vi "EC_Applied_XYZ_MM_BR_RES_2_NC_GR_pxi_Acc3_preset_LIM2.vi"() -> ()   [LabVIEW 2009]
uses:
  <vilib>/Utility/file.llb/Read From Spreadsheet File (I64).vi
  <vilib>/Utility/file.llb/Read From Spreadsheet File (string).vi
  <vilib>/Instr/_visa.llb/VISA Configure Serial Port (Instr).vi
  <vilib>/Utility/file.llb/Write To Spreadsheet File (I64).vi
  <vilib>/Utility/file.llb/Write To Spreadsheet File (string).vi
panel:
  out "R Velocity MVdeg/sec":dbl format="%.3f"
  out "R Position MV deg":dbl
  out "Z Velocity MV mm/sec":dbl format="%.3f"
  out "Z Position MV mm":dbl
  out "Y Velocity MV mm/sec":dbl format="%.3f"
  out "Y Position MV mm":dbl
  out "X Velocity MV mm/sec":dbl format="%.3f"
  out "X Position MV mm":dbl
  out "Presets":i32[][](array[numeric])
  in  "stop":bool
  in  "Tab Control 3":enum32{"Status", "Reset"}(tab)
  out "Y in Range":bool
  out "Y Scan":bool
  out "Y in Motion":bool
  out "Y Backlash corr":bool
  out "X  in Range":bool
  out "X Scan":bool
  out "X  in Motion":bool
  out "X Backlash corr":bool
  out "Z in Range":bool
  out "Z Scan":bool
  out "Z in Motion":bool
  out "Z Backlash corr":bool
  out "R in Range":bool
  out "R Scan":bool
  out "R in Motion":bool
  out "R Backlash corr":bool
  out "X Ready":bool
  out "Y Ready":bool
  out "Z Ready":bool
  out "R Ready":bool
  in  "Reset Y Position mm":dbl
  out "Reset Y Motor Steps":i32
  in  "Reset X Position mm":dbl
  out "Reset X Motor Steps":i32
  in  "Reset Z Position mm":dbl
  out "Reset Z Motor Steps":i32
  in  "Reset R Position deg":dbl
  out "Reset R Motor Steps":i32
  in  "Reset":bool
  in  "Tab Control 2":enum32{"mm", "step"}(tab)
  in  "X Scan Length SP mm":dbl
  in  "X Scan Velocity SP mm/sec":dbl
  in  "X Scan set":bool
  in  "Y Scan Length SP mm":dbl
  in  "Y Scan Velocity SP mm/sec":dbl
  in  "Y Scan set":bool
  in  "Z Scan Length SP mm":dbl
  in  "Z Scan Velocity SP mm/sec":dbl
  in  "Z Scan set":bool
  in  "R Scan Length SP deg":dbl
  in  "R Scan Velocity SP deg/sec":dbl
  in  "R Scan set":bool
  in  "X Scan Velocity SP steps/sec":i32=1 min=1 max=102400 step=1
  in  "X Scan Length SP steps":i32 min=-500000 max=500000 step=100
  out "X Scan length MV mm":dbl
  out "X Scan velocity MV mm/sec":dbl format="%#_6f"
  in  "Y Scan Velocity SP steps/sec":i32=1 min=1 max=102400 step=1
  in  "Y Scan Length SP steps":i32 min=-1000000 max=0 step=100
  out "Y Scan length MV mm":dbl
  out "Y Scan velocity MV mm/sec":dbl format="%#_6f"
  in  "Z Scan Velocity SP steps/sec":i32=1 min=1 max=102400 step=1
  in  "Z Scan Length SP steps":i32 min=-204724 max=102195276 step=100
  out "Z Scan length MV mm":dbl
  out "Z Scan velocity MV mm/sec":dbl format="%#_6f"
  in  "R Scan Velocity SP steps/sec":i32=1 min=1 max=102400 step=1
  in  "R Scan Length SP steps":i32 min=-6144000 max=0 step=100
  out "R Scan length MV deg":dbl
  out "R Scan velocity MV deg/sec":dbl format="%#_6f"
  out "atan Y/Z":dbl
  in  "Tab Control":enum32{"mm", "preset", "step"}(tab)
  in  "X Position SP mm":dbl
  in  "X Velocity SP mm/sec":dbl
  in  "X Move Set":bool
  in  "Y Move Set":bool
  in  "Y Position SP mm":dbl
  in  "Y Velocity SP mm/sec":dbl
  in  "Z Position SP mm":dbl
  in  "Z Velocity SP mm/sec":dbl
  in  "Z Move Set":bool
  in  "R Position SP deg":dbl
  in  "R Velocity SP deg/sec":dbl
  in  "R Move Set":bool
  in  "Add Button":bool
  in  "String":string
  in  "Delete Button":bool
  in  "Preset positions":i32(ring) items=["ZERO", "Default", "CDOSE", "QMS", "test", "test2", "test3"]
  in  "Set Button":bool
  in  "X Velocity SP step/sec":i32 min=1 max=50000
  in  "Y Velocity SP step/sec":i32 min=1 max=50000
  in  "Z Velocity SP step/sec":i32 min=1 max=5000
  in  "R Velocity SP step/sec":i32 min=1 max=10000
  in  "Y Step SP":i32=-20000 min=-800000 max=800000 step=500
  in  "X Step SP":i32=-20000 min=-800000 max=800000 step=500
  in  "Z Step SP":i32=-20000 min=0 max=102400000 step=500
  in  "R Step SP":i32=-20000 min=-6144000 max=0 step=500
  out "X Step PV":i32 max=2000
  out "Y Step PV":i32 max=2000
  out "Z Step PV":i32 max=2000
  out "R Step PV":i32 max=2000
  in  "Clear ZY":bool
  out "ZY Graph":cluster{"Y":dbl[], "Y":dbl[]}[](graph)
  out "ZR Graph":cluster{"Y":dbl[], "Y":dbl[]}[](graph)
  out "XY Graph":cluster{"Y":dbl[], "Y":dbl[]}[](graph)
  out "X Scan Duration":dbl
  out "Y Scan Duration":dbl
  out "Z Scan Duration":dbl
  out "R Scan Duration":dbl
  out "R Backlash steps/sec":i32
  out "R Backlash":i32
  out "R Holding Current %":i32
  out "R Run Current %":i32
  out "R offset deg":dbl
  out "R deg/rev":dbl
  out "R steps/rev":u32
  out "R velocity PV step/sec":i32
  out "R MINPOS":i32=-94296
  out "R MAXPOS":i32=-34296
  out "R COM PORT":refnum<visa-resource-name>="COM5"
  in  "R Scan OK":bool
  in  "R Go":bool
  out "R Position deg PV":dbl
  out "Z COM PORT":refnum<visa-resource-name>="COM5"
  out "Z Backlash steps/sec":i32
  out "Z Backlash":i32
  out "Z Holding Current %":i32
  out "Z Run Current %":i32
  out "Z offset mm":dbl
  out "Z mm/rev":dbl
  out "Z steps/rev":u32
  out "Z  velocity PV step/sec":i32
  out "Z MINPOS":i32=-94296
  out "Z MAXPOS":i32=-34296
  in  "Z Scan OK":bool
  in  "Z Go":bool
  out "Z Position mm PV":dbl
  out "X Position mm PV":dbl
  out "X velocity PV step/sec":i32
  in  "X Scan OK":bool
  in  "X Go":bool
  out "X Backlash steps/sec":i32
  out "X Backlash":i32
  out "X Holding Current %":i32
  out "X Run Current %":i32
  out "X offset mm":dbl
  out "X mm/rev":dbl
  out "X steps/rev":u32
  out "X MAXPOS":i32=-34296
  out "X MINPOS":i32=-94296
  out "X COM PORT":refnum<visa-resource-name>="COM5"
  out "Y Backlash steps/sec":i32
  out "Y Backlash":i32
  out "Y Holding Current %":i32
  out "Y Run Current %":i32
  in  "Scan Cancel":bool
  out "Y Position mm PV":dbl
  out "Y offset mm":dbl
  out "Y mm/rev":dbl
  out "Y steps/rev":u32
  out "Y velocity PV step/sec":i32
  in  "Y Scan OK":bool
  in  "Scan Go":bool
  in  "Stop":bool
  in  "Y Go":bool
  out "Y MINPOS":i32=-94296
  out "Y MAXPOS":i32=-34296
  out "Y COM PORT":refnum<visa-resource-name>="COM5"
  # "Current position"
  # "Goto position"
  # "RX"
  # "RY"
  # "RZ"
  # "RR"
  # "L"
  # "M"
  # "B"
  # "S"
  # "R"
  # "Preset position"
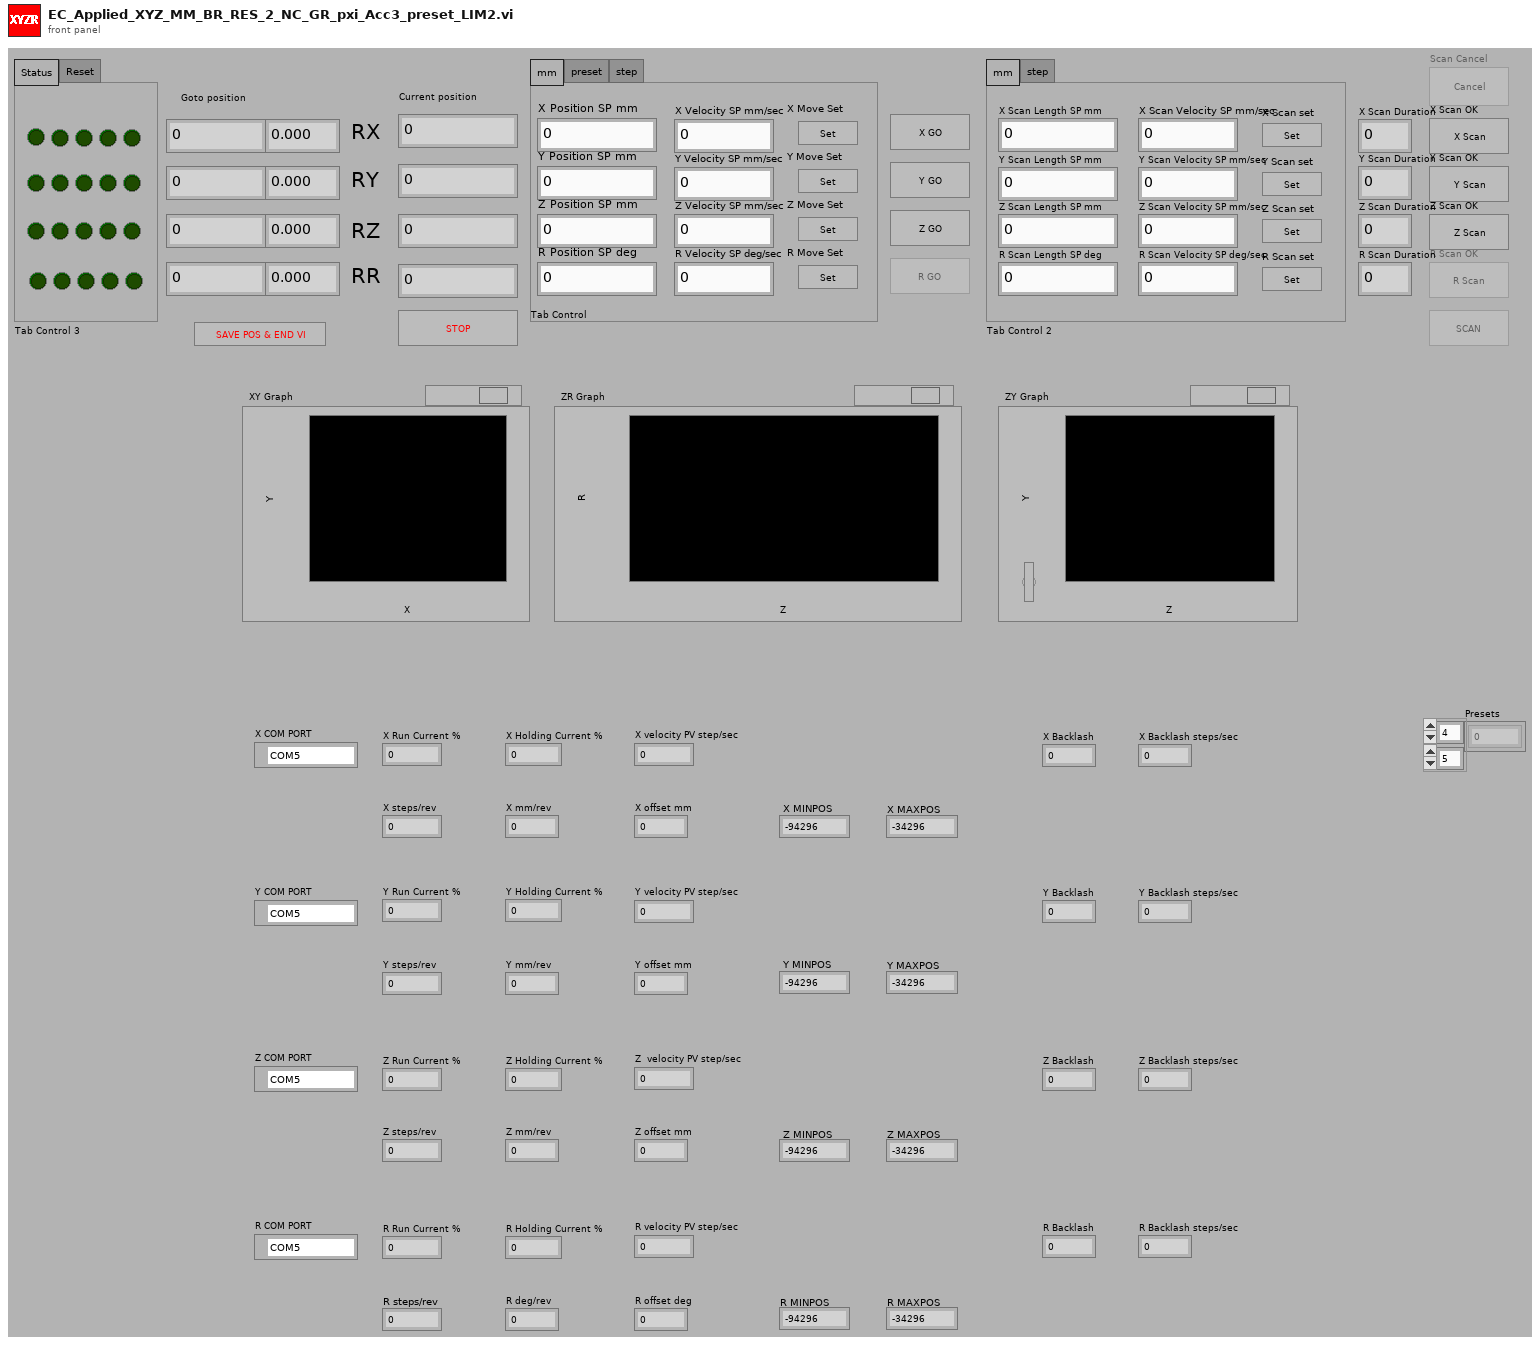
[diagram p1: front panel]
types:
  T1 = enum16{"Power-up Signature", "Accel Rate", "Accel Max", "Bit Rate", "Buffer Status", "Change Current", "Commence Jogging", "Change Jog Speed", "Continue", "Define Address", "Distance for FC,FM,FO,FY", "Decel Rate", "Distance or Position", "Define Limits", "Encoder Deadband", "Encoder Function", "Encoder Position", "Encoder Ratio", "Feed to Length with Speed Change", "Feed to Length", "Feed to Sensor with Mask Dist", "Feed to Length & Set Output", "Feed to Position", "Feed to Sensor", "Feed to Sensor w/safety", "Follow Handwheel", "Immediate Distance?", "Immediate Encoder?", "Immediate Low Output", "Immediate High Output", "Immediate Position?", "Input Status?", "Jog Accel/Decel", "Jog Disable", "Jog Enable", "Jog Speed", "Motor Disable", "Motor Enable", "Microstep Resolution", "Power up Current", "Power up Mode", "Pause", "Request Status", "Revision Level?", "Seek Home", "Stop Jogging", "Stop & Kill Buffer", "Set Output", "Set ABS Position", "Send String", "Stop", "Velocity for Speed Change", "Velocity Setting", "Wait for Input", "Wait Time"}
  T2 = enum8{"Enabled", "Disabled", "Disabled and Grayed Out"}
  T3 = cluster{"first row[0]":i64, "first row[1]":i64, "first row[2]":i64, "first row[3]":i64, "first row[4]":i64, "first row[5]":i64, "first row[6]":i64, "first row[7]":i64, "first row[8]":i64}
  T4 = cluster{"Value[0]":i32, "Value[1]":i32, "Value[2]":i32, "Value[3]":i32, "Value[4]":i32, "Value[5]":i32, "Value[6]":i32, "Value[7]":i32, "Value[8]":i32}
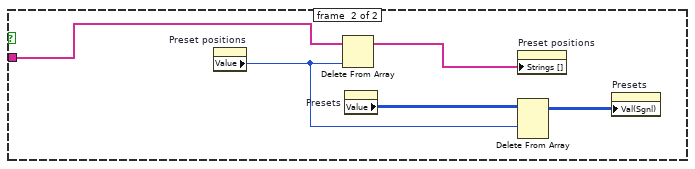
[diagram p2: hidden frame]
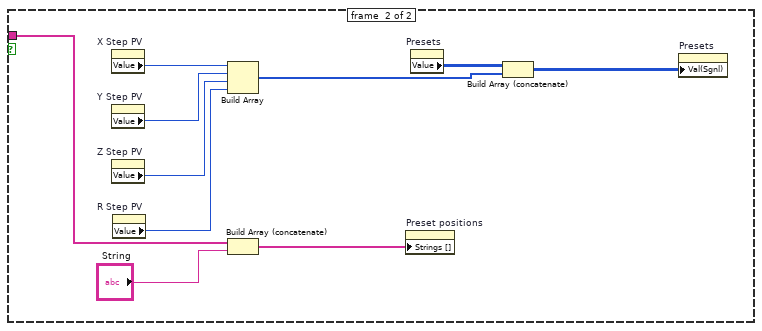
[diagram p3: hidden frame]
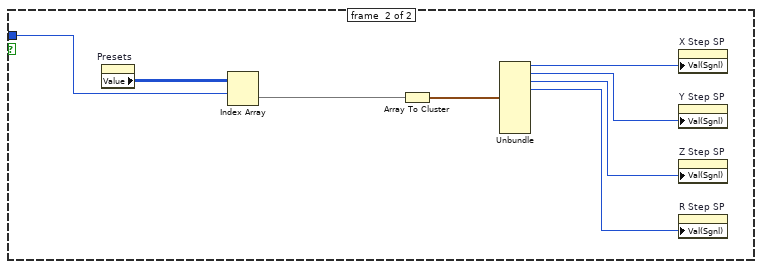
[diagram p4: hidden frame]
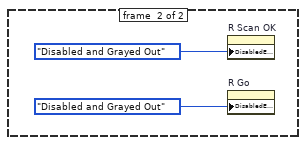
[diagram p5: hidden frame]
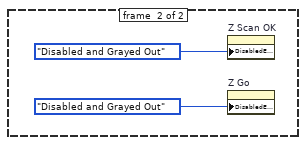
[diagram p8: hidden frame]
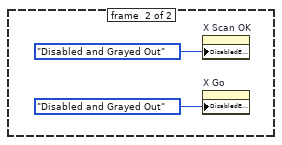
[diagram p11: hidden frame]
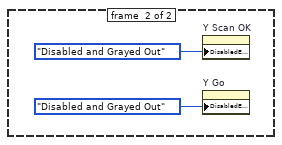
[diagram p14: hidden frame]
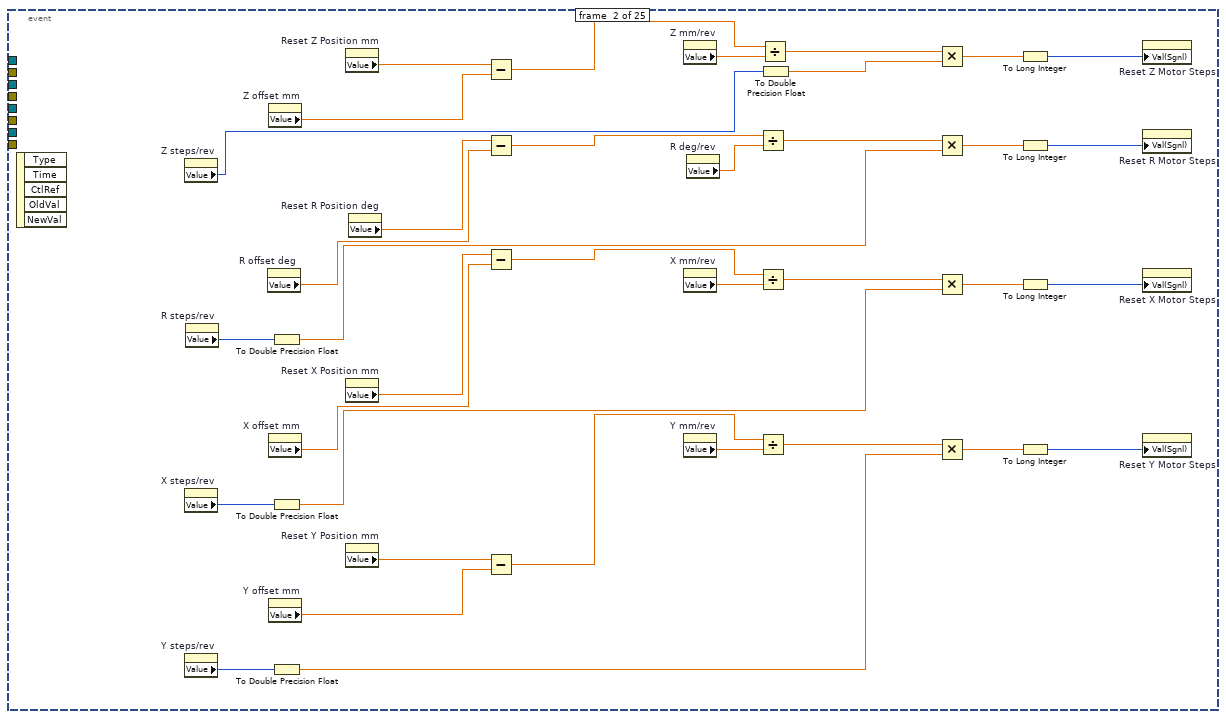
[diagram p17: hidden frame]
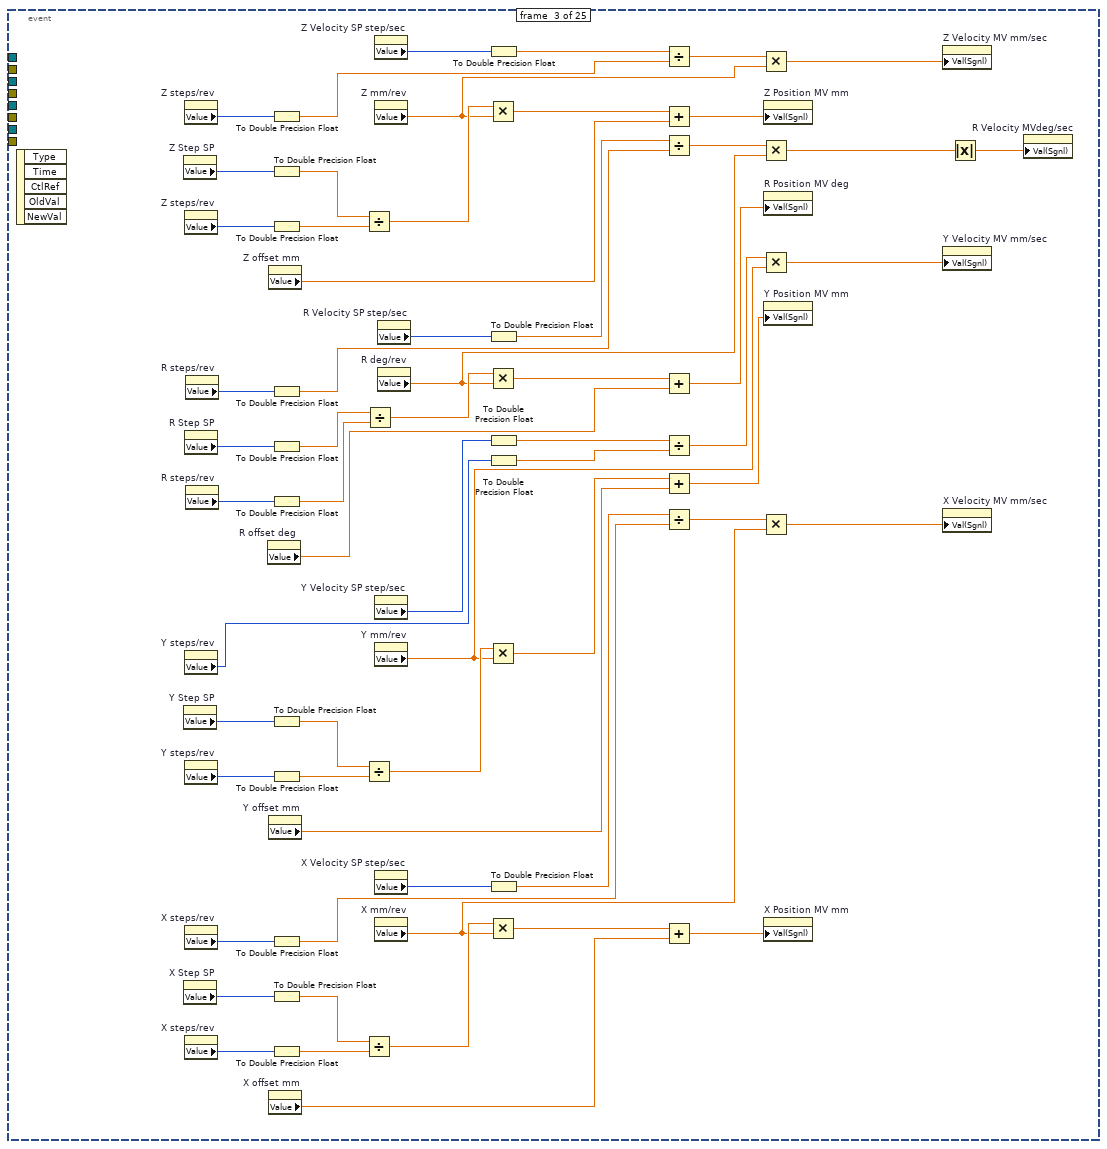
[diagram p18: hidden frame]
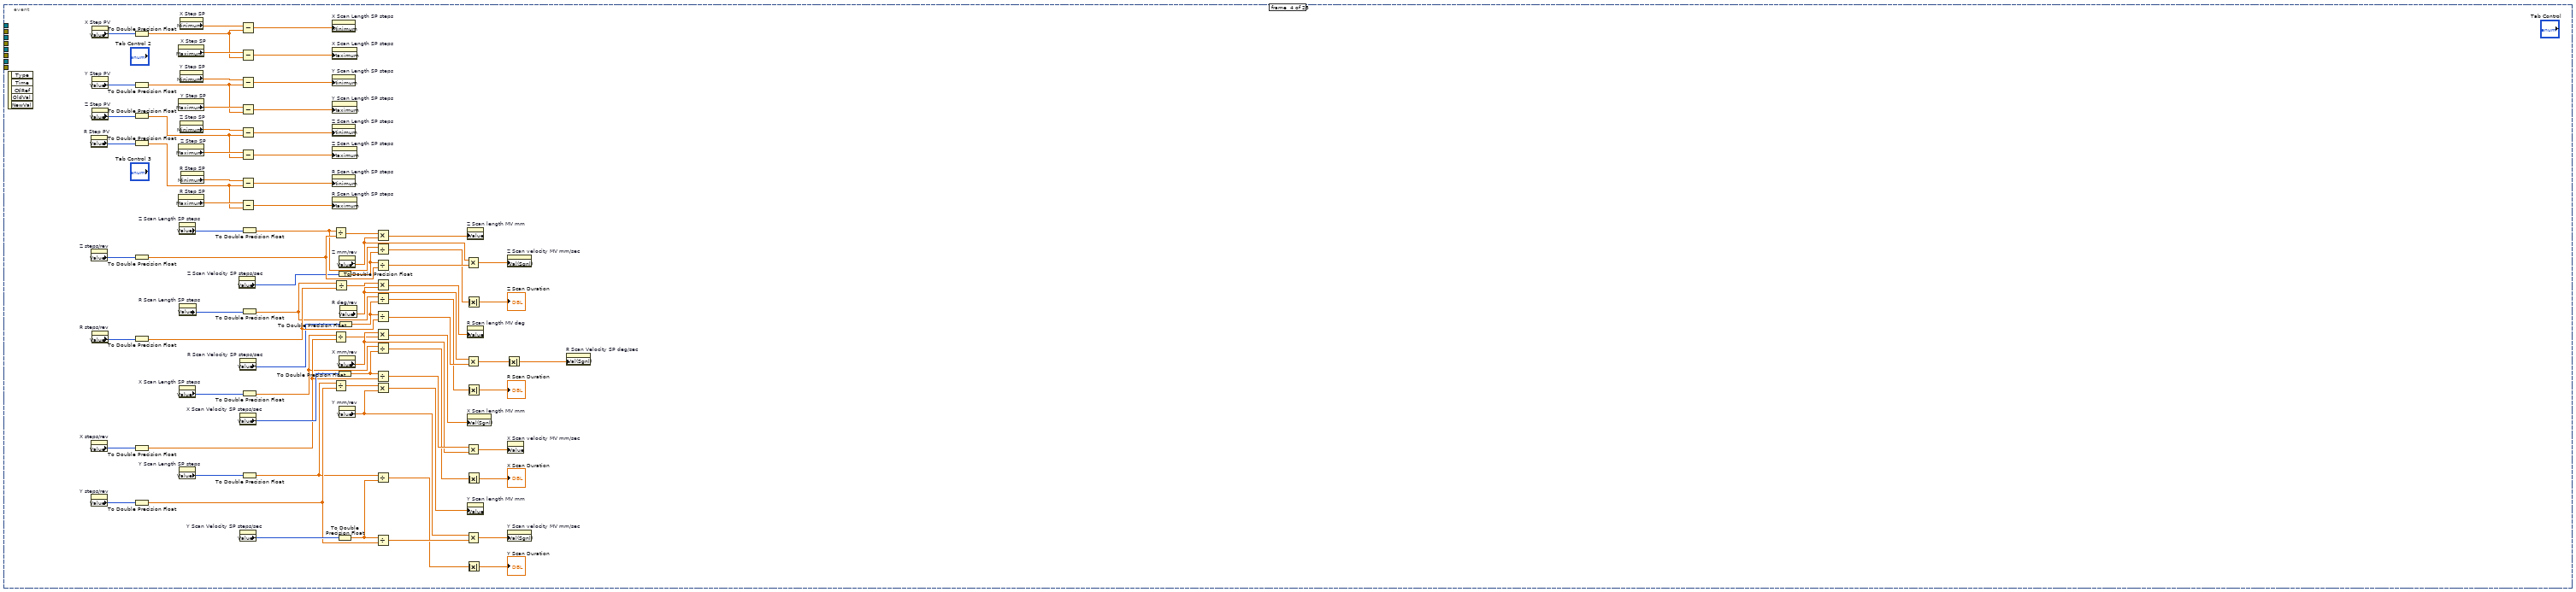
[diagram p19: hidden frame]
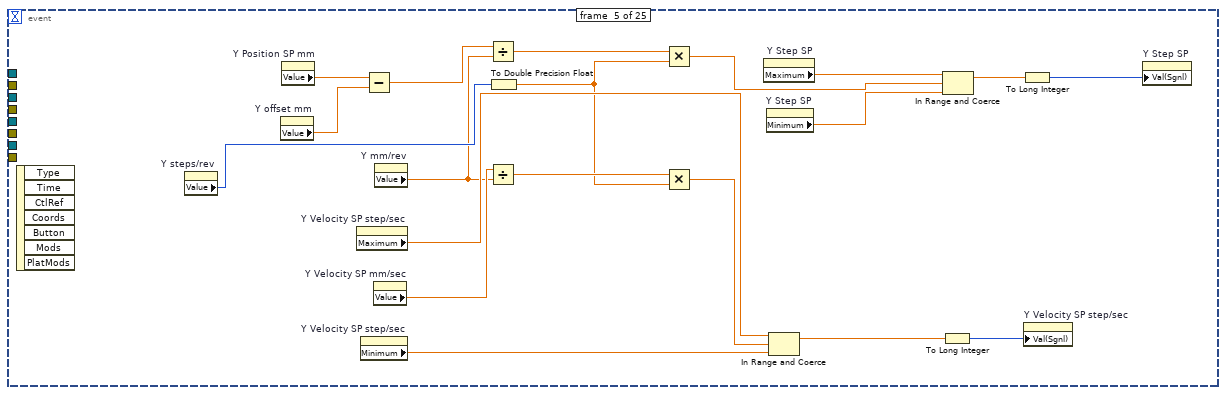
[diagram p20: hidden frame]
diagram:
  w24 = 0 ("dimension size")
  n1 = flat-sequence {
    tunnel: [w93] -> w10
    tunnel: [w92] -> w9
    tunnel: w10 -> [w107]
    tunnel: w9 -> [w106]
    tunnel: [w105] -> w8
    tunnel: [w104] -> w7
    tunnel: [w115] -> w64
    tunnel: [w114] -> w63
    tunnel: w8 -> [w117]
    tunnel: w7 -> [w116]
    tunnel: w64 -> [w132]
    tunnel: w63 -> [w131]
    tunnel: [w133] -> w62
    tunnel: [w134] -> w61
    tunnel: [w135] -> w6
    tunnel: [w146] -> w55
    tunnel: [w147] -> w56
    tunnel: w62 -> [w147]
    tunnel: w61 -> [w146]
    tunnel: w6 -> [w144]
    frame #0 {
      "Z Run Current %" <- 100 ("Z Run Current %")
      "Z Holding Current %" <- 50 ("Z Holding Current %")
    }
    frame #1 {
      "Z Backlash steps/sec" <- 1000 ("Z Backlash steps/sec")
      "Z Backlash" <- -5000 ("Z Backlash")
    }
    frame #2 {
      w83 = 2.54 ("Z mm/rev")
      w82 = u32 20000 ("step/rev")
      w84 = 5000 ("Value (Signaling)")
      n2 = property on="Z Scan Velocity SP mm/sec" class="DigNum (strict)"("Val(Sgnl)"=0.1 ("Value (Signaling)")) -> ()  [unwired: 2 in, 2 out]
      n3 = property on="Z Velocity SP step/sec" class="DigNum (strict)"("Val(Sgnl)"=w84) -> ()  [unwired: 2 in, 2 out]
      n4 = property on="Z Velocity SP step/sec" class="DigNum (strict)"("Minimum"=1.0 ("Data Entry Limits:Minimum")) -> ()  [unwired: 2 in, 2 out]
      n5 = To Double Precision Float(number=w84) -> (double precision float=w88:dbl)
      n6 = To Double Precision Float(number=w82) -> (double precision float=w87:dbl)
      n7 = property on="Z Velocity SP step/sec" class="DigNum (strict)"("Maximum"=w88) -> ()  [unwired: 2 in, 2 out]
      n8 = Divide(x=w88, y=w87) -> (x/y=w85:dbl)
      n9 = Multiply(x=w85, y=w83) -> (x*y=w86:dbl)
      n10 = property on="Z Velocity SP mm/sec" class="DigNum (strict)"("Val(Sgnl)"=w86) -> ()  [unwired: 2 in, 2 out]
      "Z mm/rev" <- w83
      "Z steps/rev" <- w82
    }
    frame #3 {
      w90 = 0 ("lower limit")
      w89 = 102400000 ("upper limit")
      n11 = property on="Z Step SP" class="DigNum (strict)"("Minimum"=w90) -> ()  [unwired: 2 in, 2 out]
      n12 = property on="Z Step SP" class="DigNum (strict)"("Maximum"=w89) -> ()  [unwired: 2 in, 2 out]
      "Z offset mm" <- 0.0 ("Z offset mm")
      "Z MINPOS" <- w90
      "Z MAXPOS" <- w89
    }
    frame #4 {
      w100 = refnum<visa-resource-name> "COM5" ("COM PORT")
      w98 = u16 0 items=["None", "XON/XOFF", "RTS/CTS", "XON/XOFF & RTS/CTS", "DTR/DSR", "XON/XOFF & DTR/DSR"] ("flow control (0:none)")
      w97 = u16 10 items=["1.0"=10, "1.5"=15, "2.0"=20] ("stop bits (10: 1 bit)")
      # "Stop bits"
      n13 = call-poly "VISA Configure Serial Port"("VISA resource name"=w100, "timeout (10sec)"=u32 10000, "baud rate (9600)"=u32 9600, "data bits (8)"=u16 8, "parity (0:none)"=enum16{"None", "Odd", "Even", "Mark", "Space"}."None", "stop bits (10: 1 bit)"=w97, "flow control (0:none)"=w98) -> ("VISA resource name out"=w93:refnum<visa-resource-name>, "error out"=w92:errorcluster)  [unwired: 7 in]
      "Z COM PORT" <- w100
    }
    frame #5 {
      # "Run Current %"
      n14 = property on="Z Run Current %" class="DigNum (strict)"() -> ("Value"=w108:i32)  [unwired: 2 in, 2 out]
      n15 = Divide(x=w108, y=100) -> (x/y=w109:dbl)
      n16 = Multiply(x=w109, y=3.5) -> (x*y=w103:dbl)
      n17 = Number To Fractional String(number=w103) -> (F-format string=w110:string)  [unwired: 3 in]
      n18 = call "Applied Send Command.vi"("error in (no error)"=w106, "Extra"=w110, "Command"=T1."Change Current", "VISA resource name"=w107) -> ("error out"=w104:errorcluster, "VISA resource name out"=w105:refnum<visa-resource-name>)  [unwired: 3 in, 1 out]
    }
    frame #6 {
      # "VELOCITY"
      n19 = property on="Z steps/rev" class="DigNum (strict)"() -> ("Value"=w113:u32)  [unwired: 2 in, 2 out]
      n20 = property on="Z Velocity SP step/sec" class="DigNum (strict)"() -> ("Value"=w112:i32)  [unwired: 2 in, 2 out]
      n21 = Divide(x=w112, y=w113) -> (x/y=w120:dbl)
      n22 = Number To Fractional String(number=w120) -> (F-format string=w122:string)  [unwired: 3 in]
      n23 = call "Applied Send Command.vi"("error in (no error)"=w116, "Extra"=w122, "Command"=T1."Velocity Setting", "VISA resource name"=w117) -> ("error out"=w123:errorcluster, "VISA resource name out"=w130:refnum<visa-resource-name>)  [unwired: 3 in, 1 out]
      n24 = call "Time Delay2"("error in (no error)"=w123, "Delay Time (s)"=0.1) -> ("error out"=w128:errorcluster)  [unwired: 9 in]
      n25 = call "Applied Send Command.vi"("error in (no error)"=w128, "Extra"="", "Command"=T1."Velocity Setting", "VISA resource name"=w130) -> ("error out"=w114:errorcluster, "read buffer"=w126:string, "VISA resource name out"=w115:refnum<visa-resource-name>)  [unwired: 3 in]
      n26 = Fract/Exp String To Number(string=w126, offset=3) -> (number=w121:dbl)  [unwired: 2 in, 1 out]
      n27 = Multiply(x=w121, y=w113) -> (x*y=w118:dbl)
      n28 = property on="Z  velocity PV step/sec" class="DigNum (strict)"("Val(Sgnl)"=w118) -> ()  [unwired: 2 in, 2 out]
    }
    frame #7 {
      # "GET CURRENT POSITION"
      n29 = call "Applied Send Command.vi"("error in (no error)"=w131, "Extra"="", "Command"=T1."Immediate Position?", "VISA resource name"=w132) -> ("error out"=w137:errorcluster, "read buffer"=w139:string, "VISA resource name out"=w133:refnum<visa-resource-name>)  [unwired: 3 in]
      n30 = call "Time Delay8"("error in (no error)"=w137, "Delay Time (s)"=0.1) -> ("error out"=w134:errorcluster)  [unwired: 9 in]
      n31 = Hexadecimal String To Number(string=w139, offset=3) -> (number=w135:u32)  [unwired: 1 in, 1 out]
    }
    frame #8 {
      n32 = property on="Z Step SP" class="DigNum (strict)"() -> ("Maximum"=w143:dbl)  [unwired: 2 in, 2 out]
      n33 = property on="Z Step SP" class="DigNum (strict)"("Val(Sgnl)"=w144) -> ()  [unwired: 2 in, 2 out]
      n34 = property on="Z Step SP" class="DigNum (strict)"() -> ("Minimum"=w142:dbl)  [unwired: 2 in, 2 out]
      n35 = In Range and Coerce(upper limit=w143, x=w144, lower limit=w142) -> (In Range?=w145:bool)  [unwired: 1 out]
      n36 = property on="Z in Range" class="Bool (strict)"("Val(Sgnl)"=w145) -> ()  [unwired: 2 in, 2 out]
    }
  }
  n37 = flat-sequence {
    tunnel: [w166] -> w3
    tunnel: [w165] -> w2
    tunnel: [w180] -> w5
    tunnel: [w179] -> w4
    tunnel: w3 -> [w178]
    tunnel: w2 -> [w177]
    tunnel: [w187] -> w60
    tunnel: [w188] -> w59
    tunnel: w5 -> [w185]
    tunnel: w4 -> [w186]
    tunnel: w60 -> [w205]
    tunnel: w59 -> [w204]
    tunnel: [w206] -> w58
    tunnel: [w208] -> w57
    tunnel: [w207] -> w1
    tunnel: [w219] -> w53
    tunnel: [w220] -> w54
    tunnel: w58 -> [w219]
    tunnel: w57 -> [w217]
    tunnel: w1 -> [w220]
    frame #0 {
      "R Run Current %" <- 100 ("R Run Current %")
      "R Holding Current %" <- 50 ("R Holding Current %")
    }
    frame #1 {
      "R Backlash" <- -12800 ("R Backlash")
      "R Backlash steps/sec" <- 6400 ("R Backlash steps/sec")
    }
    frame #2 {
      w156 = -3.0 ("R deg/rev")
      w158 = u32 20000 ("step/rev")
      w154 = 10000 ("Value (Signaling)")
      n38 = property on="R Velocity SP step/sec" class="DigNum (strict)"("Minimum"=1.0 ("Data Entry Limits:Minimum")) -> ()  [unwired: 2 in, 2 out]
      n39 = property on="R Velocity SP step/sec" class="DigNum (strict)"("Val(Sgnl)"=w154) -> ()  [unwired: 2 in, 2 out]
      n40 = property on="R Velocity SP deg/sec" class="DigNum (strict)"("Val(Sgnl)"=0.1 ("Value (Signaling)")) -> ()  [unwired: 2 in, 2 out]
      n41 = To Double Precision Float(number=w154) -> (double precision float=w152:dbl)
      n42 = To Double Precision Float(number=w158) -> (double precision float=w157:dbl)
      n43 = property on="R Velocity SP step/sec" class="DigNum (strict)"("Maximum"=w152) -> ()  [unwired: 2 in, 2 out]
      n44 = Divide(x=w152, y=w157) -> (x/y=w153:dbl)
      n45 = Multiply(x=w153, y=w156) -> (x*y=w155:dbl)
      n46 = Absolute Value(x=w155) -> (abs(x)=w160:dbl)
      n47 = property on="R Velocity SP deg/sec" class="DigNum (strict)"("Val(Sgnl)"=w160) -> ()  [unwired: 2 in, 2 out]
      "R deg/rev" <- w156
      "R steps/rev" <- w158
    }
    frame #3 {
      w163 = 0 ("upper limit")
      w164 = -6144000 ("lower limit")
      n48 = property on="R Step SP" class="DigNum (strict)"("Minimum"=w164) -> ()  [unwired: 2 in, 2 out]
      n49 = property on="R Step SP" class="DigNum (strict)"("Maximum"=w163) -> ()  [unwired: 2 in, 2 out]
      "R MINPOS" <- w163
      "R MAXPOS" <- w164
      "R offset deg" <- 0.0 ("R offset deg")
    }
    frame #4 {
      w173 = refnum<visa-resource-name> "COM6" ("COM PORT")
      w171 = u16 0 items=["None", "XON/XOFF", "RTS/CTS", "XON/XOFF & RTS/CTS", "DTR/DSR", "XON/XOFF & DTR/DSR"] ("flow control (0:none)")
      w170 = u16 10 items=["1.0"=10, "1.5"=15, "2.0"=20] ("stop bits (10: 1 bit)")
      # "Stop bits"
      n50 = call-poly "VISA Configure Serial Port"("VISA resource name"=w173, "timeout (10sec)"=u32 10000, "baud rate (9600)"=u32 9600, "data bits (8)"=u16 8, "parity (0:none)"=enum16{"None", "Odd", "Even", "Mark", "Space"}."None", "stop bits (10: 1 bit)"=w170, "flow control (0:none)"=w171) -> ("VISA resource name out"=w166:refnum<visa-resource-name>, "error out"=w165:errorcluster)  [unwired: 7 in]
      "R COM PORT" <- w173
    }
    frame #5 {
      # "Run Current %"
      n51 = property on="R Run Current %" class="DigNum (strict)"() -> ("Value"=w181:i32)  [unwired: 2 in, 2 out]
      n52 = Divide(x=w181, y=100) -> (x/y=w182:dbl)
      n53 = Multiply(x=w182, y=3.5) -> (x*y=w176:dbl)
      n54 = Number To Fractional String(number=w176) -> (F-format string=w183:string)  [unwired: 3 in]
      n55 = call "Applied Send Command.vi"("error in (no error)"=w177, "Extra"=w183, "Command"=T1."Change Current", "VISA resource name"=w178) -> ("error out"=w179:errorcluster, "VISA resource name out"=w180:refnum<visa-resource-name>)  [unwired: 3 in, 1 out]
    }
    frame #6 {
      # "VELOCITY"
      n56 = property on="R steps/rev" class="DigNum (strict)"() -> ("Value"=w191:u32)  [unwired: 2 in, 2 out]
      n57 = property on="R Velocity SP step/sec" class="DigNum (strict)"() -> ("Value"=w189:i32)  [unwired: 2 in, 2 out]
      n58 = Divide(x=w189, y=w191) -> (x/y=w193:dbl)
      n59 = Number To Fractional String(number=w193) -> (F-format string=w195:string)  [unwired: 3 in]
      n60 = call "Applied Send Command.vi"("error in (no error)"=w186, "Extra"=w195, "Command"=T1."Velocity Setting", "VISA resource name"=w185) -> ("error out"=w196:errorcluster, "VISA resource name out"=w203:refnum<visa-resource-name>)  [unwired: 3 in, 1 out]
      n61 = call "Time Delay43"("error in (no error)"=w196, "Delay Time (s)"=0.1) -> ("error out"=w201:errorcluster)  [unwired: 9 in]
      n62 = call "Applied Send Command.vi"("error in (no error)"=w201, "Extra"="", "Command"=T1."Velocity Setting", "VISA resource name"=w203) -> ("error out"=w188:errorcluster, "read buffer"=w199:string, "VISA resource name out"=w187:refnum<visa-resource-name>)  [unwired: 3 in]
      n63 = Fract/Exp String To Number(string=w199, offset=3) -> (number=w194:dbl)  [unwired: 2 in, 1 out]
      n64 = Multiply(x=w194, y=w191) -> (x*y=w190:dbl)
      n65 = property on="R velocity PV step/sec" class="DigNum (strict)"("Val(Sgnl)"=w190) -> ()  [unwired: 2 in, 2 out]
    }
    frame #7 {
      # "GET CURRENT POSITION"
      n66 = call "Applied Send Command.vi"("error in (no error)"=w204, "Extra"="", "Command"=T1."Immediate Position?", "VISA resource name"=w205) -> ("error out"=w210:errorcluster, "read buffer"=w212:string, "VISA resource name out"=w207:refnum<visa-resource-name>)  [unwired: 3 in]
      n67 = call "Time Delay42"("error in (no error)"=w210, "Delay Time (s)"=0.1) -> ("error out"=w206:errorcluster)  [unwired: 9 in]
      n68 = Hexadecimal String To Number(string=w212, offset=3) -> (number=w208:u32)  [unwired: 1 in, 1 out]
    }
    frame #8 {
      n69 = property on="R Step SP" class="DigNum (strict)"() -> ("Maximum"=w215:dbl)  [unwired: 2 in, 2 out]
      n70 = property on="R Step SP" class="DigNum (strict)"("Val(Sgnl)"=w217) -> ()  [unwired: 2 in, 2 out]
      n71 = property on="R Step SP" class="DigNum (strict)"() -> ("Minimum"=w216:dbl)  [unwired: 2 in, 2 out]
      n72 = In Range and Coerce(upper limit=w215, x=w217, lower limit=w216) -> (In Range?=w218:bool)  [unwired: 1 out]
      n73 = property on="R in Range" class="Bool (strict)"("Val(Sgnl)"=w218) -> ()  [unwired: 2 in, 2 out]
    }
  }
  n74 = flat-sequence {
    frame #0 {
      n75 = property on="X Scan" class="Bool (strict)"("Val(Sgnl)"=FALSE ("Value (Signaling)")) -> ()  [unwired: 2 in, 2 out]
      n76 = property on="Y Scan" class="Bool (strict)"("Val(Sgnl)"=FALSE ("Value (Signaling)")) -> ()  [unwired: 2 in, 2 out]
      n77 = property on="Z Scan" class="Bool (strict)"("Val(Sgnl)"=FALSE ("Value (Signaling)")) -> ()  [unwired: 2 in, 2 out]
      n78 = property on="R Scan" class="Bool (strict)"("Val(Sgnl)"=FALSE ("Value (Signaling)")) -> ()  [unwired: 2 in, 2 out]
      n79 = property on="Scan Go" class="Bool"("DisabledEnum"=T2."Disabled and Grayed Out" ("Disabled")) -> ()  [unwired: 2 in, 2 out]
      n80 = property on="Scan Cancel" class="Bool"("DisabledEnum"=T2."Disabled and Grayed Out" ("Disabled")) -> ()  [unwired: 2 in, 2 out]
    }
    frame #1 {
      n81 = property on="Y Backlash corr" class="Bool (strict)"("Val(Sgnl)"=FALSE ("Value (Signaling)")) -> ()  [unwired: 2 in, 2 out]
      n82 = property on="R Backlash corr" class="Bool (strict)"("Val(Sgnl)"=FALSE ("Value (Signaling)")) -> ()  [unwired: 2 in, 2 out]
      n83 = property on="X Backlash corr" class="Bool (strict)"("Val(Sgnl)"=FALSE ("Value (Signaling)")) -> ()  [unwired: 2 in, 2 out]
      n84 = property on="Z Backlash corr" class="Bool (strict)"("Val(Sgnl)"=FALSE ("Value (Signaling)")) -> ()  [unwired: 2 in, 2 out]
    }
  }
  n85 = flat-sequence {
    tunnel: [w248] -> w18
    tunnel: [w247] -> w17
    tunnel: w18 -> [w262]
    tunnel: w17 -> [w261]
    tunnel: [w260] -> w16
    tunnel: [w259] -> w15
    tunnel: w16 -> [w270]
    tunnel: w15 -> [w269]
    tunnel: [w268] -> w14
    tunnel: [w267] -> w13
    tunnel: [w287] -> w68
    tunnel: w14 -> [w290]
    tunnel: w13 -> [w289]
    tunnel: [w288] -> w12
    tunnel: [w286] -> w11
    tunnel: [w299] -> w74
    tunnel: [w302] -> w75
    tunnel: w68 -> [w299]
    tunnel: w12 -> [w302]
    tunnel: w11 -> [w300]
    frame #0 {
      "Y Run Current %" <- 100 ("Run Current %")
      "Y Holding Current %" <- 50 ("Holding Current %")
    }
    frame #1 {
      "Y Backlash" <- 5000 ("Backlash2")
      "Y Backlash steps/sec" <- 10000 ("Value (Signaling)")
    }
    frame #2 {
      w238 = 0.21167 ("MM/rev")
      w241 = u32 20000 ("step/rev")
      w236 = 50000 ("Value (Signaling)")
      n86 = property on="Y Velocity SP step/sec" class="DigNum (strict)"("Minimum"=1.0 ("Data Entry Limits:Minimum")) -> ()  [unwired: 2 in, 2 out]
      n87 = property on="Y Scan Velocity SP mm/sec" class="DigNum (strict)"("Val(Sgnl)"=0.1 ("Value (Signaling)")) -> ()  [unwired: 2 in, 2 out]
      n88 = property on="Y Velocity SP step/sec" class="DigNum (strict)"("Val(Sgnl)"=w236) -> ()  [unwired: 2 in, 2 out]
      n89 = To Double Precision Float(number=w236) -> (double precision float=w242:dbl)
      n90 = To Double Precision Float(number=w241) -> (double precision float=w240:dbl)
      n91 = property on="Y Velocity SP step/sec" class="DigNum (strict)"("Maximum"=w242) -> ()  [unwired: 2 in, 2 out]
      n92 = Divide(x=w242, y=w240) -> (x/y=w237:dbl)
      n93 = Multiply(x=w237, y=w238) -> (x*y=w239:dbl)
      n94 = property on="Y Velocity SP mm/sec" class="DigNum (strict)"("Val(Sgnl)"=w239) -> ()  [unwired: 2 in, 2 out]
      "Y steps/rev" <- w241
      "Y mm/rev" <- w238
    }
    frame #3 {
      w245 = -750000 ("lower limit")
      w246 = 750000 ("upper limit")
      n95 = property on="Y Step SP" class="DigNum (strict)"("Minimum"=w245) -> ()  [unwired: 2 in, 2 out]
      n96 = property on="Y Step SP" class="DigNum (strict)"("Maximum"=w246) -> ()  [unwired: 2 in, 2 out]
      "Y MAXPOS" <- w246
      "Y MINPOS" <- w245
      "Y offset mm" <- 0.0 ("offset")
    }
    frame #4 {
      w255 = refnum<visa-resource-name> "COM4" ("COM PORT")
      w253 = u16 0 items=["None", "XON/XOFF", "RTS/CTS", "XON/XOFF & RTS/CTS", "DTR/DSR", "XON/XOFF & DTR/DSR"] ("flow control (0:none)")
      w252 = u16 10 items=["1.0"=10, "1.5"=15, "2.0"=20] ("stop bits (10: 1 bit)")
      # "Stop bits"
      n97 = call-poly "VISA Configure Serial Port"("VISA resource name"=w255, "timeout (10sec)"=u32 10000, "baud rate (9600)"=u32 9600, "data bits (8)"=u16 8, "parity (0:none)"=enum16{"None", "Odd", "Even", "Mark", "Space"}."None", "stop bits (10: 1 bit)"=w252, "flow control (0:none)"=w253) -> ("VISA resource name out"=w248:refnum<visa-resource-name>, "error out"=w247:errorcluster)  [unwired: 7 in]
      "Y COM PORT" <- w255
    }
    frame #5 {
      n98 = property on="Y Run Current %" class="DigNum (strict)"() -> ("Value"=w263:i32)  [unwired: 2 in, 2 out]
      n99 = Divide(x=w263, y=100) -> (x/y=w264:dbl)
      n100 = Multiply(x=w264, y=3.5) -> (x*y=w258:dbl)
      n101 = Number To Fractional String(number=w258) -> (F-format string=w265:string)  [unwired: 3 in]
      n102 = call "Applied Send Command.vi"("error in (no error)"=w261, "Extra"=w265, "Command"=T1."Change Current", "VISA resource name"=w262) -> ("error out"=w259:errorcluster, "VISA resource name out"=w260:refnum<visa-resource-name>)  [unwired: 3 in, 1 out]
    }
    frame #6 {
      # "VELOCITY"
      n103 = property on="Y steps/rev" class="DigNum (strict)"() -> ("Value"=w274:u32)  [unwired: 2 in, 2 out]
      n104 = property on="Y Velocity SP step/sec" class="DigNum (strict)"() -> ("Value"=w271:i32)  [unwired: 2 in, 2 out]
      n105 = Divide(x=w271, y=w274) -> (x/y=w273:dbl)
      n106 = Number To Fractional String(number=w273) -> (F-format string=w277:string)  [unwired: 3 in]
      n107 = call "Applied Send Command.vi"("error in (no error)"=w269, "Extra"=w277, "Command"=T1."Velocity Setting", "VISA resource name"=w270) -> ("error out"=w278:errorcluster, "VISA resource name out"=w285:refnum<visa-resource-name>)  [unwired: 3 in, 1 out]
      n108 = call "Time Delay36"("error in (no error)"=w278, "Delay Time (s)"=0.1) -> ("error out"=w283:errorcluster)  [unwired: 9 in]
      n109 = call "Applied Send Command.vi"("error in (no error)"=w283, "Extra"="", "Command"=T1."Velocity Setting", "VISA resource name"=w285) -> ("error out"=w267:errorcluster, "read buffer"=w281:string, "VISA resource name out"=w268:refnum<visa-resource-name>)  [unwired: 3 in]
      n110 = Fract/Exp String To Number(string=w281, offset=3) -> (number=w276:dbl)  [unwired: 2 in, 1 out]
      n111 = Multiply(x=w276, y=w274) -> (x*y=w275:dbl)
      n112 = property on="Y velocity PV step/sec" class="DigNum (strict)"("Val(Sgnl)"=w275) -> ()  [unwired: 2 in, 2 out]
    }
    frame #7 {
      # "GET CURRENT POSITION"
      n113 = call "Applied Send Command.vi"("error in (no error)"=w289, "Extra"="", "Command"=T1."Immediate Position?", "VISA resource name"=w290) -> ("error out"=w292:errorcluster, "read buffer"=w294:string, "VISA resource name out"=w288:refnum<visa-resource-name>)  [unwired: 3 in]
      n114 = call "Time Delay37"("error in (no error)"=w292, "Delay Time (s)"=0.1) -> ("error out"=w287:errorcluster)  [unwired: 9 in]
      n115 = Hexadecimal String To Number(string=w294, offset=3) -> (number=w286:u32)  [unwired: 1 in, 1 out]
    }
    frame #8 {
      n116 = property on="Y Step SP" class="DigNum (strict)"() -> ("Maximum"=w298:dbl)  [unwired: 2 in, 2 out]
      n117 = property on="Y Step SP" class="DigNum (strict)"("Val(Sgnl)"=w300) -> ()  [unwired: 2 in, 2 out]
      n118 = property on="Y Step SP" class="DigNum (strict)"() -> ("Minimum"=w297:dbl)  [unwired: 2 in, 2 out]
      n119 = In Range and Coerce(upper limit=w298, x=w300, lower limit=w297) -> (In Range?=w301:bool)  [unwired: 1 out]
      n120 = property on="Y in Range" class="Bool (strict)"("Val(Sgnl)"=w301) -> ()  [unwired: 2 in, 2 out]
    }
  }
  n121 = flat-sequence {
    tunnel: [w320] -> w23
    tunnel: [w319] -> w22
    tunnel: w23 -> [w337]
    tunnel: w22 -> [w336]
    tunnel: [w335] -> w21
    tunnel: [w334] -> w20
    tunnel: [w340] -> w73
    tunnel: w21 -> [w348]
    tunnel: w20 -> [w347]
    tunnel: [w341] -> w19
    tunnel: w73 -> [w362]
    tunnel: [w361] -> w67
    tunnel: [w359] -> w66
    tunnel: [w364] -> w65
    tunnel: w19 -> [w363]
    tunnel: [w373] -> w71
    tunnel: [w374] -> w72
    tunnel: w67 -> [w374]
    tunnel: w66 -> [w373]
    tunnel: w65 -> [w369]
    frame #0 {
      "X Run Current %" <- 100 ("Run Current %")
      "X Holding Current %" <- 50 ("Holding Current %")
    }
    frame #1 {
      "X Backlash steps/sec" <- 10000 ("Value (Signaling)")
      "X Backlash" <- 5000 ("Backlash2")
    }
    frame #2 {
      w309 = 0.21167 ("MM/rev")
      w312 = u32 20000 ("step/rev")
      w307 = 50000 ("Value (Signaling)")
      n122 = property on="X Velocity SP step/sec" class="DigNum (strict)"("Minimum"=1.0 ("Data Entry Limits:Minimum")) -> ()  [unwired: 2 in, 2 out]
      n123 = property on="X Velocity SP step/sec" class="DigNum (strict)"("Val(Sgnl)"=w307) -> ()  [unwired: 2 in, 2 out]
      n124 = property on="X Scan Velocity SP mm/sec" class="DigNum (strict)"("Val(Sgnl)"=0.1 ("Value (Signaling)")) -> ()  [unwired: 2 in, 2 out]
      n125 = To Double Precision Float(number=w307) -> (double precision float=w313:dbl)
      n126 = To Double Precision Float(number=w312) -> (double precision float=w311:dbl)
      n127 = property on="X Velocity SP step/sec" class="DigNum (strict)"("Maximum"=w313) -> ()  [unwired: 2 in, 2 out]
      n128 = Divide(x=w313, y=w311) -> (x/y=w308:dbl)
      n129 = Multiply(x=w308, y=w309) -> (x*y=w310:dbl)
      n130 = property on="X Velocity SP mm/sec" class="DigNum (strict)"("Val(Sgnl)"=w310) -> ()  [unwired: 2 in, 2 out]
      "X steps/rev" <- w312
      "X mm/rev" <- w309
    }
    frame #3 {
      w318 = -750000 ("lower limit")
      w317 = 750000 ("upper limit")
      n131 = property on="X Step SP" class="DigNum (strict)"("Minimum"=w318) -> ()  [unwired: 2 in, 2 out]
      n132 = property on="X Step SP" class="DigNum (strict)"("Maximum"=w317) -> ()  [unwired: 2 in, 2 out]
      "X offset mm" <- 0.0 ("offset")
      "X MAXPOS" <- w317
      "X MINPOS" <- w318
    }
    frame #4 {
      w327 = refnum<visa-resource-name> "COM3" ("COM PORT")
      w325 = u16 0 items=["None", "XON/XOFF", "RTS/CTS", "XON/XOFF & RTS/CTS", "DTR/DSR", "XON/XOFF & DTR/DSR"] ("flow control (0:none)")
      w324 = u16 10 items=["1.0"=10, "1.5"=15, "2.0"=20] ("stop bits (10: 1 bit)")
      # "Stop bits"
      n133 = call-poly "VISA Configure Serial Port"("VISA resource name"=w327, "timeout (10sec)"=u32 10000, "baud rate (9600)"=u32 9600, "data bits (8)"=u16 8, "parity (0:none)"=enum16{"None", "Odd", "Even", "Mark", "Space"}."None", "stop bits (10: 1 bit)"=w324, "flow control (0:none)"=w325) -> ("VISA resource name out"=w320:refnum<visa-resource-name>, "error out"=w319:errorcluster)  [unwired: 7 in]
      "X COM PORT" <- w327
    }
    frame #5 {
      n134 = property on="X Run Current" class="DigNum (strict)"() -> ("Value"=w332:i32)  [unwired: 2 in, 2 out]
      n135 = Divide(x=w332, y=100) -> (x/y=w329:dbl)
      n136 = Multiply(x=3.5 ("y"), y=w329) -> (x*y=w331:dbl)
      n137 = Number To Fractional String(number=w331) -> (F-format string=w333:string)  [unwired: 3 in]
      n138 = call "Applied Send Command.vi"("error in (no error)"=w336, "Extra"=w333, "Command"=T1."Change Current", "VISA resource name"=w337) -> ("error out"=w335:errorcluster, "VISA resource name out"=w334:refnum<visa-resource-name>)  [unwired: 3 in, 1 out]
    }
    frame #6 {
      # "VELOCITY"
      n139 = property on="X steps/rev" class="DigNum (strict)"() -> ("Value"=w343:u32)  [unwired: 2 in, 2 out]
      n140 = property on="X Velocity SP step/sec" class="DigNum (strict)"() -> ("Value"=w344:i32)  [unwired: 2 in, 2 out]
      n141 = Divide(x=w344, y=w343) -> (x/y=w342:dbl)
      n142 = Number To Fractional String(number=w342) -> (F-format string=w349:string)  [unwired: 3 in]
      n143 = call "Applied Send Command.vi"("error in (no error)"=w348, "Extra"=w349, "Command"=T1."Velocity Setting", "VISA resource name"=w347) -> ("error out"=w350:errorcluster, "VISA resource name out"=w357:refnum<visa-resource-name>)  [unwired: 3 in, 1 out]
      n144 = call "Time Delay30"("error in (no error)"=w350, "Delay Time (s)"=0.1) -> ("error out"=w355:errorcluster)  [unwired: 9 in]
      n145 = call "Applied Send Command.vi"("error in (no error)"=w355, "Extra"="", "Command"=T1."Velocity Setting", "VISA resource name"=w357) -> ("error out"=w340:errorcluster, "read buffer"=w353:string, "VISA resource name out"=w341:refnum<visa-resource-name>)  [unwired: 3 in]
      n146 = Fract/Exp String To Number(string=w353, offset=3) -> (number=w346:dbl)  [unwired: 2 in, 1 out]
      n147 = Multiply(x=w346, y=w343) -> (x*y=w345:dbl)
      n148 = property on="X velocity PV step/sec" class="DigNum (strict)"("Val(Sgnl)"=w345) -> ()  [unwired: 2 in, 2 out]
    }
    frame #7 {
      # "GET CURRENT POSITION"
      n149 = call "Applied Send Command.vi"("error in (no error)"=w362, "Extra"="", "Command"=T1."Immediate Position?", "VISA resource name"=w363) -> ("error out"=w360:errorcluster, "read buffer"=w366:string, "VISA resource name out"=w361:refnum<visa-resource-name>)  [unwired: 3 in]
      n150 = call "Time Delay13"("error in (no error)"=w360, "Delay Time (s)"=0.1) -> ("error out"=w359:errorcluster)  [unwired: 9 in]
      n151 = Hexadecimal String To Number(string=w366, offset=3) -> (number=w364:u32)  [unwired: 1 in, 1 out]
    }
    frame #8 {
      n152 = property on="X Step SP" class="DigNum (strict)"() -> ("Maximum"=w372:dbl)  [unwired: 2 in, 2 out]
      n153 = property on="X Step SP" class="DigNum (strict)"("Val(Sgnl)"=w369) -> ()  [unwired: 2 in, 2 out]
      n154 = property on="X Step SP" class="DigNum (strict)"() -> ("Minimum"=w371:dbl)  [unwired: 2 in, 2 out]
      n155 = In Range and Coerce(upper limit=w372, x=w369, lower limit=w371) -> (In Range?=w370:bool)  [unwired: 1 out]
      n156 = property on="X  in Range" class="Bool (strict)"("Val(Sgnl)"=w370) -> ()  [unwired: 2 in, 2 out]
    }
  }
  n157 = call-poly <vilib>:"Read From Spreadsheet File.vi"("file path (dialog if empty)"=path "S:/LV codes/SCL2/POS.TXT") -> ("first row"=w42:i64[])  [unwired: 6 in, 4 out]
  n158 = call-poly <vilib>:"Read From Spreadsheet File.vi"("file path (dialog if empty)"=path "S:/LV codes/SCL2/PRESET.TXT") -> ("all rows"=w30:string[][])  [unwired: 6 in, 4 out]
  n159 = Array To Cluster(array=w42) -> (cluster=w41:T3)
  n160 = Transpose 2D Array(2D array=w30) -> (transposed array=w31:string[][])
  n161 = Unbundle(w41) -> ("first row[0]"=w39:i64, "first row[1]"=w38:i64, "first row[2]"=w37:i64, "first row[3]"=w36:i64)  [unwired: 5 out]
  n162 = Delete From Array(array=w31, index (row)=0) -> (deleted portion=w32:string[], array with subset deleted=w34:string[][])  [unwired: 2 in]
  n163 = property on="Reset X Motor Steps" class="DigNum (strict)"("Val(Sgnl)"=w39) -> ()  [unwired: 2 in, 2 out]
  n164 = property on="Reset Y Motor Steps" class="DigNum (strict)"("Val(Sgnl)"=w38) -> ()  [unwired: 2 in, 2 out]
  n165 = property on="Reset Z Motor Steps" class="DigNum (strict)"("Val(Sgnl)"=w37) -> ()  [unwired: 2 in, 2 out]
  n166 = property on="Reset R Motor Steps" class="DigNum (strict)"("Val(Sgnl)"=w36) -> ()  [unwired: 2 in, 2 out]
  n167 = Transpose 2D Array(2D array=w34) -> (transposed array=w35:string[][])
  n168 = property on="Preset positions" class="Ring (strict)"("Strings []"=w32) -> ()  [unwired: 2 in, 2 out]
  n169 = Decimal String To Number(string=w35) -> (number=w33:i32[][])  [unwired: 2 in, 1 out]
  n170 = Initialize Array(w24, w24, 4 ("dimension size")) -> (w27:i32[][])
  n171 = Build Array (concatenate)(w27, w33) -> (→"Presets":i32[][])
  n172 = while {
    tunnel: w75 -> [w393]
    tunnel: w74 -> [w396]
    tunnel: [w397] -> w49
    tunnel: [w395] -> w50
    tunnel: w72 -> [w392]
    tunnel: w71 -> [w391]
    tunnel: [w390] -> w70
    tunnel: [w389] -> w69
    tunnel: w56 -> [w388]
    tunnel: w55 -> [w387]
    tunnel: [w386] -> w52
    tunnel: [w385] -> w51
    tunnel: w54 -> [w384]
    tunnel: w53 -> [w383]
    tunnel: [w382] -> w48
    tunnel: [w381] -> w47
    stop <- "stop" stop-if-true
    n173 = flat-sequence {
      frame #0 {
      }
      frame #1 {
      }
    }
    n174 = flat-sequence {
      frame #0 {
      }
      frame #1 {
      }
    }
    n175 = property on="Preset positions" class="Ring (strict)"() -> ("Strings []"=w377:string[])  [unwired: 2 in, 2 out]
    n176 = event shown="[0] Timeout" {
      selector: _ -> [_ _ _ _ _ _ _ _ _ _ _ _ _ _ _ _ _ _ _ _ _ _ _ _ _]
      dyn-events: _ -> [_ _ _ _ _ _ _ _ _ _ _ _ _ _ _ _ _ _ _ _ _ _ _ _ _]
      timeout: 200 -> [_ _ _ _ _ _ _ _ _ _ _ _ _ _ _ _ _ _ _ _ _ _ _ _ _]
      tunnel: w396 -> [w517 _ _ _ _ _ _ _ _ _ _ _ w1247 _ _ _ _ w1540 _ _ w1644 w1660 w1704 w1792 w1937]
      tunnel: [w516 _ _ _ _ _ _ _ _ _ _ _ w1253 _ _ _ _ w1538 _ _ w1644 w1658 w1706 w1786 w1935] -> w397
      tunnel: w393 -> [w455 _ _ _ _ _ _ _ _ _ _ _ w1248 _ _ _ _ w1539 _ _ w1645 w1661 w1705 w1793 w1938]
      tunnel: [w515 _ _ _ _ _ _ _ _ _ _ _ w1254 _ _ _ _ w1535 _ _ w1645 w1659 w1707 w1787 w1936] -> w395
      tunnel: w392 -> [w454 _ _ _ _ _ _ _ _ _ _ _ _ _ _ w1441 w1501 _ _ _ _ w1655 w1697 w1795 w1934]
      tunnel: w391 -> [w492 _ _ _ _ _ _ _ _ _ _ _ _ _ _ w1440 w1500 _ _ _ _ w1654 w1696 w1794 w1933]
      tunnel: [w491 _ _ _ _ _ _ _ _ _ _ _ _ _ _ w1439 w1499 _ _ _ _ w1657 w1695 w1781 w1932] -> w390
      tunnel: [w490 _ _ _ _ _ _ _ _ _ _ _ _ _ _ w1438 w1498 _ _ _ _ w1656 w1694 w1780 w1931] -> w389
      tunnel: w388 -> [w464 _ _ _ _ _ _ _ _ _ _ _ _ w1310 _ _ _ _ w1573 _ _ w1653 w1691 w1791 w1930]
      tunnel: w387 -> [w467 _ _ _ _ _ _ _ _ _ _ _ _ w1309 _ _ _ _ w1572 _ _ w1652 w1690 w1790 w1929]
      tunnel: [w466 _ _ _ _ _ _ _ _ _ _ _ _ w1307 _ _ _ _ w1570 _ _ w1651 w1689 w1785 w1926] -> w386
      tunnel: [w465 _ _ _ _ _ _ _ _ _ _ _ _ w1308 _ _ _ _ w1571 _ _ w1650 w1688 w1784 w1925] -> w385
      tunnel: w384 -> [w463 _ _ _ _ _ _ _ _ _ _ _ _ _ w1374 _ _ _ _ w1610 _ w1649 w1685 w1789 w1928]
      tunnel: w383 -> [w462 _ _ _ _ _ _ _ _ _ _ _ _ _ w1373 _ _ _ _ w1609 _ w1648 w1684 w1788 w1927]
      tunnel: [w461 _ _ _ _ _ _ _ _ _ _ _ _ _ w1371 _ _ _ _ w1608 _ w1647 w1683 w1783 w1924] -> w382
      tunnel: [w460 _ _ _ _ _ _ _ _ _ _ _ _ _ w1372 _ _ _ _ w1607 _ w1646 w1682 w1782 w1923] -> w381
      event #0 {
        n177 = event-data() -> ()  [unwired: 1 in, 2 out]
        n178 = property on="X Step SP" class="DigNum (strict)"() -> ("Maximum"=w432:dbl)  [unwired: 2 in, 2 out]
        n179 = property on="Y Step SP" class="DigNum (strict)"() -> ("Maximum"=w437:dbl)  [unwired: 2 in, 2 out]
        n180 = flat-sequence {
          tunnel: [w626] -> w489
          tunnel: [w639] -> w488
          tunnel: [w649] -> w487
          tunnel: [w619] -> w486
          tunnel: w464 -> [w634]
          tunnel: w467 -> [w635]
          tunnel: w489 -> [w659]
          tunnel: [w659] -> w485
          tunnel: w488 -> [w658]
          tunnel: [w658] -> w484
          tunnel: w487 -> [w657]
          tunnel: [w657] -> w483
          tunnel: w486 -> [w654]
          tunnel: [w654] -> w482
          tunnel: w485 -> [w666]
          tunnel: [w667] -> w481
          tunnel: w484 -> [w669]
          tunnel: [w668] -> w480
          tunnel: w483 -> [w665]
          tunnel: [w664] -> w479
          tunnel: w482 -> [w664]
          tunnel: w481 -> [w679]
          tunnel: w480 -> [w680]
          tunnel: w479 -> [w682]
          tunnel: [w678] -> w465
          tunnel: [w677] -> w466
          frame #0 {
            w638 = 0.2 ("Delay Time (s)")
            n181 = property on="Z Step SP" class="DigNum (strict)"() -> ("Maximum"=w651:dbl)  [unwired: 2 in, 2 out]
            n182 = property on="Z Step SP" class="DigNum (strict)"() -> ("Minimum"=w653:dbl)  [unwired: 2 in, 2 out]
            n183 = property on="Z steps/rev" class="DigNum (strict)"() -> ("Value"=w647:u32)  [unwired: 2 in, 2 out]
            n184 = property on="Z offset mm" class="DigNum (strict)"() -> ("Value"=w643:dbl)  [unwired: 2 in, 2 out]
            n185 = To Long Integer(number=w651) -> (32bit integer=w650:i32)
            n186 = To Long Integer(number=w653) -> (32bit integer=w652:i32)
            n187 = To Double Precision Float(number=w647) -> (double precision float=w648:dbl)
            n188 = call "Applied Send Command.vi"("error in (no error)"=w635, "Command"=T1."Immediate Position?", "VISA resource name"=w634) -> ("error out"=w633:errorcluster, "read buffer"=w630:string, "VISA resource name out"=w628:refnum<visa-resource-name>)  [unwired: 4 in]
            n189 = call "Time Delay17"("error in (no error)"=w633, "Delay Time (s)"=w638) -> ("error out"=w618:errorcluster)  [unwired: 9 in]
            n190 = Hexadecimal String To Number(string=w630, offset=3) -> (number=w631:u32)  [unwired: 1 in, 1 out]
            n191 = To Long Integer(number=w631) -> (32bit integer=w641:i32)
            n192 = call "Applied Send Command.vi"("error in (no error)"=w618, "Command"=T1."Request Status", "VISA resource name"=w628) -> ("error out"=w627:errorcluster, "read buffer"=w623:string, "VISA resource name out"=w626:refnum<visa-resource-name>)  [unwired: 4 in]
            n193 = property on="Z Step PV" class="DigNum (strict)"("Val(Sgnl)"=w641) -> ()  [unwired: 2 in, 2 out]
            n194 = call "Time Delay16"("error in (no error)"=w627, "Delay Time (s)"=w638) -> ("error out"=w639:errorcluster)  [unwired: 9 in]
            n195 = String Subset(string=w623, offset (0)=0, length (rest)=1 ("length (rest)")) -> (substring=w620:string)
            n196 = In Range and Coerce(upper limit=w650, x=w641, lower limit=w652) -> (In Range?=w649:bool)  [unwired: 1 out]
            n197 = To Double Precision Float(number=w641) -> (double precision float=w642:dbl)
            n198 = Not Equal?(x=w620, y="R") -> (x != y?=w619:bool)
            n199 = Equal?(x=w620, y="R") -> (x = y?=w637:bool)
            n200 = property on="Z in Motion" class="Bool (strict)"("Val(Sgnl)"=w619) -> ()  [unwired: 2 in, 2 out]
            n201 = property on="Z in Range" class="Bool (strict)"("Val(Sgnl)"=w649) -> ()  [unwired: 2 in, 2 out]
            n202 = property on="Z Ready" class="Bool (strict)"("Val(Sgnl)"=w637) -> ()  [unwired: 2 in, 2 out]
            n203 = Divide(x=w642, y=w648) -> (x/y=w646:dbl)
            n204 = property on="Z mm/rev" class="DigNum (strict)"() -> ("Value"=w645:dbl)  [unwired: 2 in, 2 out]
            n205 = Multiply(x=w646, y=w645) -> (x*y=w644:dbl)
            n206 = Add(x=w644, y=w643) -> (x+y=w640:dbl)
            n207 = property on="Z Position mm PV" class="DigNum (strict)"("Val(Sgnl)"=w640) -> ()  [unwired: 2 in, 2 out]
          }
          frame #1 {
            n208 = property on="Z Scan" class="Bool (strict)"() -> ("Value"=w655:bool)  [unwired: 2 in, 2 out]
            n209 = Or(x=w654, y=w655) -> (x .or. y?=w656:bool)
            n210 = case shown="True" w656 {
              frame #0 {
                n211 = property on="Z Scan OK" class="Bool"("DisabledEnum"=T2."Enabled" ("Disabled")) -> ()  [unwired: 2 in, 2 out]
                n212 = property on="Z Go" class="Bool"("DisabledEnum"=T2."Enabled" ("Disabled")) -> ()  [unwired: 2 in, 2 out]
              }
              frame #1 {
                n213 = property on="Z Scan OK" class="Bool"("DisabledEnum"=T2."Disabled and Grayed Out" ("Disabled")) -> ()  [unwired: 2 in, 2 out]
                n214 = property on="Z Go" class="Bool"("DisabledEnum"=T2."Disabled and Grayed Out" ("Disabled")) -> ()  [unwired: 2 in, 2 out]
              }
            }
          }
          frame #2 {
            n215 = case shown="False" w665 {
              tunnel: w666 -> [w673 w676]
              tunnel: [w671 w676] -> w667
              tunnel: [w670 w675] -> w668
              tunnel: w669 -> [w672 w675]
              frame #0 {
                n216 = call "Applied Send Command.vi"("error in (no error)"=w672, "Command"=T1."Stop & Kill Buffer", "VISA resource name"=w673) -> ("error out"=w670:errorcluster, "VISA resource name out"=w671:refnum<visa-resource-name>)  [unwired: 4 in, 1 out]
              }
              frame #1 {
              }
            }
          }
          frame #3 {
            n217 = property on="Z Backlash corr" class="Bool (strict)"() -> ("Value"=w683:bool)  [unwired: 2 in, 2 out]
            n218 = Implies(1:w682, 2:w683) -> (0:w681:bool)
            n219 = case shown="False" w681 {
              tunnel: w680 -> [w684 w716]
              tunnel: w679 -> [w685 w717]
              tunnel: [w686 w716] -> w678
              tunnel: [w687 w717] -> w677
              frame #0 {
                w713 = 0.1 ("Delay Time (s)")
                # "Backlash"
                # "Backlash"
                n220 = property on="Z Backlash" class="DigNum (strict)"() -> ("Value"=w691:i32)  [unwired: 2 in, 2 out]
                n221 = To Long Integer(number=w691) -> (32bit integer=w694:i32)
                n222 = property on="Z Backlash corr" class="Bool (strict)"("Val(Sgnl)"=FALSE ("Value (Signaling)")) -> ()  [unwired: 2 in, 2 out]
                n223 = Number To Decimal String(number=w691) -> (decimal integer string=w699:string)  [unwired: 1 in]
                n224 = Negate(x=w694) -> (-x=w693:i32)
                n225 = property on="Z Backlash steps/sec" class="DigNum (strict)"() -> ("Value"=w690:i32)  [unwired: 2 in, 2 out]
                n226 = Number To Decimal String(number=w693) -> (decimal integer string=w700:string)  [unwired: 1 in]
                n227 = property on="Z steps/rev" class="DigNum (strict)"() -> ("Value"=w689:u32)  [unwired: 2 in, 2 out]
                n228 = Divide(x=w690, y=w689) -> (x/y=w714:dbl)
                n229 = Number To Fractional String(number=w714) -> (F-format string=w715:string)  [unwired: 3 in]
                n230 = call "Applied Send Command.vi"("error in (no error)"=w684, "Extra"=w715, "Command"=T1."Velocity Setting", "VISA resource name"=w685) -> ("error out"=w711:errorcluster, "VISA resource name out"=w704:refnum<visa-resource-name>)  [unwired: 3 in, 1 out]
                n231 = call "Time Delay47"("error in (no error)"=w711, "Delay Time (s)"=w713) -> ("error out"=w712:errorcluster)  [unwired: 9 in]
                n232 = call "Applied Send Command.vi"("error in (no error)"=w712, "Extra"=w699, "Command"=T1."Distance or Position", "VISA resource name"=w704) -> ("error out"=w705:errorcluster, "VISA resource name out"=w698:refnum<visa-resource-name>)  [unwired: 3 in, 1 out]
                n233 = call "Time Delay44"("error in (no error)"=w705, "Delay Time (s)"=w713) -> ("error out"=w706:errorcluster)  [unwired: 9 in]
                n234 = call "Applied Send Command.vi"("error in (no error)"=w706, "Command"=T1."Feed to Length", "VISA resource name"=w698) -> ("error out"=w707:errorcluster, "VISA resource name out"=w701:refnum<visa-resource-name>)  [unwired: 4 in, 1 out]
                n235 = call "Time Delay45"("error in (no error)"=w707, "Delay Time (s)"=w713) -> ("error out"=w708:errorcluster)  [unwired: 9 in]
                n236 = call "Applied Send Command.vi"("error in (no error)"=w708, "Extra"=w700, "Command"=T1."Distance or Position", "VISA resource name"=w701) -> ("error out"=w709:errorcluster, "VISA resource name out"=w702:refnum<visa-resource-name>)  [unwired: 3 in, 1 out]
                n237 = call "Time Delay46"("error in (no error)"=w709, "Delay Time (s)"=w713) -> ("error out"=w710:errorcluster)  [unwired: 9 in]
                n238 = call "Applied Send Command.vi"("error in (no error)"=w710, "Command"=T1."Feed to Length", "VISA resource name"=w702) -> ("error out"=w686:errorcluster, "VISA resource name out"=w687:refnum<visa-resource-name>)  [unwired: 4 in, 1 out]
              }
              frame #1 {
              }
            }
          }
        }
        n239 = flat-sequence {
          tunnel: [w527] -> w478
          tunnel: [w539] -> w477
          tunnel: [w549] -> w476
          tunnel: [w518] -> w475
          tunnel: w463 -> [w536]
          tunnel: w462 -> [w535]
          tunnel: w478 -> [w559]
          tunnel: [w559] -> w474
          tunnel: w477 -> [w558]
          tunnel: [w558] -> w473
          tunnel: w476 -> [w557]
          tunnel: [w557] -> w472
          tunnel: w475 -> [w554]
          tunnel: [w554] -> w471
          tunnel: w474 -> [w566]
          tunnel: [w567] -> w470
          tunnel: w473 -> [w569]
          tunnel: [w568] -> w469
          tunnel: w472 -> [w565]
          tunnel: [w564] -> w468
          tunnel: w471 -> [w564]
          tunnel: w470 -> [w579]
          tunnel: w469 -> [w580]
          tunnel: w468 -> [w582]
          tunnel: [w578] -> w460
          tunnel: [w577] -> w461
          frame #0 {
            w538 = 0.2 ("Delay Time (s)")
            n240 = property on="R Step SP" class="DigNum (strict)"() -> ("Maximum"=w551:dbl)  [unwired: 2 in, 2 out]
            n241 = property on="R Step SP" class="DigNum (strict)"() -> ("Minimum"=w553:dbl)  [unwired: 2 in, 2 out]
            n242 = property on="R steps/rev" class="DigNum (strict)"() -> ("Value"=w547:u32)  [unwired: 2 in, 2 out]
            n243 = property on="R offset deg" class="DigNum (strict)"() -> ("Value"=w543:dbl)  [unwired: 2 in, 2 out]
            n244 = To Long Integer(number=w551) -> (32bit integer=w550:i32)
            n245 = To Long Integer(number=w553) -> (32bit integer=w552:i32)
            n246 = To Double Precision Float(number=w547) -> (double precision float=w548:dbl)
            n247 = call "Applied Send Command.vi"("error in (no error)"=w535, "Command"=T1."Immediate Position?", "VISA resource name"=w536) -> ("error out"=w531:errorcluster, "read buffer"=w532:string, "VISA resource name out"=w529:refnum<visa-resource-name>)  [unwired: 4 in]
            n248 = call "Time Delay21"("error in (no error)"=w531, "Delay Time (s)"=w538) -> ("error out"=w528:errorcluster)  [unwired: 9 in]
            n249 = Hexadecimal String To Number(string=w532, offset=3) -> (number=w533:u32)  [unwired: 1 in, 1 out]
            n250 = To Long Integer(number=w533) -> (32bit integer=w541:i32)
            n251 = call "Applied Send Command.vi"("error in (no error)"=w528, "Command"=T1."Request Status", "VISA resource name"=w529) -> ("error out"=w526:errorcluster, "read buffer"=w523:string, "VISA resource name out"=w527:refnum<visa-resource-name>)  [unwired: 4 in]
            n252 = property on="R Step PV" class="DigNum (strict)"("Val(Sgnl)"=w541) -> ()  [unwired: 2 in, 2 out]
            n253 = call "Time Delay20"("error in (no error)"=w526, "Delay Time (s)"=w538) -> ("error out"=w539:errorcluster)  [unwired: 9 in]
            n254 = String Subset(string=w523, offset (0)=0, length (rest)=1 ("length (rest)")) -> (substring=w519:string)
            n255 = In Range and Coerce(upper limit=w550, x=w541, lower limit=w552) -> (In Range?=w549:bool)  [unwired: 1 out]
            n256 = To Double Precision Float(number=w541) -> (double precision float=w542:dbl)
            n257 = Not Equal?(x=w519, y="R") -> (x != y?=w518:bool)
            n258 = Equal?(x=w519, y="R") -> (x = y?=w520:bool)
            n259 = property on="R in Motion" class="Bool (strict)"("Val(Sgnl)"=w518) -> ()  [unwired: 2 in, 2 out]
            n260 = property on="R in Range" class="Bool (strict)"("Val(Sgnl)"=w549) -> ()  [unwired: 2 in, 2 out]
            n261 = property on="R Ready" class="Bool (strict)"("Val(Sgnl)"=w520) -> ()  [unwired: 2 in, 2 out]
            n262 = Divide(x=w542, y=w548) -> (x/y=w546:dbl)
            n263 = property on="R deg/rev" class="DigNum (strict)"() -> ("Value"=w545:dbl)  [unwired: 2 in, 2 out]
            n264 = Multiply(x=w546, y=w545) -> (x*y=w544:dbl)
            n265 = Add(x=w544, y=w543) -> (x+y=w540:dbl)
            n266 = property on="R Position deg PV" class="DigNum (strict)"("Val(Sgnl)"=w540) -> ()  [unwired: 2 in, 2 out]
          }
          frame #1 {
            n267 = property on="R Scan" class="Bool (strict)"() -> ("Value"=w555:bool)  [unwired: 2 in, 2 out]
            n268 = Or(x=w554, y=w555) -> (x .or. y?=w556:bool)
            n269 = case shown="True" w556 {
              frame #0 {
                n270 = property on="R Scan OK" class="Bool"("DisabledEnum"=T2."Enabled" ("Disabled")) -> ()  [unwired: 2 in, 2 out]
                n271 = property on="R Go" class="Bool"("DisabledEnum"=T2."Enabled" ("Disabled")) -> ()  [unwired: 2 in, 2 out]
              }
              frame #1 {
                n272 = property on="R Scan OK" class="Bool"("DisabledEnum"=T2."Disabled and Grayed Out" ("Disabled")) -> ()  [unwired: 2 in, 2 out]
                n273 = property on="R Go" class="Bool"("DisabledEnum"=T2."Disabled and Grayed Out" ("Disabled")) -> ()  [unwired: 2 in, 2 out]
              }
            }
          }
          frame #2 {
            n274 = case shown="False" w565 {
              tunnel: w566 -> [w573 w576]
              tunnel: [w571 w576] -> w567
              tunnel: [w570 w575] -> w568
              tunnel: w569 -> [w572 w575]
              frame #0 {
                n275 = call "Applied Send Command.vi"("error in (no error)"=w572, "Command"=T1."Stop & Kill Buffer", "VISA resource name"=w573) -> ("error out"=w570:errorcluster, "VISA resource name out"=w571:refnum<visa-resource-name>)  [unwired: 4 in, 1 out]
              }
              frame #1 {
              }
            }
          }
          frame #3 {
            n276 = property on="R Backlash corr" class="Bool (strict)"() -> ("Value"=w583:bool)  [unwired: 2 in, 2 out]
            n277 = Implies(1:w582, 2:w583) -> (0:w581:bool)
            n278 = case shown="False" w581 {
              tunnel: w580 -> [w587 w616]
              tunnel: w579 -> [w586 w617]
              tunnel: [w584 w616] -> w578
              tunnel: [w585 w617] -> w577
              frame #0 {
                w594 = 0.1 ("Delay Time (s)")
                # "Backlash"
                # "Backlash"
                n279 = property on="R Backlash" class="DigNum (strict)"() -> ("Value"=w588:i32)  [unwired: 2 in, 2 out]
                n280 = To Long Integer(number=w588) -> (32bit integer=w613:i32)
                n281 = property on="R Backlash corr" class="Bool (strict)"("Val(Sgnl)"=FALSE ("Value (Signaling)")) -> ()  [unwired: 2 in, 2 out]
                n282 = Number To Decimal String(number=w588) -> (decimal integer string=w608:string)  [unwired: 1 in]
                n283 = Negate(x=w613) -> (-x=w614:i32)
                n284 = property on="R Backlash steps/sec" class="DigNum (strict)"() -> ("Value"=w591:i32)  [unwired: 2 in, 2 out]
                n285 = Number To Decimal String(number=w614) -> (decimal integer string=w607:string)  [unwired: 1 in]
                n286 = property on="R steps/rev" class="DigNum (strict)"() -> ("Value"=w589:u32)  [unwired: 2 in, 2 out]
                n287 = Divide(x=w591, y=w589) -> (x/y=w590:dbl)
                n288 = Number To Fractional String(number=w590) -> (F-format string=w593:string)  [unwired: 3 in]
                n289 = call "Applied Send Command.vi"("error in (no error)"=w587, "Extra"=w593, "Command"=T1."Velocity Setting", "VISA resource name"=w586) -> ("error out"=w596:errorcluster, "VISA resource name out"=w603:refnum<visa-resource-name>)  [unwired: 3 in, 1 out]
                n290 = call "Time Delay49"("error in (no error)"=w596, "Delay Time (s)"=w594) -> ("error out"=w595:errorcluster)  [unwired: 9 in]
                n291 = call "Applied Send Command.vi"("error in (no error)"=w595, "Extra"=w608, "Command"=T1."Distance or Position", "VISA resource name"=w603) -> ("error out"=w602:errorcluster, "VISA resource name out"=w609:refnum<visa-resource-name>)  [unwired: 3 in, 1 out]
                n292 = call "Time Delay18"("error in (no error)"=w602, "Delay Time (s)"=w594) -> ("error out"=w601:errorcluster)  [unwired: 9 in]
                n293 = call "Applied Send Command.vi"("error in (no error)"=w601, "Command"=T1."Feed to Length", "VISA resource name"=w609) -> ("error out"=w600:errorcluster, "VISA resource name out"=w606:refnum<visa-resource-name>)  [unwired: 4 in, 1 out]
                n294 = call "Time Delay19"("error in (no error)"=w600, "Delay Time (s)"=w594) -> ("error out"=w599:errorcluster)  [unwired: 9 in]
                n295 = call "Applied Send Command.vi"("error in (no error)"=w599, "Extra"=w607, "Command"=T1."Distance or Position", "VISA resource name"=w606) -> ("error out"=w598:errorcluster, "VISA resource name out"=w605:refnum<visa-resource-name>)  [unwired: 3 in, 1 out]
                n296 = call "Time Delay48"("error in (no error)"=w598, "Delay Time (s)"=w594) -> ("error out"=w597:errorcluster)  [unwired: 9 in]
                n297 = call "Applied Send Command.vi"("error in (no error)"=w597, "Command"=T1."Feed to Length", "VISA resource name"=w605) -> ("error out"=w584:errorcluster, "VISA resource name out"=w585:refnum<visa-resource-name>)  [unwired: 4 in, 1 out]
              }
              frame #1 {
              }
            }
          }
        }
        n298 = property on="X Step SP" class="DigNum (strict)"() -> ("Minimum"=w433:dbl)  [unwired: 2 in, 2 out]
        n299 = property on="Y Step SP" class="DigNum (strict)"() -> ("Minimum"=w436:dbl)  [unwired: 2 in, 2 out]
        n300 = property on="X Step PV" class="DigNum (strict)"() -> ("Value"=w431:i32)  [unwired: 2 in, 2 out]
        n301 = property on="Y Step PV" class="DigNum (strict)"() -> ("Value"=w430:i32)  [unwired: 2 in, 2 out]
        n302 = Subtract(x=w432, y=w433) -> (x-y=w434:dbl)
        n303 = Absolute Value(x=w431) -> (abs(x)=w428:i32)
        n304 = Absolute Value(x=w430) -> (abs(x)=w429:i32)
        n305 = Subtract(x=w437, y=w436) -> (x-y=w438:dbl)
        n306 = property on="X Position mm PV" class="DigNum (strict)"() -> ("Value"=w456:dbl)  [unwired: 2 in, 2 out]
        n307 = property on="Y Position mm PV" class="DigNum (strict)"() -> ("Value"=w449:dbl)  [unwired: 2 in, 2 out]
        n308 = property on="Z Position mm PV" class="DigNum (strict)"() -> ("Value"=w450:dbl)  [unwired: 2 in, 2 out]
        n309 = property on="R Position deg PV" class="DigNum (strict)"() -> ("Value"=w457:dbl)  [unwired: 2 in, 2 out]
        n310 = property on="Y Scan Length SP steps" class="DigNum (strict)"() -> ("Value"=w441:i32)  [unwired: 2 in, 2 out]
        n311 = property on="Z Scan Length SP steps" class="DigNum (strict)"() -> ("Value"=w442:i32)  [unwired: 2 in, 2 out]
        n312 = Multiply(x=w428, y=w429) -> (x*y=w423:i32)
        n313 = Divide(x=w438, y=2.0) -> (x/y=w426:dbl)
        n314 = Divide(x=w434, y=2.0) -> (x/y=w427:dbl)
        n315 = call "Build XY Graph"("Reset"=TRUE, "Y Input"=w449, "X Input"=w456) -> ("XY Graph"=→"XY Graph":cluster{"Y":dbl[], "Y":dbl[]}[])  [unwired: 7 in, 1 out]
        n316 = call "Build XY Graph2"("Reset"=TRUE, "Y Input"=w457, "X Input"=w450) -> ("XY Graph"=→"ZR Graph":cluster{"Y":dbl[], "Y":dbl[]}[])  [unwired: 7 in, 1 out]
        n317 = property on="Clear ZY" class="Bool (strict)"() -> ("Value"=w440:bool)  [unwired: 2 in, 2 out]
        n318 = Absolute Value(x=w426) -> (abs(x)=w424:dbl)
        n319 = Absolute Value(x=w427) -> (abs(x)=w425:dbl)
        n320 = call "Build XY Graph3"("Reset"=w440, "Y Input"=w449, "X Input"=w450) -> ("XY Graph"=→"ZY Graph":cluster{"Y":dbl[], "Y":dbl[]}[])  [unwired: 7 in, 1 out]
        n321 = Divide(x=w441, y=w442) -> (x/y=w443:dbl)
        n322 = Multiply(x=w424, y=w425) -> (x*y=w422:dbl)
        n323 = Inverse Tangent(1:w443) -> (0:w444:dbl)
        n324 = Less Or Equal?(x=w423, y=w422) -> (x <= y?=w421:bool)
        n325 = Divide(x=w444, y=6.283185307179586) -> (x/y=w445:dbl)
        n326 = flat-sequence {
          tunnel: [w730] -> w503
          tunnel: [w741] -> w502
          tunnel: [w719] -> w501
          tunnel: [w726] -> w500
          tunnel: w454 -> [w737]
          tunnel: w492 -> [w725]
          tunnel: w432 -> [w721]
          tunnel: w433 -> [w720]
          tunnel: w421 -> [w718]
          tunnel: w503 -> [w761]
          tunnel: [w761] -> w499
          tunnel: w502 -> [w760]
          tunnel: [w760] -> w498
          tunnel: w501 -> [w759]
          tunnel: [w759] -> w497
          tunnel: w500 -> [w756]
          tunnel: [w756] -> w496
          tunnel: w499 -> [w770]
          tunnel: [w767] -> w495
          tunnel: w498 -> [w769]
          tunnel: [w768] -> w494
          tunnel: w497 -> [w766]
          tunnel: [w771] -> w493
          tunnel: w496 -> [w771]
          tunnel: w495 -> [w782]
          tunnel: w494 -> [w783]
          tunnel: w493 -> [w784]
          tunnel: [w781] -> w490
          tunnel: [w780] -> w491
          frame #0 {
            w740 = 0.2 ("Delay Time (s)")
            n327 = To Long Integer(number=w721) -> (32bit integer=w753:i32)
            n328 = To Long Integer(number=w720) -> (32bit integer=w754:i32)
            n329 = property on="X steps/rev" class="DigNum (strict)"() -> ("Value"=w750:u32)  [unwired: 2 in, 2 out]
            n330 = property on="X offset mm" class="DigNum (strict)"() -> ("Value"=w746:dbl)  [unwired: 2 in, 2 out]
            n331 = To Double Precision Float(number=w750) -> (double precision float=w751:dbl)
            n332 = call "Applied Send Command.vi"("error in (no error)"=w725, "Command"=T1."Immediate Position?", "VISA resource name"=w737) -> ("error out"=w735:errorcluster, "read buffer"=w736:string, "VISA resource name out"=w731:refnum<visa-resource-name>)  [unwired: 4 in]
            n333 = call "Time Delay12"("error in (no error)"=w735, "Delay Time (s)"=w740) -> ("error out"=w728:errorcluster)  [unwired: 9 in]
            n334 = Hexadecimal String To Number(string=w736, offset=3) -> (number=w742:u32)  [unwired: 1 in, 1 out]
            n335 = To Long Integer(number=w742) -> (32bit integer=w744:i32)
            n336 = call "Applied Send Command.vi"("error in (no error)"=w728, "Command"=T1."Request Status", "VISA resource name"=w731) -> ("error out"=w729:errorcluster, "read buffer"=w733:string, "VISA resource name out"=w730:refnum<visa-resource-name>)  [unwired: 4 in]
            n337 = property on="X Step PV" class="DigNum (strict)"("Val(Sgnl)"=w744) -> ()  [unwired: 2 in, 2 out]
            n338 = call "Time Delay11"("error in (no error)"=w729, "Delay Time (s)"=w740) -> ("error out"=w741:errorcluster)  [unwired: 9 in]
            n339 = String Subset(string=w733, offset (0)=0, length (rest)=1 ("length (rest)")) -> (substring=w722:string)
            n340 = In Range and Coerce(upper limit=w753, x=w744, lower limit=w754) -> (In Range?=w752:bool)  [unwired: 1 out]
            n341 = To Double Precision Float(number=w744) -> (double precision float=w745:dbl)
            n342 = Not Equal?(x=w722, y="R") -> (x != y?=w726:bool)
            n343 = Equal?(x=w722, y="R") -> (x = y?=w739:bool)
            n344 = property on="X  in Motion" class="Bool (strict)"("Val(Sgnl)"=w726) -> ()  [unwired: 2 in, 2 out]
            n345 = property on="X Ready" class="Bool (strict)"("Val(Sgnl)"=w739) -> ()  [unwired: 2 in, 2 out]
            n346 = Divide(x=w745, y=w751) -> (x/y=w749:dbl)
            n347 = And(x=w718, y=w752) -> (x .and. y?=w719:bool)
            n348 = property on="X  in Range" class="Bool (strict)"("Val(Sgnl)"=w719) -> ()  [unwired: 2 in, 2 out]
            n349 = property on="X mm/rev" class="DigNum (strict)"() -> ("Value"=w748:dbl)  [unwired: 2 in, 2 out]
            n350 = Multiply(x=w749, y=w748) -> (x*y=w747:dbl)
            n351 = Add(x=w747, y=w746) -> (x+y=w743:dbl)
            n352 = property on="X Position mm PV" class="DigNum (strict)"("Val(Sgnl)"=w743) -> ()  [unwired: 2 in, 2 out]
          }
          frame #1 {
            n353 = property on="X Scan" class="Bool (strict)"() -> ("Value"=w757:bool)  [unwired: 2 in, 2 out]
            n354 = Or(x=w756, y=w757) -> (x .or. y?=w758:bool)
            n355 = case shown="True" w758 {
              frame #0 {
                n356 = property on="X Scan OK" class="Bool"("DisabledEnum"=T2."Enabled" ("Disabled")) -> ()  [unwired: 2 in, 2 out]
                n357 = property on="X Go" class="Bool"("DisabledEnum"=T2."Enabled" ("Disabled")) -> ()  [unwired: 2 in, 2 out]
              }
              frame #1 {
                n358 = property on="X Scan OK" class="Bool"("DisabledEnum"=T2."Disabled and Grayed Out" ("Disabled")) -> ()  [unwired: 2 in, 2 out]
                n359 = property on="X Go" class="Bool"("DisabledEnum"=T2."Disabled and Grayed Out" ("Disabled")) -> ()  [unwired: 2 in, 2 out]
              }
            }
          }
          frame #2 {
            n360 = case shown="False" w766 {
              tunnel: w770 -> [w773 w778]
              tunnel: [w775 w778] -> w767
              tunnel: [w776 w777] -> w768
              tunnel: w769 -> [w772 w777]
              frame #0 {
                n361 = call "Applied Send Command.vi"("error in (no error)"=w772, "Command"=T1."Stop & Kill Buffer", "VISA resource name"=w773) -> ("error out"=w776:errorcluster, "VISA resource name out"=w775:refnum<visa-resource-name>)  [unwired: 4 in, 1 out]
              }
              frame #1 {
              }
            }
          }
          frame #3 {
            n362 = property on="X Backlash corr" class="Bool (strict)"() -> ("Value"=w785:bool)  [unwired: 2 in, 2 out]
            n363 = Implies(1:w784, 2:w785) -> (0:w779:bool)
            n364 = case shown="False" w779 {
              tunnel: w783 -> [w799 w818]
              tunnel: w782 -> [w800 w819]
              tunnel: [w802 w818] -> w781
              tunnel: [w801 w819] -> w780
              frame #0 {
                w790 = 0.1 ("Delay Time (s)")
                # "Backlash"
                n365 = property on="X Backlash" class="DigNum (strict)"() -> ("Value"=w805:i32)  [unwired: 2 in, 2 out]
                n366 = To Long Integer(number=w805) -> (32bit integer=w814:i32)
                n367 = property on="X Backlash corr" class="Bool (strict)"("Val(Sgnl)"=FALSE ("Value (Signaling)")) -> ()  [unwired: 2 in, 2 out]
                n368 = Number To Decimal String(number=w805) -> (decimal integer string=w809:string)  [unwired: 1 in]
                n369 = Negate(x=w814) -> (-x=w815:i32)
                n370 = property on="X Backlash steps/sec" class="DigNum (strict)"() -> ("Value"=w789:i32)  [unwired: 2 in, 2 out]
                n371 = Number To Decimal String(number=w815) -> (decimal integer string=w808:string)  [unwired: 1 in]
                n372 = property on="X steps/rev" class="DigNum (strict)"() -> ("Value"=w788:u32)  [unwired: 2 in, 2 out]
                n373 = Divide(x=w789, y=w788) -> (x/y=w787:dbl)
                n374 = Number To Fractional String(number=w787) -> (F-format string=w786:string)  [unwired: 3 in]
                n375 = call "Applied Send Command.vi"("error in (no error)"=w799, "Extra"=w786, "Command"=T1."Velocity Setting", "VISA resource name"=w800) -> ("error out"=w792:errorcluster, "VISA resource name out"=w803:refnum<visa-resource-name>)  [unwired: 3 in, 1 out]
                n376 = call "Time Delay35"("error in (no error)"=w792, "Delay Time (s)"=w790) -> ("error out"=w791:errorcluster)  [unwired: 9 in]
                n377 = call "Applied Send Command.vi"("error in (no error)"=w791, "Extra"=w809, "Command"=T1."Distance or Position", "VISA resource name"=w803) -> ("error out"=w798:errorcluster, "VISA resource name out"=w810:refnum<visa-resource-name>)  [unwired: 3 in, 1 out]
                n378 = call "Time Delay32"("error in (no error)"=w798, "Delay Time (s)"=w790) -> ("error out"=w797:errorcluster)  [unwired: 9 in]
                n379 = call "Applied Send Command.vi"("error in (no error)"=w797, "Command"=T1."Feed to Length", "VISA resource name"=w810) -> ("error out"=w796:errorcluster, "VISA resource name out"=w807:refnum<visa-resource-name>)  [unwired: 4 in, 1 out]
                n380 = call "Time Delay33"("error in (no error)"=w796, "Delay Time (s)"=w790) -> ("error out"=w795:errorcluster)  [unwired: 9 in]
                n381 = call "Applied Send Command.vi"("error in (no error)"=w795, "Extra"=w808, "Command"=T1."Distance or Position", "VISA resource name"=w807) -> ("error out"=w794:errorcluster, "VISA resource name out"=w806:refnum<visa-resource-name>)  [unwired: 3 in, 1 out]
                n382 = call "Time Delay34"("error in (no error)"=w794, "Delay Time (s)"=w790) -> ("error out"=w793:errorcluster)  [unwired: 9 in]
                n383 = call "Applied Send Command.vi"("error in (no error)"=w793, "Command"=T1."Feed to Length", "VISA resource name"=w806) -> ("error out"=w802:errorcluster, "VISA resource name out"=w801:refnum<visa-resource-name>)  [unwired: 4 in, 1 out]
              }
              frame #1 {
              }
            }
          }
        }
        n384 = flat-sequence {
          tunnel: w517 -> [w836]
          tunnel: w455 -> [w837]
          tunnel: [w833] -> w514
          tunnel: [w843] -> w512
          tunnel: [w822] -> w510
          tunnel: [w824] -> w508
          tunnel: w437 -> [w823]
          tunnel: w436 -> [w820]
          tunnel: w421 -> [w821]
          tunnel: w514 -> [w863]
          tunnel: [w863] -> w513
          tunnel: w512 -> [w862]
          tunnel: [w862] -> w511
          tunnel: w510 -> [w861]
          tunnel: [w861] -> w509
          tunnel: w508 -> [w858]
          tunnel: [w858] -> w504
          tunnel: w513 -> [w870]
          tunnel: [w871] -> w507
          tunnel: w511 -> [w873]
          tunnel: [w872] -> w506
          tunnel: w509 -> [w869]
          tunnel: [w868] -> w505
          tunnel: w504 -> [w868]
          tunnel: w507 -> [w883]
          tunnel: w506 -> [w884]
          tunnel: w505 -> [w886]
          tunnel: [w882] -> w516
          tunnel: [w881] -> w515
          frame #0 {
            w842 = 0.2 ("Delay Time (s)")
            n385 = To Long Integer(number=w823) -> (32bit integer=w855:i32)
            n386 = To Long Integer(number=w820) -> (32bit integer=w856:i32)
            n387 = property on="Y steps/rev" class="DigNum (strict)"() -> ("Value"=w852:u32)  [unwired: 2 in, 2 out]
            n388 = property on="Y offset mm" class="DigNum (strict)"() -> ("Value"=w848:dbl)  [unwired: 2 in, 2 out]
            n389 = To Double Precision Float(number=w852) -> (double precision float=w853:dbl)
            n390 = call "Applied Send Command.vi"("error in (no error)"=w836, "Command"=T1."Immediate Position?", "VISA resource name"=w837) -> ("error out"=w839:errorcluster, "read buffer"=w840:string, "VISA resource name out"=w834:refnum<visa-resource-name>)  [unwired: 4 in]
            n391 = call "Time Delay4"("error in (no error)"=w839, "Delay Time (s)"=w842) -> ("error out"=w832:errorcluster)  [unwired: 9 in]
            n392 = Hexadecimal String To Number(string=w840, offset=3) -> (number=w844:u32)  [unwired: 1 in, 1 out]
            n393 = To Long Integer(number=w844) -> (32bit integer=w846:i32)
            n394 = call "Applied Send Command.vi"("error in (no error)"=w832, "Command"=T1."Request Status", "VISA resource name"=w834) -> ("error out"=w831:errorcluster, "read buffer"=w828:string, "VISA resource name out"=w833:refnum<visa-resource-name>)  [unwired: 4 in]
            n395 = property on="Y Step PV" class="DigNum (strict)"("Val(Sgnl)"=w846) -> ()  [unwired: 2 in, 2 out]
            n396 = call "Time Delay3"("error in (no error)"=w831, "Delay Time (s)"=w842) -> ("error out"=w843:errorcluster)  [unwired: 9 in]
            n397 = String Subset(string=w828, offset (0)=0, length (rest)=1 ("length (rest)")) -> (substring=w826:string)
            n398 = In Range and Coerce(upper limit=w855, x=w846, lower limit=w856) -> (In Range?=w854:bool)  [unwired: 1 out]
            n399 = To Double Precision Float(number=w846) -> (double precision float=w847:dbl)
            n400 = Not Equal?(x=w826, y="R") -> (x != y?=w824:bool)
            n401 = Equal?(x=w826, y="R") -> (x = y?=w841:bool)
            n402 = property on="Y in Motion" class="Bool (strict)"("Val(Sgnl)"=w824) -> ()  [unwired: 2 in, 2 out]
            n403 = property on="Y Ready" class="Bool (strict)"("Val(Sgnl)"=w841) -> ()  [unwired: 2 in, 2 out]
            n404 = Divide(x=w847, y=w853) -> (x/y=w851:dbl)
            n405 = And(x=w854, y=w821) -> (x .and. y?=w822:bool)
            n406 = property on="Y in Range" class="Bool (strict)"("Val(Sgnl)"=w822) -> ()  [unwired: 2 in, 2 out]
            n407 = property on="Y mm/rev" class="DigNum (strict)"() -> ("Value"=w850:dbl)  [unwired: 2 in, 2 out]
            n408 = Multiply(x=w851, y=w850) -> (x*y=w849:dbl)
            n409 = Add(x=w849, y=w848) -> (x+y=w845:dbl)
            n410 = property on="Y Position mm PV" class="DigNum (strict)"("Val(Sgnl)"=w845) -> ()  [unwired: 2 in, 2 out]
          }
          frame #1 {
            n411 = property on="Y Scan" class="Bool (strict)"() -> ("Value"=w859:bool)  [unwired: 2 in, 2 out]
            n412 = Or(x=w858, y=w859) -> (x .or. y?=w860:bool)
            n413 = case shown="True" w860 {
              frame #0 {
                n414 = property on="Y Scan OK" class="Bool"("DisabledEnum"=T2."Enabled" ("Disabled")) -> ()  [unwired: 2 in, 2 out]
                n415 = property on="Y Go" class="Bool"("DisabledEnum"=T2."Enabled" ("Disabled")) -> ()  [unwired: 2 in, 2 out]
              }
              frame #1 {
                n416 = property on="Y Scan OK" class="Bool"("DisabledEnum"=T2."Disabled and Grayed Out" ("Disabled")) -> ()  [unwired: 2 in, 2 out]
                n417 = property on="Y Go" class="Bool"("DisabledEnum"=T2."Disabled and Grayed Out" ("Disabled")) -> ()  [unwired: 2 in, 2 out]
              }
            }
          }
          frame #2 {
            n418 = case shown="False" w869 {
              tunnel: w870 -> [w875 w880]
              tunnel: [w877 w880] -> w871
              tunnel: [w876 w879] -> w872
              tunnel: w873 -> [w874 w879]
              frame #0 {
                n419 = call "Applied Send Command.vi"("error in (no error)"=w874, "Command"=T1."Stop & Kill Buffer", "VISA resource name"=w875) -> ("error out"=w876:errorcluster, "VISA resource name out"=w877:refnum<visa-resource-name>)  [unwired: 4 in, 1 out]
              }
              frame #1 {
              }
            }
          }
          frame #3 {
            n420 = property on="Y Backlash corr" class="Bool (strict)"() -> ("Value"=w887:bool)  [unwired: 2 in, 2 out]
            n421 = Implies(1:w886, 2:w887) -> (0:w885:bool)
            n422 = case shown="False" w885 {
              tunnel: w884 -> [w890 w919]
              tunnel: w883 -> [w891 w920]
              tunnel: [w888 w919] -> w882
              tunnel: [w889 w920] -> w881
              frame #0 {
                w897 = 0.1 ("Delay Time (s)")
                # "Backlash"
                n423 = property on="Y Backlash" class="DigNum (strict)"() -> ("Value"=w892:i32)  [unwired: 2 in, 2 out]
                n424 = To Long Integer(number=w892) -> (32bit integer=w915:i32)
                n425 = property on="Y Backlash corr" class="Bool (strict)"("Val(Sgnl)"=FALSE ("Value (Signaling)")) -> ()  [unwired: 2 in, 2 out]
                n426 = Number To Decimal String(number=w892) -> (decimal integer string=w910:string)  [unwired: 1 in]
                n427 = Negate(x=w915) -> (-x=w916:i32)
                n428 = property on="Y Backlash steps/sec" class="DigNum (strict)"() -> ("Value"=w893:i32)  [unwired: 2 in, 2 out]
                n429 = Number To Decimal String(number=w916) -> (decimal integer string=w909:string)  [unwired: 1 in]
                n430 = property on="Y steps/rev" class="DigNum (strict)"() -> ("Value"=w896:u32)  [unwired: 2 in, 2 out]
                n431 = Divide(x=w893, y=w896) -> (x/y=w895:dbl)
                n432 = Number To Fractional String(number=w895) -> (F-format string=w894:string)  [unwired: 3 in]
                n433 = call "Applied Send Command.vi"("error in (no error)"=w890, "Extra"=w894, "Command"=T1."Velocity Setting", "VISA resource name"=w891) -> ("error out"=w899:errorcluster, "VISA resource name out"=w905:refnum<visa-resource-name>)  [unwired: 3 in, 1 out]
                n434 = call "Time Delay41"("error in (no error)"=w899, "Delay Time (s)"=w897) -> ("error out"=w898:errorcluster)  [unwired: 9 in]
                n435 = call "Applied Send Command.vi"("error in (no error)"=w898, "Extra"=w910, "Command"=T1."Distance or Position", "VISA resource name"=w905) -> ("error out"=w904:errorcluster, "VISA resource name out"=w911:refnum<visa-resource-name>)  [unwired: 3 in, 1 out]
                n436 = call "Time Delay38"("error in (no error)"=w904, "Delay Time (s)"=w897) -> ("error out"=w903:errorcluster)  [unwired: 9 in]
                n437 = call "Applied Send Command.vi"("error in (no error)"=w903, "Command"=T1."Feed to Length", "VISA resource name"=w911) -> ("error out"=w902:errorcluster, "VISA resource name out"=w908:refnum<visa-resource-name>)  [unwired: 4 in, 1 out]
                n438 = call "Applied Send Command.vi"("Extra"=w909, "Command"=T1."Distance or Position", "VISA resource name"=w908) -> ("error out"=w901:errorcluster, "VISA resource name out"=w907:refnum<visa-resource-name>)  [unwired: 4 in, 1 out]
                n439 = call "Time Delay39"("error in (no error)"=w902, "Delay Time (s)"=w897) -> ()  [unwired: 9 in, 1 out]
                n440 = call "Time Delay40"("error in (no error)"=w901, "Delay Time (s)"=w897) -> ("error out"=w900:errorcluster)  [unwired: 9 in]
                n441 = call "Applied Send Command.vi"("error in (no error)"=w900, "Command"=T1."Feed to Length", "VISA resource name"=w907) -> ("error out"=w888:errorcluster, "VISA resource name out"=w889:refnum<visa-resource-name>)  [unwired: 4 in, 1 out]
              }
              frame #1 {
              }
            }
          }
        }
        n442 = Multiply(x=360.0, y=w445) -> (x*y=w448:dbl)
        n443 = property on="atan Y/Z" class="DigNum (strict)"("Val(Sgnl)"=w448) -> ()  [unwired: 2 in, 2 out]
      }
      event #1 {
        n444 = event-data() -> ()  [unwired: 1 in, 5 out]
        n445 = property on="Z steps/rev" class="DigNum (strict)"() -> ("Value"=w932:u32)  [unwired: 2 in, 2 out]
        n446 = property on="X steps/rev" class="DigNum (strict)"() -> ("Value"=w941:u32)  [unwired: 2 in, 2 out]
        n447 = property on="Y steps/rev" class="DigNum (strict)"() -> ("Value"=w950:u32)  [unwired: 2 in, 2 out]
        n448 = property on="R steps/rev" class="DigNum (strict)"() -> ("Value"=w923:u32)  [unwired: 2 in, 2 out]
        n449 = property on="R offset deg" class="DigNum (strict)"() -> ("Value"=w921:dbl)  [unwired: 2 in, 2 out]
        n450 = property on="Z offset mm" class="DigNum (strict)"() -> ("Value"=w930:dbl)  [unwired: 2 in, 2 out]
        n451 = property on="X offset mm" class="DigNum (strict)"() -> ("Value"=w939:dbl)  [unwired: 2 in, 2 out]
        n452 = property on="Y offset mm" class="DigNum (strict)"() -> ("Value"=w948:dbl)  [unwired: 2 in, 2 out]
        n453 = To Double Precision Float(number=w923) -> (double precision float=w926:dbl)
        n454 = To Double Precision Float(number=w941) -> (double precision float=w944:dbl)
        n455 = To Double Precision Float(number=w950) -> (double precision float=w953:dbl)
        n456 = property on="Reset Z Position mm" class="DigNum (strict)"() -> ("Value"=w938:dbl)  [unwired: 2 in, 2 out]
        n457 = property on="Reset X Position mm" class="DigNum (strict)"() -> ("Value"=w947:dbl)  [unwired: 2 in, 2 out]
        n458 = property on="Reset Y Position mm" class="DigNum (strict)"() -> ("Value"=w956:dbl)  [unwired: 2 in, 2 out]
        n459 = property on="Reset R Position deg" class="DigNum (strict)"() -> ("Value"=w929:dbl)  [unwired: 2 in, 2 out]
        n460 = Subtract(x=w938, y=w930) -> (x-y=w937:dbl)
        n461 = Subtract(x=w929, y=w921) -> (x-y=w928:dbl)
        n462 = Subtract(x=w947, y=w939) -> (x-y=w946:dbl)
        n463 = Subtract(x=w956, y=w948) -> (x-y=w955:dbl)
        n464 = property on="Z mm/rev" class="DigNum (strict)"() -> ("Value"=w931:dbl)  [unwired: 2 in, 2 out]
        n465 = property on="X mm/rev" class="DigNum (strict)"() -> ("Value"=w940:dbl)  [unwired: 2 in, 2 out]
        n466 = property on="Y mm/rev" class="DigNum (strict)"() -> ("Value"=w949:dbl)  [unwired: 2 in, 2 out]
        n467 = property on="R deg/rev" class="DigNum (strict)"() -> ("Value"=w922:dbl)  [unwired: 2 in, 2 out]
        n468 = Divide(x=w928, y=w922) -> (x/y=w927:dbl)
        n469 = Divide(x=w946, y=w940) -> (x/y=w945:dbl)
        n470 = Divide(x=w955, y=w949) -> (x/y=w954:dbl)
        n471 = Divide(x=w937, y=w931) -> (x/y=w936:dbl)
        n472 = To Double Precision Float(number=w932) -> (double precision float=w935:dbl)
        n473 = Multiply(x=w936, y=w935) -> (x*y=w934:dbl)
        n474 = Multiply(x=w927, y=w926) -> (x*y=w925:dbl)
        n475 = Multiply(x=w945, y=w944) -> (x*y=w943:dbl)
        n476 = Multiply(x=w954, y=w953) -> (x*y=w952:dbl)
        n477 = To Long Integer(number=w934) -> (32bit integer=w933:i32)
        n478 = To Long Integer(number=w925) -> (32bit integer=w924:i32)
        n479 = To Long Integer(number=w943) -> (32bit integer=w942:i32)
        n480 = To Long Integer(number=w952) -> (32bit integer=w951:i32)
        n481 = property on="Reset Z Motor Steps" class="DigNum (strict)"("Val(Sgnl)"=w933) -> ()  [unwired: 2 in, 2 out]
        n482 = property on="Reset R Motor Steps" class="DigNum (strict)"("Val(Sgnl)"=w924) -> ()  [unwired: 2 in, 2 out]
        n483 = property on="Reset X Motor Steps" class="DigNum (strict)"("Val(Sgnl)"=w942) -> ()  [unwired: 2 in, 2 out]
        n484 = property on="Reset Y Motor Steps" class="DigNum (strict)"("Val(Sgnl)"=w951) -> ()  [unwired: 2 in, 2 out]
      }
      event #2 {
        n485 = event-data() -> ()  [unwired: 1 in, 5 out]
        n486 = property on="Z Step SP" class="DigNum (strict)"() -> ("Value"=w973:i32)  [unwired: 2 in, 2 out]
        n487 = property on="Y Step SP" class="DigNum (strict)"() -> ("Value"=w989:i32)  [unwired: 2 in, 2 out]
        n488 = property on="X Step SP" class="DigNum (strict)"() -> ("Value"=w981:i32)  [unwired: 2 in, 2 out]
        n489 = property on="Z steps/rev" class="DigNum (strict)"() -> ("Value"=w1000:u32)  [unwired: 2 in, 2 out]
        n490 = property on="Z steps/rev" class="DigNum (strict)"() -> ("Value"=w971:u32)  [unwired: 2 in, 2 out]
        n491 = property on="R Step SP" class="DigNum (strict)"() -> ("Value"=w965:i32)  [unwired: 2 in, 2 out]
        n492 = property on="Y steps/rev" class="DigNum (strict)"() -> ("Value"=w1012:u32)  [unwired: 2 in, 2 out]
        n493 = property on="Y steps/rev" class="DigNum (strict)"() -> ("Value"=w987:u32)  [unwired: 2 in, 2 out]
        n494 = property on="X steps/rev" class="DigNum (strict)"() -> ("Value"=w1006:u32)  [unwired: 2 in, 2 out]
        n495 = property on="X steps/rev" class="DigNum (strict)"() -> ("Value"=w979:u32)  [unwired: 2 in, 2 out]
        n496 = property on="R steps/rev" class="DigNum (strict)"() -> ("Value"=w994:u32)  [unwired: 2 in, 2 out]
        n497 = property on="R steps/rev" class="DigNum (strict)"() -> ("Value"=w963:u32)  [unwired: 2 in, 2 out]
        n498 = property on="R offset deg" class="DigNum (strict)"() -> ("Value"=w962:dbl)  [unwired: 2 in, 2 out]
        n499 = property on="Z offset mm" class="DigNum (strict)"() -> ("Value"=w970:dbl)  [unwired: 2 in, 2 out]
        n500 = property on="Y offset mm" class="DigNum (strict)"() -> ("Value"=w986:dbl)  [unwired: 2 in, 2 out]
        n501 = property on="X offset mm" class="DigNum (strict)"() -> ("Value"=w978:dbl)  [unwired: 2 in, 2 out]
        n502 = To Double Precision Float(number=w1000) -> (double precision float=w1005:dbl)
        n503 = To Double Precision Float(number=w973) -> (double precision float=w974:dbl)
        n504 = To Double Precision Float(number=w971) -> (double precision float=w977:dbl)
        n505 = To Double Precision Float(number=w994) -> (double precision float=w999:dbl)
        n506 = To Double Precision Float(number=w965) -> (double precision float=w966:dbl)
        n507 = To Double Precision Float(number=w963) -> (double precision float=w969:dbl)
        n508 = To Double Precision Float(number=w989) -> (double precision float=w990:dbl)
        n509 = To Double Precision Float(number=w987) -> (double precision float=w993:dbl)
        n510 = To Double Precision Float(number=w1006) -> (double precision float=w1011:dbl)
        n511 = To Double Precision Float(number=w981) -> (double precision float=w982:dbl)
        n512 = To Double Precision Float(number=w979) -> (double precision float=w985:dbl)
        n513 = Divide(x=w974, y=w977) -> (x/y=w976:dbl)
        n514 = Divide(x=w990, y=w993) -> (x/y=w992:dbl)
        n515 = Divide(x=w982, y=w985) -> (x/y=w984:dbl)
        n516 = Divide(x=w966, y=w969) -> (x/y=w968:dbl)
        n517 = property on="Z Velocity SP step/sec" class="DigNum (strict)"() -> ("Value"=w1002:i32)  [unwired: 2 in, 2 out]
        n518 = property on="Z mm/rev" class="DigNum (strict)"() -> ("Value"=w960:dbl)  [unwired: 2 in, 2 out]
        n519 = property on="Y Velocity SP step/sec" class="DigNum (strict)"() -> ("Value"=w1014:i32)  [unwired: 2 in, 2 out]
        n520 = property on="Y mm/rev" class="DigNum (strict)"() -> ("Value"=w958:dbl)  [unwired: 2 in, 2 out]
        n521 = property on="X Velocity SP step/sec" class="DigNum (strict)"() -> ("Value"=w1008:i32)  [unwired: 2 in, 2 out]
        n522 = property on="X mm/rev" class="DigNum (strict)"() -> ("Value"=w959:dbl)  [unwired: 2 in, 2 out]
        n523 = property on="R Velocity SP step/sec" class="DigNum (strict)"() -> ("Value"=w996:i32)  [unwired: 2 in, 2 out]
        n524 = property on="R deg/rev" class="DigNum (strict)"() -> ("Value"=w961:dbl)  [unwired: 2 in, 2 out]
        n525 = Multiply(x=w976, y=w960) -> (x*y=w975:dbl)
        n526 = Multiply(x=w968, y=w961) -> (x*y=w967:dbl)
        n527 = Multiply(x=w992, y=w958) -> (x*y=w991:dbl)
        n528 = Multiply(x=w984, y=w959) -> (x*y=w983:dbl)
        n529 = To Double Precision Float(number=w1002) -> (double precision float=w1003:dbl)
        n530 = To Double Precision Float(number=w996) -> (double precision float=w997:dbl)
        n531 = To Double Precision Float(number=w1014) -> (double precision float=w1015:dbl)
        n532 = To Double Precision Float(number=w1012) -> (double precision float=w1017:dbl)
        n533 = To Double Precision Float(number=w1008) -> (double precision float=w1009:dbl)
        n534 = Divide(x=w1003, y=w1005) -> (x/y=w1004:dbl)
        n535 = Add(x=w975, y=w970) -> (x+y=w972:dbl)
        n536 = Divide(x=w997, y=w999) -> (x/y=w998:dbl)
        n537 = Add(x=w967, y=w962) -> (x+y=w964:dbl)
        n538 = Divide(x=w1015, y=w1017) -> (x/y=w1016:dbl)
        n539 = Add(x=w991, y=w986) -> (x+y=w988:dbl)
        n540 = Divide(x=w1009, y=w1011) -> (x/y=w1010:dbl)
        n541 = Add(x=w983, y=w978) -> (x+y=w980:dbl)
        n542 = Multiply(x=w1004, y=w960) -> (x*y=w1001:dbl)
        n543 = Multiply(x=w998, y=w961) -> (x*y=w995:dbl)
        n544 = Multiply(x=w1016, y=w958) -> (x*y=w1013:dbl)
        n545 = Multiply(x=w1010, y=w959) -> (x*y=w1007:dbl)
        n546 = property on="Z Position MV mm" class="DigNum (strict)"("Val(Sgnl)"=w972) -> ()  [unwired: 2 in, 2 out]
        n547 = property on="R Position MV deg" class="DigNum (strict)"("Val(Sgnl)"=w964) -> ()  [unwired: 2 in, 2 out]
        n548 = property on="Y Position MV mm" class="DigNum (strict)"("Val(Sgnl)"=w988) -> ()  [unwired: 2 in, 2 out]
        n549 = property on="X Position MV mm" class="DigNum (strict)"("Val(Sgnl)"=w980) -> ()  [unwired: 2 in, 2 out]
        n550 = property on="Z Velocity MV mm/sec" class="DigNum (strict)"("Val(Sgnl)"=w1001) -> ()  [unwired: 2 in, 2 out]
        n551 = property on="Y Velocity MV mm/sec" class="DigNum (strict)"("Val(Sgnl)"=w1013) -> ()  [unwired: 2 in, 2 out]
        n552 = property on="X Velocity MV mm/sec" class="DigNum (strict)"("Val(Sgnl)"=w1007) -> ()  [unwired: 2 in, 2 out]
        n553 = Absolute Value(x=w995) -> (abs(x)=w957:dbl)
        n554 = property on="R Velocity MVdeg/sec" class="DigNum (strict)"("Val(Sgnl)"=w957) -> ()  [unwired: 2 in, 2 out]
      }
      event #3 {
        n555 = event-data() -> ()  [unwired: 1 in, 5 out]
        n556 = property on="R Step PV" class="DigNum (strict)"() -> ("Value"=w1045:i32)  [unwired: 2 in, 2 out]
        n557 = property on="Z steps/rev" class="DigNum (strict)"() -> ("Value"=w1061:u32)  [unwired: 2 in, 2 out]
        n558 = property on="X steps/rev" class="DigNum (strict)"() -> ("Value"=w1088:u32)  [unwired: 2 in, 2 out]
        n559 = property on="Y steps/rev" class="DigNum (strict)"() -> ("Value"=w1074:u32)  [unwired: 2 in, 2 out]
        n560 = property on="X Step PV" class="DigNum (strict)"() -> ("Value"=w1086:i32)  [unwired: 2 in, 2 out]
        n561 = property on="Y Step PV" class="DigNum (strict)"() -> ("Value"=w1072:i32)  [unwired: 2 in, 2 out]
        n562 = property on="Z Step PV" class="DigNum (strict)"() -> ("Value"=w1059:i32)  [unwired: 2 in, 2 out]
        n563 = property on="R steps/rev" class="DigNum (strict)"() -> ("Value"=w1047:u32)  [unwired: 2 in, 2 out]
        n564 = To Double Precision Float(number=w1086) -> (double precision float=w1039:dbl)
        n565 = To Double Precision Float(number=w1072) -> (double precision float=w1038:dbl)
        n566 = To Double Precision Float(number=w1059) -> (double precision float=w1037:dbl)
        n567 = To Double Precision Float(number=w1045) -> (double precision float=w1036:dbl)
        n568 = To Double Precision Float(number=w1061) -> (double precision float=w1058:dbl)
        n569 = To Double Precision Float(number=w1047) -> (double precision float=w1044:dbl)
        n570 = To Double Precision Float(number=w1088) -> (double precision float=w1085:dbl)
        n571 = To Double Precision Float(number=w1074) -> (double precision float=w1029:dbl)
        n572 = property on="X Step SP" class="DigNum (strict)"() -> ("Maximum"=w1092:dbl)  [unwired: 2 in, 2 out]
        n573 = property on="Y Step SP" class="DigNum (strict)"() -> ("Maximum"=w1078:dbl)  [unwired: 2 in, 2 out]
        n574 = property on="Z Step SP" class="DigNum (strict)"() -> ("Maximum"=w1065:dbl)  [unwired: 2 in, 2 out]
        n575 = property on="R Step SP" class="DigNum (strict)"() -> ("Maximum"=w1053:dbl)  [unwired: 2 in, 2 out]
        n576 = property on="Z Scan Length SP steps" class="DigNum (strict)"() -> ("Value"=w1062:i32)  [unwired: 2 in, 2 out]
        n577 = property on="X Scan Length SP steps" class="DigNum (strict)"() -> ("Value"=w1084:i32)  [unwired: 2 in, 2 out]
        n578 = property on="Y Scan Length SP steps" class="DigNum (strict)"() -> ("Value"=w1075:i32)  [unwired: 2 in, 2 out]
        n579 = property on="R Scan Length SP steps" class="DigNum (strict)"() -> ("Value"=w1048:i32)  [unwired: 2 in, 2 out]
        n580 = property on="X Step SP" class="DigNum (strict)"() -> ("Minimum"=w1093:dbl)  [unwired: 2 in, 2 out]
        n581 = property on="Y Step SP" class="DigNum (strict)"() -> ("Minimum"=w1079:dbl)  [unwired: 2 in, 2 out]
        n582 = property on="Z Step SP" class="DigNum (strict)"() -> ("Minimum"=w1066:dbl)  [unwired: 2 in, 2 out]
        n583 = property on="R Step SP" class="DigNum (strict)"() -> ("Minimum"=w1050:dbl)  [unwired: 2 in, 2 out]
        n584 = property on="Z Scan Velocity SP steps/sec" class="DigNum (strict)"() -> ("Value"=w1057:i32)  [unwired: 2 in, 2 out]
        n585 = property on="R Scan Velocity SP steps/sec" class="DigNum (strict)"() -> ("Value"=w1043:i32)  [unwired: 2 in, 2 out]
        n586 = property on="X Scan Velocity SP steps/sec" class="DigNum (strict)"() -> ("Value"=w1089:i32)  [unwired: 2 in, 2 out]
        n587 = property on="Y Scan Velocity SP steps/sec" class="DigNum (strict)"() -> ("Value"=w1071:i32)  [unwired: 2 in, 2 out]
        n588 = Subtract(x=w1093, y=w1039) -> (x-y=w1094:dbl)
        n589 = Subtract(x=w1092, y=w1039) -> (x-y=w1091:dbl)
        n590 = Subtract(x=w1079, y=w1038) -> (x-y=w1080:dbl)
        n591 = Subtract(x=w1078, y=w1038) -> (x-y=w1077:dbl)
        n592 = Subtract(x=w1066, y=w1037) -> (x-y=w1067:dbl)
        n593 = Subtract(x=w1065, y=w1037) -> (x-y=w1064:dbl)
        n594 = Subtract(x=w1050, y=w1036) -> (x-y=w1051:dbl)
        n595 = Subtract(x=w1053, y=w1036) -> (x-y=w1052:dbl)
        n596 = To Double Precision Float(number=w1062) -> (double precision float=w1035:dbl)
        n597 = To Double Precision Float(number=w1048) -> (double precision float=w1033:dbl)
        n598 = To Double Precision Float(number=w1084) -> (double precision float=w1024:dbl)
        n599 = To Double Precision Float(number=w1075) -> (double precision float=w1028:dbl)
        n600 = property on="X Scan Length SP steps" class="DigNum (strict)"("Minimum"=w1094) -> ()  [unwired: 2 in, 2 out]
        n601 = property on="X Scan Length SP steps" class="DigNum (strict)"("Maximum"=w1091) -> ()  [unwired: 2 in, 2 out]
        n602 = property on="Y Scan Length SP steps" class="DigNum (strict)"("Minimum"=w1080) -> ()  [unwired: 2 in, 2 out]
        n603 = property on="Y Scan Length SP steps" class="DigNum (strict)"("Maximum"=w1077) -> ()  [unwired: 2 in, 2 out]
        n604 = property on="Z Scan Length SP steps" class="DigNum (strict)"("Minimum"=w1067) -> ()  [unwired: 2 in, 2 out]
        n605 = property on="Z Scan Length SP steps" class="DigNum (strict)"("Maximum"=w1064) -> ()  [unwired: 2 in, 2 out]
        n606 = property on="R Scan Length SP steps" class="DigNum (strict)"("Minimum"=w1051) -> ()  [unwired: 2 in, 2 out]
        n607 = property on="R Scan Length SP steps" class="DigNum (strict)"("Maximum"=w1052) -> ()  [unwired: 2 in, 2 out]
        n608 = Divide(x=w1035, y=w1058) -> (x/y=w1063:dbl)
        n609 = Divide(x=w1024, y=w1085) -> (x/y=w1083:dbl)
        n610 = Divide(x=w1028, y=w1029) -> (x/y=w1076:dbl)
        n611 = Divide(x=w1033, y=w1044) -> (x/y=w1049:dbl)
        n612 = To Double Precision Float(number=w1057) -> (double precision float=w1034:dbl)
        n613 = To Double Precision Float(number=w1089) -> (double precision float=w1023:dbl)
        n614 = To Double Precision Float(number=w1071) -> (double precision float=w1027:dbl)
        n615 = To Double Precision Float(number=w1043) -> (double precision float=w1032:dbl)
        n616 = property on="Z mm/rev" class="DigNum (strict)"() -> ("Value"=w1060:dbl)  [unwired: 2 in, 2 out]
        n617 = property on="X mm/rev" class="DigNum (strict)"() -> ("Value"=w1087:dbl)  [unwired: 2 in, 2 out]
        n618 = property on="Y mm/rev" class="DigNum (strict)"() -> ("Value"=w1073:dbl)  [unwired: 2 in, 2 out]
        n619 = property on="R deg/rev" class="DigNum (strict)"() -> ("Value"=w1046:dbl)  [unwired: 2 in, 2 out]
        n620 = Multiply(x=w1063, y=w1060) -> (x*y=w1055:dbl)
        n621 = Divide(x=w1035, y=w1034) -> (x/y=w1030:dbl)
        n622 = Divide(x=w1034, y=w1058) -> (x/y=w1056:dbl)
        n623 = Multiply(x=w1049, y=w1046) -> (x*y=w1041:dbl)
        n624 = Divide(x=w1033, y=w1032) -> (x/y=w1031:dbl)
        n625 = Divide(x=w1032, y=w1044) -> (x/y=w1042:dbl)
        n626 = Multiply(x=w1087, y=w1083) -> (x*y=w1081:dbl)
        n627 = Divide(x=w1024, y=w1023) -> (x/y=w1025:dbl)
        n628 = Divide(x=w1023, y=w1085) -> (x/y=w1090:dbl)
        n629 = Multiply(x=w1076, y=w1073) -> (x*y=w1069:dbl)
        n630 = Divide(x=w1028, y=w1027) -> (x/y=w1026:dbl)
        n631 = Divide(x=w1027, y=w1029) -> (x/y=w1070:dbl)
        n632 = Multiply(x=w1060, y=w1056) -> (x*y=w1054:dbl)
        n633 = Multiply(x=w1046, y=w1042) -> (x*y=w1040:dbl)
        n634 = Multiply(x=w1090, y=w1087) -> (x*y=w1082:dbl)
        n635 = Multiply(x=w1073, y=w1070) -> (x*y=w1068:dbl)
        n636 = Absolute Value(x=w1030) -> (abs(x)=→"Z Scan Duration":dbl)
        n637 = Absolute Value(x=w1031) -> (abs(x)=→"R Scan Duration":dbl)
        n638 = Absolute Value(x=w1025) -> (abs(x)=→"X Scan Duration":dbl)
        n639 = Absolute Value(x=w1026) -> (abs(x)=→"Y Scan Duration":dbl)
        n640 = property on="Z Scan length MV mm" class="DigNum (strict)"("Value"=w1055) -> ()  [unwired: 2 in, 2 out]
        n641 = property on="R Scan length MV deg" class="DigNum (strict)"("Value"=w1041) -> ()  [unwired: 2 in, 2 out]
        n642 = property on="X Scan length MV mm" class="DigNum (strict)"("Val(Sgnl)"=w1081) -> ()  [unwired: 2 in, 2 out]
        n643 = property on="Y Scan length MV mm" class="DigNum (strict)"("Value"=w1069) -> ()  [unwired: 2 in, 2 out]
        n644 = Absolute Value(x=w1040) -> (abs(x)=w1022:dbl)
        n645 = property on="Z Scan velocity MV mm/sec" class="DigNum (strict)"("Val(Sgnl)"=w1054) -> ()  [unwired: 2 in, 2 out]
        n646 = property on="X Scan velocity MV mm/sec" class="DigNum (strict)"("Value"=w1082) -> ()  [unwired: 2 in, 2 out]
        n647 = property on="Y Scan velocity MV mm/sec" class="DigNum (strict)"("Val(Sgnl)"=w1068) -> ()  [unwired: 2 in, 2 out]
        n648 = property on="R Scan Velocity SP deg/sec" class="DigNum (strict)"("Val(Sgnl)"=w1022) -> ()  [unwired: 2 in, 2 out]
      }
      event #4 {
        n649 = event-data() -> ()  [unwired: 1 in, 7 out]
        n650 = property on="Y steps/rev" class="DigNum (strict)"() -> ("Value"=w1111:u32)  [unwired: 2 in, 2 out]
        n651 = property on="Y offset mm" class="DigNum (strict)"() -> ("Value"=w1109:dbl)  [unwired: 2 in, 2 out]
        n652 = property on="Y Position SP mm" class="DigNum (strict)"() -> ("Value"=w1108:dbl)  [unwired: 2 in, 2 out]
        n653 = property on="Y Velocity SP step/sec" class="DigNum (strict)"() -> ("Maximum"=w1098:dbl)  [unwired: 2 in, 2 out]
        n654 = property on="Y Velocity SP step/sec" class="DigNum (strict)"() -> ("Minimum"=w1097:dbl)  [unwired: 2 in, 2 out]
        n655 = Subtract(x=w1108, y=w1109) -> (x-y=w1112:dbl)
        n656 = property on="Y Velocity SP mm/sec" class="DigNum (strict)"() -> ("Value"=w1102:dbl)  [unwired: 2 in, 2 out]
        n657 = property on="Y mm/rev" class="DigNum (strict)"() -> ("Value"=w1095:dbl)  [unwired: 2 in, 2 out]
        n658 = Divide(x=w1112, y=w1095) -> (x/y=w1113:dbl)
        n659 = Divide(x=w1102, y=w1095) -> (x/y=w1103:dbl)
        n660 = To Double Precision Float(number=w1111) -> (double precision float=w1096:dbl)
        n661 = Multiply(x=w1113, y=w1096) -> (x*y=w1107:dbl)
        n662 = Multiply(x=w1103, y=w1096) -> (x*y=w1100:dbl)
        n663 = property on="Y Step SP" class="DigNum (strict)"() -> ("Maximum"=w1105:dbl)  [unwired: 2 in, 2 out]
        n664 = property on="Y Step SP" class="DigNum (strict)"() -> ("Minimum"=w1104:dbl)  [unwired: 2 in, 2 out]
        n665 = In Range and Coerce(upper limit=w1098, x=w1100, lower limit=w1097) -> (coerced(x)=w1099:dbl)  [unwired: 1 out]
        n666 = To Long Integer(number=w1099) -> (32bit integer=w1101:i32)
        n667 = In Range and Coerce(upper limit=w1105, x=w1107, lower limit=w1104) -> (coerced(x)=w1106:dbl)  [unwired: 1 out]
        n668 = To Long Integer(number=w1106) -> (32bit integer=w1110:i32)
        n669 = property on="Y Velocity SP step/sec" class="DigNum (strict)"("Val(Sgnl)"=w1101) -> ()  [unwired: 2 in, 2 out]
        n670 = property on="Y Step SP" class="DigNum (strict)"("Val(Sgnl)"=w1110) -> ()  [unwired: 2 in, 2 out]
      }
      event #5 {
        n671 = event-data() -> ()  [unwired: 1 in, 7 out]
        n672 = property on="X steps/rev" class="DigNum (strict)"() -> ("Value"=w1130:u32)  [unwired: 2 in, 2 out]
        n673 = property on="X offset mm" class="DigNum (strict)"() -> ("Value"=w1128:dbl)  [unwired: 2 in, 2 out]
        n674 = property on="X Position SP mm" class="DigNum (strict)"() -> ("Value"=w1127:dbl)  [unwired: 2 in, 2 out]
        n675 = property on="X Velocity SP step/sec" class="DigNum (strict)"() -> ("Maximum"=w1117:dbl)  [unwired: 2 in, 2 out]
        n676 = property on="X Velocity SP step/sec" class="DigNum (strict)"() -> ("Minimum"=w1116:dbl)  [unwired: 2 in, 2 out]
        n677 = Subtract(x=w1127, y=w1128) -> (x-y=w1131:dbl)
        n678 = property on="X Velocity SP mm/sec" class="DigNum (strict)"() -> ("Value"=w1121:dbl)  [unwired: 2 in, 2 out]
        n679 = property on="X mm/rev" class="DigNum (strict)"() -> ("Value"=w1114:dbl)  [unwired: 2 in, 2 out]
        n680 = Divide(x=w1131, y=w1114) -> (x/y=w1132:dbl)
        n681 = Divide(x=w1121, y=w1114) -> (x/y=w1122:dbl)
        n682 = To Double Precision Float(number=w1130) -> (double precision float=w1115:dbl)
        n683 = Multiply(x=w1132, y=w1115) -> (x*y=w1126:dbl)
        n684 = Multiply(x=w1122, y=w1115) -> (x*y=w1119:dbl)
        n685 = property on="X Step SP" class="DigNum (strict)"() -> ("Maximum"=w1124:dbl)  [unwired: 2 in, 2 out]
        n686 = property on="X Step SP" class="DigNum (strict)"() -> ("Minimum"=w1123:dbl)  [unwired: 2 in, 2 out]
        n687 = In Range and Coerce(upper limit=w1117, x=w1119, lower limit=w1116) -> (coerced(x)=w1118:dbl)  [unwired: 1 out]
        n688 = To Long Integer(number=w1118) -> (32bit integer=w1120:i32)
        n689 = In Range and Coerce(upper limit=w1124, x=w1126, lower limit=w1123) -> (coerced(x)=w1125:dbl)  [unwired: 1 out]
        n690 = To Long Integer(number=w1125) -> (32bit integer=w1129:i32)
        n691 = property on="X Velocity SP step/sec" class="DigNum (strict)"("Val(Sgnl)"=w1120) -> ()  [unwired: 2 in, 2 out]
        n692 = property on="X Step SP" class="DigNum (strict)"("Val(Sgnl)"=w1129) -> ()  [unwired: 2 in, 2 out]
      }
      event #6 {
        n693 = event-data() -> ()  [unwired: 1 in, 7 out]
        n694 = property on="Z steps/rev" class="DigNum (strict)"() -> ("Value"=w1147:u32)  [unwired: 2 in, 2 out]
        n695 = property on="Z offset mm" class="DigNum (strict)"() -> ("Value"=w1145:dbl)  [unwired: 2 in, 2 out]
        n696 = property on="Z Position SP mm" class="DigNum (strict)"() -> ("Value"=w1144:dbl)  [unwired: 2 in, 2 out]
        n697 = property on="Z Velocity SP step/sec" class="DigNum (strict)"() -> ("Maximum"=w1134:dbl)  [unwired: 2 in, 2 out]
        n698 = property on="Z Velocity SP step/sec" class="DigNum (strict)"() -> ("Minimum"=w1133:dbl)  [unwired: 2 in, 2 out]
        n699 = Subtract(x=w1144, y=w1145) -> (x-y=w1148:dbl)
        n700 = property on="Z Velocity SP mm/sec" class="DigNum (strict)"() -> ("Value"=w1138:dbl)  [unwired: 2 in, 2 out]
        n701 = property on="Z mm/rev" class="DigNum (strict)"() -> ("Value"=w1150:dbl)  [unwired: 2 in, 2 out]
        n702 = Divide(x=w1148, y=w1150) -> (x/y=w1149:dbl)
        n703 = Divide(x=w1138, y=w1150) -> (x/y=w1139:dbl)
        n704 = To Double Precision Float(number=w1147) -> (double precision float=w1151:dbl)
        n705 = Multiply(x=w1149, y=w1151) -> (x*y=w1143:dbl)
        n706 = Multiply(x=w1139, y=w1151) -> (x*y=w1136:dbl)
        n707 = property on="Z Step SP" class="DigNum (strict)"() -> ("Maximum"=w1141:dbl)  [unwired: 2 in, 2 out]
        n708 = property on="Z Step SP" class="DigNum (strict)"() -> ("Minimum"=w1140:dbl)  [unwired: 2 in, 2 out]
        n709 = In Range and Coerce(upper limit=w1134, x=w1136, lower limit=w1133) -> (coerced(x)=w1135:dbl)  [unwired: 1 out]
        n710 = To Long Integer(number=w1135) -> (32bit integer=w1137:i32)
        n711 = In Range and Coerce(upper limit=w1141, x=w1143, lower limit=w1140) -> (coerced(x)=w1142:dbl)  [unwired: 1 out]
        n712 = To Long Integer(number=w1142) -> (32bit integer=w1146:i32)
        n713 = property on="Z Velocity SP step/sec" class="DigNum (strict)"("Val(Sgnl)"=w1137) -> ()  [unwired: 2 in, 2 out]
        n714 = property on="Z Step SP" class="DigNum (strict)"("Val(Sgnl)"=w1146) -> ()  [unwired: 2 in, 2 out]
      }
      event #7 {
        n715 = event-data() -> ()  [unwired: 1 in, 7 out]
        n716 = property on="R steps/rev" class="DigNum (strict)"() -> ("Value"=w1169:u32)  [unwired: 2 in, 2 out]
        n717 = property on="R offset deg" class="DigNum (strict)"() -> ("Value"=w1167:dbl)  [unwired: 2 in, 2 out]
        n718 = property on="R Position SP deg" class="DigNum (strict)"() -> ("Value"=w1166:dbl)  [unwired: 2 in, 2 out]
        n719 = property on="R Velocity SP step/sec" class="DigNum (strict)"() -> ("Maximum"=w1156:dbl)  [unwired: 2 in, 2 out]
        n720 = property on="R Velocity SP step/sec" class="DigNum (strict)"() -> ("Minimum"=w1155:dbl)  [unwired: 2 in, 2 out]
        n721 = Subtract(x=w1166, y=w1167) -> (x-y=w1170:dbl)
        n722 = property on="R Velocity SP deg/sec" class="DigNum (strict)"() -> ("Value"=w1160:dbl)  [unwired: 2 in, 2 out]
        n723 = property on="R deg/rev" class="DigNum (strict)"() -> ("Value"=w1153:dbl)  [unwired: 2 in, 2 out]
        n724 = Divide(x=w1170, y=w1153) -> (x/y=w1171:dbl)
        n725 = Divide(x=w1160, y=w1153) -> (x/y=w1161:dbl)
        n726 = To Double Precision Float(number=w1169) -> (double precision float=w1154:dbl)
        n727 = Multiply(x=w1171, y=w1154) -> (x*y=w1165:dbl)
        n728 = Multiply(x=w1161, y=w1154) -> (x*y=w1158:dbl)
        n729 = property on="R Step SP" class="DigNum (strict)"() -> ("Maximum"=w1163:dbl)  [unwired: 2 in, 2 out]
        n730 = property on="R Step SP" class="DigNum (strict)"() -> ("Minimum"=w1162:dbl)  [unwired: 2 in, 2 out]
        n731 = Absolute Value(x=w1158) -> (abs(x)=w1152:dbl)
        n732 = In Range and Coerce(upper limit=w1163, x=w1165, lower limit=w1162) -> (coerced(x)=w1164:dbl)  [unwired: 1 out]
        n733 = In Range and Coerce(upper limit=w1156, x=w1152, lower limit=w1155) -> (coerced(x)=w1157:dbl)  [unwired: 1 out]
        n734 = To Long Integer(number=w1164) -> (32bit integer=w1168:i32)
        n735 = To Long Integer(number=w1157) -> (32bit integer=w1159:i32)
        n736 = property on="R Step SP" class="DigNum (strict)"("Val(Sgnl)"=w1168) -> ()  [unwired: 2 in, 2 out]
        n737 = property on="R Velocity SP step/sec" class="DigNum (strict)"("Val(Sgnl)"=w1159) -> ()  [unwired: 2 in, 2 out]
      }
      event #8 {
        n738 = event-data() -> ()  [unwired: 1 in, 7 out]
        n739 = property on="Y steps/rev" class="DigNum (strict)"() -> ("Value"=w1187:u32)  [unwired: 2 in, 2 out]
        n740 = To Double Precision Float(number=w1187) -> (double precision float=w1173:dbl)
        n741 = property on="Y mm/rev" class="DigNum (strict)"() -> ("Value"=w1172:dbl)  [unwired: 2 in, 2 out]
        n742 = property on="Y Scan Length SP mm" class="DigNum (strict)"() -> ("Value"=w1185:dbl)  [unwired: 2 in, 2 out]
        n743 = property on="Y Scan Velocity SP mm/sec" class="DigNum (strict)"() -> ("Value"=w1179:dbl)  [unwired: 2 in, 2 out]
        n744 = property on="Y Scan Velocity SP steps/sec" class="DigNum (strict)"() -> ("Maximum"=w1175:dbl)  [unwired: 2 in, 2 out]
        n745 = property on="Y Scan Velocity SP steps/sec" class="DigNum (strict)"() -> ("Minimum"=w1174:dbl)  [unwired: 2 in, 2 out]
        n746 = Divide(x=w1185, y=w1172) -> (x/y=w1188:dbl)
        n747 = Divide(x=w1179, y=w1172) -> (x/y=w1180:dbl)
        n748 = Multiply(x=w1188, y=w1173) -> (x*y=w1184:dbl)
        n749 = Multiply(x=w1180, y=w1173) -> (x*y=w1177:dbl)
        n750 = property on="Y Step SP" class="DigNum (strict)"() -> ("Maximum"=w1181:dbl)  [unwired: 2 in, 2 out]
        n751 = property on="Y Step SP" class="DigNum (strict)"() -> ("Minimum"=w1182:dbl)  [unwired: 2 in, 2 out]
        n752 = In Range and Coerce(upper limit=w1175, x=w1177, lower limit=w1174) -> (coerced(x)=w1176:dbl)  [unwired: 1 out]
        n753 = To Long Integer(number=w1176) -> (32bit integer=w1178:i32)
        n754 = In Range and Coerce(upper limit=w1181, x=w1184, lower limit=w1182) -> (coerced(x)=w1183:dbl)  [unwired: 1 out]
        n755 = To Long Integer(number=w1183) -> (32bit integer=w1186:i32)
        n756 = property on="Y Scan Velocity SP steps/sec" class="DigNum (strict)"("Val(Sgnl)"=w1178) -> ()  [unwired: 2 in, 2 out]
        n757 = property on="Y Scan Length SP steps" class="DigNum (strict)"("Val(Sgnl)"=w1186) -> ()  [unwired: 2 in, 2 out]
      }
      event #9 {
        n758 = event-data() -> ()  [unwired: 1 in, 7 out]
        n759 = property on="X steps/rev" class="DigNum (strict)"() -> ("Value"=w1204:u32)  [unwired: 2 in, 2 out]
        n760 = To Double Precision Float(number=w1204) -> (double precision float=w1190:dbl)
        n761 = property on="X mm/rev" class="DigNum (strict)"() -> ("Value"=w1189:dbl)  [unwired: 2 in, 2 out]
        n762 = property on="X Scan Length SP mm" class="DigNum (strict)"() -> ("Value"=w1202:dbl)  [unwired: 2 in, 2 out]
        n763 = property on="X Scan Velocity SP mm/sec" class="DigNum (strict)"() -> ("Value"=w1196:dbl)  [unwired: 2 in, 2 out]
        n764 = property on="X Scan Velocity SP steps/sec" class="DigNum (strict)"() -> ("Maximum"=w1192:dbl)  [unwired: 2 in, 2 out]
        n765 = property on="X Scan Velocity SP steps/sec" class="DigNum (strict)"() -> ("Minimum"=w1191:dbl)  [unwired: 2 in, 2 out]
        n766 = Divide(x=w1202, y=w1189) -> (x/y=w1205:dbl)
        n767 = Divide(x=w1196, y=w1189) -> (x/y=w1197:dbl)
        n768 = Multiply(x=w1205, y=w1190) -> (x*y=w1201:dbl)
        n769 = Multiply(x=w1197, y=w1190) -> (x*y=w1194:dbl)
        n770 = property on="X Step SP" class="DigNum (strict)"() -> ("Maximum"=w1198:dbl)  [unwired: 2 in, 2 out]
        n771 = property on="X Step SP" class="DigNum (strict)"() -> ("Minimum"=w1199:dbl)  [unwired: 2 in, 2 out]
        n772 = In Range and Coerce(upper limit=w1192, x=w1194, lower limit=w1191) -> (coerced(x)=w1193:dbl)  [unwired: 1 out]
        n773 = To Long Integer(number=w1193) -> (32bit integer=w1195:i32)
        n774 = In Range and Coerce(upper limit=w1198, x=w1201, lower limit=w1199) -> (coerced(x)=w1200:dbl)  [unwired: 1 out]
        n775 = To Long Integer(number=w1200) -> (32bit integer=w1203:i32)
        n776 = property on="X Scan Velocity SP steps/sec" class="DigNum (strict)"("Val(Sgnl)"=w1195) -> ()  [unwired: 2 in, 2 out]
        n777 = property on="X Scan Length SP steps" class="DigNum (strict)"("Val(Sgnl)"=w1203) -> ()  [unwired: 2 in, 2 out]
      }
      event #10 {
        n778 = event-data() -> ()  [unwired: 1 in, 7 out]
        n779 = property on="Z steps/rev" class="DigNum (strict)"() -> ("Value"=w1221:u32)  [unwired: 2 in, 2 out]
        n780 = To Double Precision Float(number=w1221) -> (double precision float=w1207:dbl)
        n781 = property on="Z mm/rev" class="DigNum (strict)"() -> ("Value"=w1206:dbl)  [unwired: 2 in, 2 out]
        n782 = property on="Z Scan Length SP mm" class="DigNum (strict)"() -> ("Value"=w1219:dbl)  [unwired: 2 in, 2 out]
        n783 = property on="Z Scan Velocity SP mm/sec" class="DigNum (strict)"() -> ("Value"=w1213:dbl)  [unwired: 2 in, 2 out]
        n784 = property on="Z Scan Velocity SP steps/sec" class="DigNum (strict)"() -> ("Maximum"=w1209:dbl)  [unwired: 2 in, 2 out]
        n785 = property on="Z Scan Velocity SP steps/sec" class="DigNum (strict)"() -> ("Minimum"=w1208:dbl)  [unwired: 2 in, 2 out]
        n786 = Divide(x=w1219, y=w1206) -> (x/y=w1222:dbl)
        n787 = Divide(x=w1213, y=w1206) -> (x/y=w1214:dbl)
        n788 = Multiply(x=w1222, y=w1207) -> (x*y=w1218:dbl)
        n789 = Multiply(x=w1214, y=w1207) -> (x*y=w1211:dbl)
        n790 = property on="Z Step SP" class="DigNum (strict)"() -> ("Maximum"=w1215:dbl)  [unwired: 2 in, 2 out]
        n791 = property on="Z Step SP" class="DigNum (strict)"() -> ("Minimum"=w1216:dbl)  [unwired: 2 in, 2 out]
        n792 = In Range and Coerce(upper limit=w1209, x=w1211, lower limit=w1208) -> (coerced(x)=w1210:dbl)  [unwired: 1 out]
        n793 = To Long Integer(number=w1210) -> (32bit integer=w1212:i32)
        n794 = In Range and Coerce(upper limit=w1215, x=w1218, lower limit=w1216) -> (coerced(x)=w1217:dbl)  [unwired: 1 out]
        n795 = To Long Integer(number=w1217) -> (32bit integer=w1220:i32)
        n796 = property on="Z Scan Velocity SP steps/sec" class="DigNum (strict)"("Val(Sgnl)"=w1212) -> ()  [unwired: 2 in, 2 out]
        n797 = property on="Z Scan Length SP steps" class="DigNum (strict)"("Val(Sgnl)"=w1220) -> ()  [unwired: 2 in, 2 out]
      }
      event #11 {
        n798 = event-data() -> ()  [unwired: 1 in, 7 out]
        n799 = property on="R steps/rev" class="DigNum (strict)"() -> ("Value"=w1239:u32)  [unwired: 2 in, 2 out]
        n800 = To Double Precision Float(number=w1239) -> (double precision float=w1225:dbl)
        n801 = property on="R Velocity SP step/sec" class="DigNum (strict)"() -> ("Maximum"=w1227:dbl)  [unwired: 2 in, 2 out]
        n802 = property on="R Scan Length SP deg" class="DigNum (strict)"() -> ("Value"=w1237:dbl)  [unwired: 2 in, 2 out]
        n803 = property on="R deg/rev" class="DigNum (strict)"() -> ("Value"=w1224:dbl)  [unwired: 2 in, 2 out]
        n804 = property on="R Scan Velocity SP steps/sec" class="DigNum (strict)"() -> ("Minimum"=w1226:dbl)  [unwired: 2 in, 2 out]
        n805 = property on="R Scan Velocity SP deg/sec" class="DigNum (strict)"() -> ("Value"=w1231:dbl)  [unwired: 2 in, 2 out]
        n806 = Divide(x=w1237, y=w1224) -> (x/y=w1240:dbl)
        n807 = Multiply(x=w1240, y=w1225) -> (x*y=w1236:dbl)
        n808 = Divide(x=w1231, y=w1224) -> (x/y=w1232:dbl)
        n809 = property on="R Step SP" class="DigNum (strict)"() -> ("Maximum"=w1233:dbl)  [unwired: 2 in, 2 out]
        n810 = property on="R Step SP" class="DigNum (strict)"() -> ("Minimum"=w1234:dbl)  [unwired: 2 in, 2 out]
        n811 = Multiply(x=w1232, y=w1225) -> (x*y=w1229:dbl)
        n812 = Absolute Value(x=w1229) -> (abs(x)=w1223:dbl)
        n813 = In Range and Coerce(upper limit=w1233, x=w1236, lower limit=w1234) -> (coerced(x)=w1235:dbl)  [unwired: 1 out]
        n814 = To Long Integer(number=w1235) -> (32bit integer=w1238:i32)
        n815 = In Range and Coerce(upper limit=w1227, x=w1223, lower limit=w1226) -> (coerced(x)=w1228:dbl)  [unwired: 1 out]
        n816 = To Long Integer(number=w1228) -> (32bit integer=w1230:i32)
        n817 = property on="R Scan Length SP steps" class="DigNum (strict)"("Val(Sgnl)"=w1238) -> ()  [unwired: 2 in, 2 out]
        n818 = property on="R Scan Velocity SP steps/sec" class="DigNum (strict)"("Val(Sgnl)"=w1230) -> ()  [unwired: 2 in, 2 out]
      }
      event #12 {
        n819 = event-data() -> ()  [unwired: 1 in, 7 out]
        n820 = flat-sequence {
          tunnel: w1247 -> [w1257]
          tunnel: w1248 -> [w1258]
          tunnel: [w1258] -> w1244
          tunnel: [w1257] -> w1243
          tunnel: [w1261] -> w1246
          tunnel: [w1260] -> w1245
          tunnel: w1244 -> [w1263]
          tunnel: w1243 -> [w1262]
          tunnel: [w1284] -> w1250
          tunnel: [w1279] -> w1249
          tunnel: w1246 -> [w1283]
          tunnel: w1245 -> [w1282]
          tunnel: [w1278] -> w1242
          tunnel: [w1295] -> w1252
          tunnel: [w1290] -> w1251
          tunnel: w1250 -> [w1293]
          tunnel: w1249 -> [w1294]
          tunnel: w1242 -> [w1291]
          tunnel: [w1291] -> w1241
          tunnel: [w1298] -> w1253
          tunnel: [w1301] -> w1254
          tunnel: w1252 -> [w1300]
          tunnel: w1251 -> [w1299]
          tunnel: w1241 -> [w1302]
          frame #0 {
            n821 = property on="Scan Go" class="Bool"("DisabledEnum"=T2."Disabled and Grayed Out" ("Disabled")) -> ()  [unwired: 2 in, 2 out]
            n822 = property on="Y Go" class="Bool"("DisabledEnum"=T2."Disabled and Grayed Out" ("Disabled")) -> ()  [unwired: 2 in, 2 out]
          }
          frame #1 {
            n823 = property on="Y Step SP" class="DigNum (strict)"() -> ("Value"=w1271:i32)  [unwired: 2 in, 2 out]
            n824 = property on="Y Step PV" class="DigNum (strict)"() -> ("Value"=w1270:i32)  [unwired: 2 in, 2 out]
            n825 = property on="Y Backlash" class="DigNum (strict)"() -> ("Value"=w1259:i32)  [unwired: 2 in, 2 out]
            n826 = Subtract(x=w1271, y=w1270) -> (x-y=w1269:i32)
            n827 = Sign(1:w1259) -> (0:w1267:i32)
            n828 = Sign(1:w1269) -> (0:w1268:i32)
            n829 = Multiply(x=w1268, y=w1267) -> (x*y=w1266:i32)
            n830 = Equal?(x=w1266, y=1) -> (x = y?=w1264:bool)
            n831 = case shown="False" w1264 {
              tunnel: w1263 -> [w1274 w1276]
              tunnel: w1262 -> [w1273 w1275]
              tunnel: [w1273 w1275] -> w1261
              tunnel: [w1274 w1276] -> w1260
              frame #0 {
                n832 = property on="Y Backlash corr" class="Bool (strict)"("Val(Sgnl)"=FALSE ("Value (Signaling)")) -> ()  [unwired: 2 in, 2 out]
              }
              frame #1 {
                n833 = property on="Y Backlash corr" class="Bool (strict)"("Val(Sgnl)"=TRUE ("Value (Signaling)")) -> ()  [unwired: 2 in, 2 out]
              }
            }
          }
          frame #2 {
            w1278 = 0.1 ("Delay Time (s)")
            # "Velocity Setting"
            n834 = property on="Y Velocity SP step/sec" class="DigNum (strict)"() -> ("Value"=w1287:i32)  [unwired: 2 in, 2 out]
            n835 = Number To Decimal String(number=w1287) -> ()  [unwired: 1 in, 1 out]
            n836 = property on="Y steps/rev" class="DigNum (strict)"() -> ("Value"=w1286:u32)  [unwired: 2 in, 2 out]
            n837 = Divide(x=w1287, y=w1286) -> (x/y=w1288:dbl)
            n838 = Number To Fractional String(number=w1288) -> (F-format string=w1281:string)  [unwired: 3 in]
            n839 = call "Applied Send Command.vi"("error in (no error)"=w1283, "Extra"=w1281, "Command"=T1."Velocity Setting", "VISA resource name"=w1282) -> ("error out"=w1280:errorcluster, "VISA resource name out"=w1284:refnum<visa-resource-name>)  [unwired: 3 in, 1 out]
            n840 = call "Time Delay22"("error in (no error)"=w1280, "Delay Time (s)"=w1278) -> ("error out"=w1279:errorcluster)  [unwired: 9 in]
          }
          frame #3 {
            # "Move to Abs Position"
            n841 = property on="Y Step SP" class="DigNum (strict)"() -> ("Value"=w1297:i32)  [unwired: 2 in, 2 out]
            n842 = Number To Decimal String(number=w1297) -> (decimal integer string=w1292:string)  [unwired: 1 in]
            n843 = call "Applied Send Command.vi"("error in (no error)"=w1294, "Extra"=w1292, "Command"=T1."Distance or Position", "VISA resource name"=w1293) -> ("error out"=w1289:errorcluster, "VISA resource name out"=w1295:refnum<visa-resource-name>)  [unwired: 3 in, 1 out]
            n844 = call "Time Delay"("error in (no error)"=w1289, "Delay Time (s)"=w1291) -> ("error out"=w1290:errorcluster)  [unwired: 9 in]
          }
          frame #4 {
            n845 = call "Applied Send Command.vi"("error in (no error)"=w1299, "Command"=T1."Feed to Position", "VISA resource name"=w1300) -> ("error out"=w1303:errorcluster, "VISA resource name out"=w1301:refnum<visa-resource-name>)  [unwired: 4 in, 1 out]
            n846 = call "Time Delay23"("error in (no error)"=w1303, "Delay Time (s)"=w1302) -> ("error out"=w1298:errorcluster)  [unwired: 9 in]
          }
        }
      }
      event #13 {
        n847 = event-data() -> ()  [unwired: 1 in, 7 out]
        n848 = flat-sequence {
          tunnel: w1309 -> [w1321]
          tunnel: w1310 -> [w1322]
          tunnel: [w1322] -> w1312
          tunnel: [w1321] -> w1311
          tunnel: [w1325] -> w1314
          tunnel: [w1324] -> w1313
          tunnel: w1312 -> [w1327]
          tunnel: w1311 -> [w1326]
          tunnel: [w1345] -> w1316
          tunnel: [w1343] -> w1315
          tunnel: w1314 -> [w1346]
          tunnel: w1313 -> [w1347]
          tunnel: [w1342] -> w1306
          tunnel: [w1356] -> w1318
          tunnel: [w1355] -> w1317
          tunnel: w1316 -> [w1357]
          tunnel: w1315 -> [w1359]
          tunnel: w1306 -> [w1353]
          tunnel: [w1353] -> w1305
          tunnel: [w1368] -> w1308
          tunnel: [w1364] -> w1307
          tunnel: w1318 -> [w1365]
          tunnel: w1317 -> [w1362]
          tunnel: w1305 -> [w1367]
          frame #0 {
            n849 = property on="Scan Go" class="Bool"("DisabledEnum"=T2."Disabled and Grayed Out" ("Disabled")) -> ()  [unwired: 2 in, 2 out]
            n850 = property on="Z Go" class="Bool"("DisabledEnum"=T2."Disabled and Grayed Out" ("Disabled")) -> ()  [unwired: 2 in, 2 out]
          }
          frame #1 {
            n851 = property on="Z Step SP" class="DigNum (strict)"() -> ("Value"=w1335:i32)  [unwired: 2 in, 2 out]
            n852 = property on="Z Step PV" class="DigNum (strict)"() -> ("Value"=w1334:i32)  [unwired: 2 in, 2 out]
            n853 = property on="Z Backlash" class="DigNum (strict)"() -> ("Value"=w1323:i32)  [unwired: 2 in, 2 out]
            n854 = Subtract(x=w1335, y=w1334) -> (x-y=w1333:i32)
            n855 = Sign(1:w1323) -> (0:w1331:i32)
            n856 = Sign(1:w1333) -> (0:w1332:i32)
            n857 = Multiply(x=w1332, y=w1331) -> (x*y=w1330:i32)
            n858 = Equal?(x=w1330, y=1) -> (x = y?=w1328:bool)
            n859 = case shown="True" w1328 {
              tunnel: w1327 -> [w1338 w1340]
              tunnel: w1326 -> [w1337 w1339]
              tunnel: [w1337 w1339] -> w1325
              tunnel: [w1338 w1340] -> w1324
              frame #0 {
                n860 = property on="Z Backlash corr" class="Bool (strict)"("Val(Sgnl)"=FALSE ("Value (Signaling)")) -> ()  [unwired: 2 in, 2 out]
              }
              frame #1 {
                n861 = property on="Z Backlash corr" class="Bool (strict)"("Val(Sgnl)"=TRUE ("Value (Signaling)")) -> ()  [unwired: 2 in, 2 out]
              }
            }
          }
          frame #2 {
            w1342 = 0.1 ("Delay Time (s)")
            n862 = property on="Z Velocity SP step/sec" class="DigNum (strict)"() -> ("Value"=w1349:i32)  [unwired: 2 in, 2 out]
            n863 = property on="Z steps/rev" class="DigNum (strict)"() -> ("Value"=w1348:u32)  [unwired: 2 in, 2 out]
            n864 = Divide(x=w1349, y=w1348) -> (x/y=w1350:dbl)
            n865 = Number To Fractional String(number=w1350) -> (F-format string=w1351:string)  [unwired: 3 in]
            n866 = call "Applied Send Command.vi"("error in (no error)"=w1346, "Extra"=w1351, "Command"=T1."Velocity Setting", "VISA resource name"=w1347) -> ("error out"=w1344:errorcluster, "VISA resource name out"=w1345:refnum<visa-resource-name>)  [unwired: 3 in, 1 out]
            n867 = call "Time Delay52"("error in (no error)"=w1344, "Delay Time (s)"=w1342) -> ("error out"=w1343:errorcluster)  [unwired: 9 in]
          }
          frame #3 {
            # "Move to Abs Position"
            n868 = property on="Z Step SP" class="DigNum (strict)"() -> ("Value"=w1361:i32)  [unwired: 2 in, 2 out]
            n869 = Number To Decimal String(number=w1361) -> (decimal integer string=w1358:string)  [unwired: 1 in]
            n870 = call "Applied Send Command.vi"("error in (no error)"=w1359, "Extra"=w1358, "Command"=T1."Distance or Position", "VISA resource name"=w1357) -> ("error out"=w1354:errorcluster, "VISA resource name out"=w1356:refnum<visa-resource-name>)  [unwired: 3 in, 1 out]
            n871 = call "Time Delay51"("error in (no error)"=w1354, "Delay Time (s)"=w1353) -> ("error out"=w1355:errorcluster)  [unwired: 9 in]
          }
          frame #4 {
            n872 = call "Applied Send Command.vi"("error in (no error)"=w1362, "Command"=T1."Feed to Position", "VISA resource name"=w1365) -> ("error out"=w1363:errorcluster, "VISA resource name out"=w1364:refnum<visa-resource-name>)  [unwired: 4 in, 1 out]
            n873 = call "Time Delay28"("error in (no error)"=w1363, "Delay Time (s)"=w1367) -> ("error out"=w1368:errorcluster)  [unwired: 9 in]
          }
        }
      }
      event #14 {
        n874 = event-data() -> ()  [unwired: 1 in, 7 out]
        n875 = flat-sequence {
          tunnel: w1373 -> [w1385]
          tunnel: w1374 -> [w1386]
          tunnel: [w1386] -> w1376
          tunnel: [w1385] -> w1375
          tunnel: [w1389] -> w1378
          tunnel: [w1388] -> w1377
          tunnel: w1376 -> [w1391]
          tunnel: w1375 -> [w1390]
          tunnel: [w1407] -> w1380
          tunnel: [w1408] -> w1379
          tunnel: w1378 -> [w1409]
          tunnel: w1377 -> [w1410]
          tunnel: [w1406] -> w1370
          tunnel: [w1420] -> w1382
          tunnel: [w1418] -> w1381
          tunnel: w1380 -> [w1419]
          tunnel: w1379 -> [w1421]
          tunnel: w1370 -> [w1416]
          tunnel: [w1416] -> w1369
          tunnel: [w1431] -> w1372
          tunnel: [w1427] -> w1371
          tunnel: w1382 -> [w1428]
          tunnel: w1381 -> [w1425]
          tunnel: w1369 -> [w1430]
          frame #0 {
            n876 = property on="Scan Go" class="Bool"("DisabledEnum"=T2."Disabled and Grayed Out" ("Disabled")) -> ()  [unwired: 2 in, 2 out]
            n877 = property on="R Go" class="Bool"("DisabledEnum"=T2."Disabled and Grayed Out" ("Disabled")) -> ()  [unwired: 2 in, 2 out]
          }
          frame #1 {
            n878 = property on="R Step SP" class="DigNum (strict)"() -> ("Value"=w1399:i32)  [unwired: 2 in, 2 out]
            n879 = property on="R Step PV" class="DigNum (strict)"() -> ("Value"=w1398:i32)  [unwired: 2 in, 2 out]
            n880 = property on="R Backlash" class="DigNum (strict)"() -> ("Value"=w1387:i32)  [unwired: 2 in, 2 out]
            n881 = Subtract(x=w1399, y=w1398) -> (x-y=w1397:i32)
            n882 = Sign(1:w1387) -> (0:w1395:i32)
            n883 = Sign(1:w1397) -> (0:w1396:i32)
            n884 = Multiply(x=w1396, y=w1395) -> (x*y=w1394:i32)
            n885 = Equal?(x=w1394, y=1) -> (x = y?=w1392:bool)
            n886 = case shown="True" w1392 {
              tunnel: w1391 -> [w1402 w1404]
              tunnel: w1390 -> [w1401 w1403]
              tunnel: [w1401 w1403] -> w1389
              tunnel: [w1402 w1404] -> w1388
              frame #0 {
                n887 = property on="R Backlash corr" class="Bool (strict)"("Val(Sgnl)"=FALSE ("Value (Signaling)")) -> ()  [unwired: 2 in, 2 out]
              }
              frame #1 {
                n888 = property on="R Backlash corr" class="Bool (strict)"("Val(Sgnl)"=TRUE ("Value (Signaling)")) -> ()  [unwired: 2 in, 2 out]
              }
            }
          }
          frame #2 {
            w1406 = 0.1 ("Delay Time (s)")
            # "Velocity Setting"
            n889 = property on="R Velocity SP step/sec" class="DigNum (strict)"() -> ("Value"=w1412:i32)  [unwired: 2 in, 2 out]
            n890 = property on="R steps/rev" class="DigNum (strict)"() -> ("Value"=w1411:u32)  [unwired: 2 in, 2 out]
            n891 = Divide(x=w1412, y=w1411) -> (x/y=w1413:dbl)
            n892 = Number To Fractional String(number=w1413) -> (F-format string=w1414:string)  [unwired: 3 in]
            n893 = call "Applied Send Command.vi"("error in (no error)"=w1409, "Extra"=w1414, "VISA resource name"=w1410) -> ("error out"=w1415:errorcluster, "VISA resource name out"=w1407:refnum<visa-resource-name>)  [unwired: 4 in, 1 out]
            n894 = call "Time Delay54"("error in (no error)"=w1415, "Delay Time (s)"=w1406) -> ("error out"=w1408:errorcluster)  [unwired: 9 in]
          }
          frame #3 {
            # "Distance/Position"
            n895 = property on="R Step SP" class="DigNum (strict)"() -> ("Value"=w1422:i32)  [unwired: 2 in, 2 out]
            n896 = Number To Decimal String(number=w1422) -> (decimal integer string=w1423:string)  [unwired: 1 in]
            n897 = call "Applied Send Command.vi"("error in (no error)"=w1421, "Extra"=w1423, "Command"=T1."Distance or Position", "VISA resource name"=w1419) -> ("error out"=w1417:errorcluster, "VISA resource name out"=w1420:refnum<visa-resource-name>)  [unwired: 3 in, 1 out]
            n898 = call "Time Delay53"("error in (no error)"=w1417, "Delay Time (s)"=w1416) -> ("error out"=w1418:errorcluster)  [unwired: 9 in]
          }
          frame #4 {
            # "Feed to Position"
            n899 = call "Applied Send Command.vi"("error in (no error)"=w1425, "Command"=T1."Feed to Position", "VISA resource name"=w1428) -> ("error out"=w1426:errorcluster, "VISA resource name out"=w1427:refnum<visa-resource-name>)  [unwired: 4 in, 1 out]
            n900 = call "Time Delay29"("error in (no error)"=w1426, "Delay Time (s)"=w1430) -> ("error out"=w1431:errorcluster)  [unwired: 9 in]
          }
        }
      }
      event #15 {
        n901 = event-data() -> ()  [unwired: 1 in, 7 out]
        n902 = flat-sequence {
          tunnel: [w1447] -> w1443
          tunnel: [w1446] -> w1442
          tunnel: w1441 -> [w1447]
          tunnel: w1440 -> [w1446]
          tunnel: [w1452] -> w1445
          tunnel: [w1451] -> w1444
          tunnel: w1443 -> [w1454]
          tunnel: w1442 -> [w1453]
          tunnel: [w1473] -> w1437
          tunnel: [w1470] -> w1435
          tunnel: w1445 -> [w1474]
          tunnel: w1444 -> [w1475]
          tunnel: [w1469] -> w1433
          tunnel: w1437 -> [w1482]
          tunnel: [w1481] -> w1436
          tunnel: w1435 -> [w1483]
          tunnel: [w1484] -> w1434
          tunnel: w1433 -> [w1480]
          tunnel: [w1480] -> w1432
          tunnel: w1436 -> [w1494]
          tunnel: w1434 -> [w1493]
          tunnel: [w1492] -> w1439
          tunnel: [w1491] -> w1438
          tunnel: w1432 -> [w1489]
          frame #0 {
            n903 = property on="Scan Go" class="Bool"("DisabledEnum"=T2."Disabled and Grayed Out" ("Disabled")) -> ()  [unwired: 2 in, 2 out]
            n904 = property on="X Go" class="Bool"("DisabledEnum"=T2."Disabled and Grayed Out" ("Disabled")) -> ()  [unwired: 2 in, 2 out]
          }
          frame #1 {
            n905 = property on="X Step SP" class="DigNum (strict)"() -> ("Value"=w1462:i32)  [unwired: 2 in, 2 out]
            n906 = property on="X Step PV" class="DigNum (strict)"() -> ("Value"=w1461:i32)  [unwired: 2 in, 2 out]
            n907 = property on="X Backlash" class="DigNum (strict)"() -> ("Value"=w1450:i32)  [unwired: 2 in, 2 out]
            n908 = Subtract(x=w1462, y=w1461) -> (x-y=w1460:i32)
            n909 = Sign(1:w1450) -> (0:w1458:i32)
            n910 = Sign(1:w1460) -> (0:w1459:i32)
            n911 = Multiply(x=w1459, y=w1458) -> (x*y=w1457:i32)
            n912 = Equal?(x=w1457, y=1) -> (x = y?=w1455:bool)
            n913 = case shown="True" w1455 {
              tunnel: w1454 -> [w1465 w1467]
              tunnel: w1453 -> [w1464 w1466]
              tunnel: [w1464 w1466] -> w1452
              tunnel: [w1465 w1467] -> w1451
              frame #0 {
                n914 = property on="X Backlash corr" class="Bool (strict)"("Val(Sgnl)"=FALSE ("Value (Signaling)")) -> ()  [unwired: 2 in, 2 out]
              }
              frame #1 {
                n915 = property on="X Backlash corr" class="Bool (strict)"("Val(Sgnl)"=TRUE ("Value (Signaling)")) -> ()  [unwired: 2 in, 2 out]
              }
            }
          }
          frame #2 {
            w1469 = 0.1 ("Delay Time (s)")
            n916 = property on="X Velocity SP step/sec" class="DigNum (strict)"() -> ("Value"=w1472:i32)  [unwired: 2 in, 2 out]
            n917 = property on="X steps/rev" class="DigNum (strict)"() -> ("Value"=w1476:u32)  [unwired: 2 in, 2 out]
            n918 = Divide(x=w1472, y=w1476) -> (x/y=w1477:dbl)
            n919 = Number To Fractional String(number=w1477) -> (F-format string=w1478:string)  [unwired: 3 in]
            n920 = call "Applied Send Command.vi"("error in (no error)"=w1474, "Extra"=w1478, "Command"=T1."Velocity Setting", "VISA resource name"=w1475) -> ("error out"=w1471:errorcluster, "VISA resource name out"=w1473:refnum<visa-resource-name>)  [unwired: 3 in, 1 out]
            n921 = call "Time Delay14"("error in (no error)"=w1471, "Delay Time (s)"=w1469) -> ("error out"=w1470:errorcluster)  [unwired: 9 in]
          }
          frame #3 {
            # "Distance/Position"
            n922 = property on="X Step SP" class="DigNum (strict)"() -> ("Value"=w1485:i32)  [unwired: 2 in, 2 out]
            n923 = Number To Decimal String(number=w1485) -> (decimal integer string=w1487:string)  [unwired: 1 in]
            n924 = call "Applied Send Command.vi"("error in (no error)"=w1483, "Extra"=w1487, "Command"=T1."Distance or Position", "VISA resource name"=w1482) -> ("error out"=w1486:errorcluster, "VISA resource name out"=w1481:refnum<visa-resource-name>)  [unwired: 3 in, 1 out]
            n925 = call "Time Delay31"("error in (no error)"=w1486, "Delay Time (s)"=w1480) -> ("error out"=w1484:errorcluster)  [unwired: 9 in]
          }
          frame #4 {
            # "Feed to Position"
            n926 = call "Applied Send Command.vi"("error in (no error)"=w1493, "Command"=T1."Feed to Position", "VISA resource name"=w1494) -> ("error out"=w1490:errorcluster, "VISA resource name out"=w1492:refnum<visa-resource-name>)  [unwired: 4 in, 1 out]
            n927 = call "Time Delay15"("error in (no error)"=w1490, "Delay Time (s)"=w1489) -> ("error out"=w1491:errorcluster)  [unwired: 9 in]
          }
        }
      }
      event #16 {
        n928 = event-data() -> ()  [unwired: 1 in, 7 out]
        n929 = flat-sequence {
          tunnel: [w1511] -> w1503
          tunnel: [w1522] -> w1502
          tunnel: w1501 -> [w1519]
          tunnel: w1500 -> [w1518]
          tunnel: w1503 -> [w1529]
          tunnel: w1502 -> [w1528]
          tunnel: [w1529] -> w1497
          tunnel: [w1528] -> w1496
          tunnel: [w1531] -> w1498
          tunnel: [w1532] -> w1499
          tunnel: w1497 -> [w1532]
          tunnel: w1496 -> [w1531]
          frame #0 {
            # "VELOCITY"
            n930 = property on="X steps/rev" class="DigNum (strict)"() -> ("Value"=w1504:u32)  [unwired: 2 in, 2 out]
            n931 = property on="X Scan Velocity SP steps/sec" class="DigNum (strict)"() -> ("Value"=w1505:i32)  [unwired: 2 in, 2 out]
            n932 = Divide(x=w1505, y=w1504) -> (x/y=w1506:dbl)
            n933 = Number To Fractional String(number=w1506) -> (F-format string=w1520:string)  [unwired: 3 in]
            n934 = call "Applied Send Command.vi"("error in (no error)"=w1518, "Extra"=w1520, "Command"=T1."Velocity Setting", "VISA resource name"=w1519) -> ("error out"=w1507:errorcluster, "VISA resource name out"=w1508:refnum<visa-resource-name>)  [unwired: 3 in, 1 out]
            n935 = call "Time Delay9"("error in (no error)"=w1507) -> ("error out"=w1509:errorcluster)  [unwired: 10 in]
            n936 = call "Applied Send Command.vi"("error in (no error)"=w1509, "Extra"="", "Command"=T1."Velocity Setting", "VISA resource name"=w1508) -> ("error out"=w1510:errorcluster, "read buffer"=w1515:string, "VISA resource name out"=w1511:refnum<visa-resource-name>)  [unwired: 3 in]
            n937 = call "Time Delay10"("error in (no error)"=w1510) -> ("error out"=w1522:errorcluster)  [unwired: 10 in]
            n938 = Fract/Exp String To Number(string=w1515, offset=3) -> (number=w1513:dbl)  [unwired: 2 in, 1 out]
            n939 = Multiply(x=w1513, y=w1504) -> (x*y=w1512:dbl)
            n940 = property on="X velocity PV step/sec" class="DigNum (strict)"("Val(Sgnl)"=w1512) -> ()  [unwired: 2 in, 2 out]
          }
          frame #1 {
            n941 = property on="X Scan" class="Bool (strict)"("Val(Sgnl)"=TRUE ("Slew Ready 2")) -> ()  [unwired: 2 in, 2 out]
            n942 = property on="Scan Cancel" class="Bool"("DisabledEnum"=T2."Enabled" ("Disabled")) -> ()  [unwired: 2 in, 2 out]
            n943 = property on="Scan Go" class="Bool"("DisabledEnum"=T2."Enabled" ("Disabled")) -> ()  [unwired: 2 in, 2 out]
            n944 = property on="X Scan Length SP steps" class="DigNum (strict)"("DisabledEnum"=T2."Disabled and Grayed Out" ("Disabled")) -> ()  [unwired: 2 in, 2 out]
            n945 = property on="X Scan Velocity SP steps/sec" class="DigNum (strict)"("DisabledEnum"=T2."Disabled and Grayed Out" ("Disabled")) -> ()  [unwired: 2 in, 2 out]
          }
          frame #2 {
            n946 = property on="X Go" class="Bool"("DisabledEnum"=T2."Disabled and Grayed Out" ("Disabled")) -> ()  [unwired: 2 in, 2 out]
          }
        }
      }
      event #17 {
        n947 = event-data() -> ()  [unwired: 1 in, 7 out]
        n948 = flat-sequence {
          tunnel: w1540 -> [w1552]
          tunnel: w1539 -> [w1553]
          tunnel: [w1543] -> w1537
          tunnel: [w1559] -> w1536
          tunnel: w1537 -> [w1566]
          tunnel: w1536 -> [w1565]
          tunnel: [w1566] -> w1534
          tunnel: [w1565] -> w1533
          tunnel: [w1568] -> w1538
          tunnel: [w1569] -> w1535
          tunnel: w1534 -> [w1569]
          tunnel: w1533 -> [w1568]
          frame #0 {
            # "VELOCITY"
            n949 = property on="Y Scan Velocity SP steps/sec" class="DigNum (strict)"() -> ("Value"=w1555:i32)  [unwired: 2 in, 2 out]
            n950 = property on="Y steps/rev" class="DigNum (strict)"() -> ("Value"=w1546:u32)  [unwired: 2 in, 2 out]
            n951 = Divide(x=w1555, y=w1546) -> (x/y=w1556:dbl)
            n952 = Number To Fractional String(number=w1556) -> (F-format string=w1557:string)  [unwired: 3 in]
            n953 = call "Applied Send Command.vi"("error in (no error)"=w1552, "Extra"=w1557, "Command"=T1."Velocity Setting", "VISA resource name"=w1553) -> ("error out"=w1554:errorcluster, "VISA resource name out"=w1544:refnum<visa-resource-name>)  [unwired: 3 in, 1 out]
            n954 = call "Time Delay5"("error in (no error)"=w1554) -> ("error out"=w1545:errorcluster)  [unwired: 10 in]
            n955 = call "Applied Send Command.vi"("error in (no error)"=w1545, "Extra"="", "Command"=T1."Velocity Setting", "VISA resource name"=w1544) -> ("error out"=w1542:errorcluster, "read buffer"=w1549:string, "VISA resource name out"=w1543:refnum<visa-resource-name>)  [unwired: 3 in]
            n956 = Fract/Exp String To Number(string=w1549, offset=3) -> (number=w1548:dbl)  [unwired: 2 in, 1 out]
            n957 = call "Time Delay6"("error in (no error)"=w1542) -> ("error out"=w1559:errorcluster)  [unwired: 10 in]
            n958 = Multiply(x=w1548, y=w1546) -> (x*y=w1547:dbl)
            n959 = property on="Y velocity PV step/sec" class="DigNum (strict)"("Val(Sgnl)"=w1547) -> ()  [unwired: 2 in, 2 out]
          }
          frame #1 {
            n960 = property on="Y Scan" class="Bool (strict)"("Val(Sgnl)"=TRUE ("Slew Ready 2")) -> ()  [unwired: 2 in, 2 out]
            n961 = property on="Scan Cancel" class="Bool"("DisabledEnum"=T2."Enabled" ("Disabled")) -> ()  [unwired: 2 in, 2 out]
            n962 = property on="Scan Go" class="Bool"("DisabledEnum"=T2."Enabled" ("Disabled")) -> ()  [unwired: 2 in, 2 out]
            n963 = property on="Y Scan Length SP steps" class="DigNum (strict)"("DisabledEnum"=T2."Disabled and Grayed Out" ("Disabled")) -> ()  [unwired: 2 in, 2 out]
            n964 = property on="Y Scan Velocity SP steps/sec" class="DigNum (strict)"("DisabledEnum"=T2."Disabled and Grayed Out" ("Disabled")) -> ()  [unwired: 2 in, 2 out]
          }
          frame #2 {
            n965 = property on="Y Go" class="Bool"("DisabledEnum"=T2."Disabled and Grayed Out" ("Disabled")) -> ()  [unwired: 2 in, 2 out]
          }
        }
      }
      event #18 {
        n966 = event-data() -> ()  [unwired: 1 in, 7 out]
        n967 = flat-sequence {
          tunnel: [w1582] -> w1577
          tunnel: [w1596] -> w1576
          tunnel: w1573 -> [w1578]
          tunnel: w1572 -> [w1579]
          tunnel: w1577 -> [w1603]
          tunnel: w1576 -> [w1602]
          tunnel: [w1603] -> w1575
          tunnel: [w1602] -> w1574
          tunnel: [w1605] -> w1571
          tunnel: [w1606] -> w1570
          tunnel: w1575 -> [w1606]
          tunnel: w1574 -> [w1605]
          frame #0 {
            # "VELOCITY"
            n968 = property on="Z Scan Velocity SP steps/sec" class="DigNum (strict)"() -> ("Value"=w1592:i32)  [unwired: 2 in, 2 out]
            n969 = property on="Z steps/rev" class="DigNum (strict)"() -> ("Value"=w1585:u32)  [unwired: 2 in, 2 out]
            n970 = Divide(x=w1592, y=w1585) -> (x/y=w1593:dbl)
            n971 = Number To Fractional String(number=w1593) -> (F-format string=w1594:string)  [unwired: 3 in]
            n972 = call "Applied Send Command.vi"("error in (no error)"=w1579, "Extra"=w1594, "Command"=T1."Velocity Setting", "VISA resource name"=w1578) -> ("error out"=w1591:errorcluster, "VISA resource name out"=w1581:refnum<visa-resource-name>)  [unwired: 3 in, 1 out]
            n973 = call "Time Delay24"("error in (no error)"=w1591) -> ("error out"=w1580:errorcluster)  [unwired: 10 in]
            n974 = call "Applied Send Command.vi"("error in (no error)"=w1580, "Extra"="", "Command"=T1."Velocity Setting", "VISA resource name"=w1581) -> ("error out"=w1583:errorcluster, "read buffer"=w1588:string, "VISA resource name out"=w1582:refnum<visa-resource-name>)  [unwired: 3 in]
            n975 = call "Time Delay25"("error in (no error)"=w1583) -> ("error out"=w1596:errorcluster)  [unwired: 10 in]
            n976 = Fract/Exp String To Number(string=w1588, offset=3) -> (number=w1587:dbl)  [unwired: 2 in, 1 out]
            n977 = Multiply(x=w1587, y=w1585) -> (x*y=w1584:dbl)
            n978 = property on="Z  velocity PV step/sec" class="DigNum (strict)"("Val(Sgnl)"=w1584) -> ()  [unwired: 2 in, 2 out]
          }
          frame #1 {
            n979 = property on="Z Scan" class="Bool (strict)"("Val(Sgnl)"=TRUE ("Slew Ready 2")) -> ()  [unwired: 2 in, 2 out]
            n980 = property on="Scan Cancel" class="Bool"("DisabledEnum"=T2."Enabled" ("Disabled")) -> ()  [unwired: 2 in, 2 out]
            n981 = property on="Scan Go" class="Bool"("DisabledEnum"=T2."Enabled" ("Disabled")) -> ()  [unwired: 2 in, 2 out]
            n982 = property on="Z Scan Length SP steps" class="DigNum (strict)"("DisabledEnum"=T2."Disabled and Grayed Out" ("Disabled")) -> ()  [unwired: 2 in, 2 out]
            n983 = property on="Z Scan Velocity SP steps/sec" class="DigNum (strict)"("DisabledEnum"=T2."Disabled and Grayed Out" ("Disabled")) -> ()  [unwired: 2 in, 2 out]
          }
          frame #2 {
            n984 = property on="Z Go" class="Bool"("DisabledEnum"=T2."Disabled and Grayed Out" ("Disabled")) -> ()  [unwired: 2 in, 2 out]
          }
        }
      }
      event #19 {
        n985 = event-data() -> ()  [unwired: 1 in, 7 out]
        n986 = flat-sequence {
          tunnel: [w1618] -> w1614
          tunnel: [w1633] -> w1613
          tunnel: w1610 -> [w1626]
          tunnel: w1609 -> [w1627]
          tunnel: w1614 -> [w1640]
          tunnel: w1613 -> [w1639]
          tunnel: [w1640] -> w1612
          tunnel: [w1639] -> w1611
          tunnel: [w1642] -> w1607
          tunnel: [w1643] -> w1608
          tunnel: w1612 -> [w1643]
          tunnel: w1611 -> [w1642]
          frame #0 {
            # "VELOCITY"
            n987 = property on="R Scan Velocity SP steps/sec" class="DigNum (strict)"() -> ("Value"=w1628:i32)  [unwired: 2 in, 2 out]
            n988 = property on="R steps/rev" class="DigNum (strict)"() -> ("Value"=w1616:u32)  [unwired: 2 in, 2 out]
            n989 = Divide(x=w1628, y=w1616) -> (x/y=w1630:dbl)
            n990 = Number To Fractional String(number=w1630) -> (F-format string=w1631:string)  [unwired: 3 in]
            n991 = call "Applied Send Command.vi"("error in (no error)"=w1627, "Extra"=w1631, "Command"=T1."Velocity Setting", "VISA resource name"=w1626) -> ("error out"=w1629:errorcluster, "VISA resource name out"=w1620:refnum<visa-resource-name>)  [unwired: 3 in, 1 out]
            n992 = call "Time Delay26"("error in (no error)"=w1629) -> ("error out"=w1619:errorcluster)  [unwired: 10 in]
            n993 = call "Applied Send Command.vi"("error in (no error)"=w1619, "Extra"="", "Command"=T1."Velocity Setting", "VISA resource name"=w1620) -> ("error out"=w1617:errorcluster, "read buffer"=w1623:string, "VISA resource name out"=w1618:refnum<visa-resource-name>)  [unwired: 3 in]
            n994 = call "Time Delay27"("error in (no error)"=w1617) -> ("error out"=w1633:errorcluster)  [unwired: 10 in]
            n995 = Fract/Exp String To Number(string=w1623, offset=3) -> (number=w1622:dbl)  [unwired: 2 in, 1 out]
            n996 = Multiply(x=w1622, y=w1616) -> (x*y=w1615:dbl)
            n997 = property on="R velocity PV step/sec" class="DigNum (strict)"("Val(Sgnl)"=w1615) -> ()  [unwired: 2 in, 2 out]
          }
          frame #1 {
            n998 = property on="R Scan" class="Bool (strict)"("Val(Sgnl)"=TRUE ("Slew Ready 2")) -> ()  [unwired: 2 in, 2 out]
            n999 = property on="Scan Cancel" class="Bool"("DisabledEnum"=T2."Enabled" ("Disabled")) -> ()  [unwired: 2 in, 2 out]
            n1000 = property on="Scan Go" class="Bool"("DisabledEnum"=T2."Enabled" ("Disabled")) -> ()  [unwired: 2 in, 2 out]
            n1001 = property on="R Scan Length SP steps" class="DigNum (strict)"("DisabledEnum"=T2."Disabled and Grayed Out" ("Disabled")) -> ()  [unwired: 2 in, 2 out]
            n1002 = property on="R Scan Velocity SP steps/sec" class="DigNum (strict)"("DisabledEnum"=T2."Disabled and Grayed Out" ("Disabled")) -> ()  [unwired: 2 in, 2 out]
          }
          frame #2 {
            n1003 = property on="R Go" class="Bool"("DisabledEnum"=T2."Disabled and Grayed Out" ("Disabled")) -> ()  [unwired: 2 in, 2 out]
          }
        }
      }
      event #20 {
        n1004 = event-data() -> ()  [unwired: 1 in, 4 out]
        n1005 = event-data() -> ()  [unwired: 3 in, 1 out]
      }
      event #21 {
        n1006 = event-data() -> ()  [unwired: 1 in, 7 out]
        n1007 = flat-sequence {
          tunnel: [w1674] -> w1657
          tunnel: [w1673] -> w1656
          tunnel: w1655 -> [w1675]
          tunnel: w1654 -> [w1672]
          frame #0 {
            n1008 = call "Applied Send Command.vi"("error in (no error)"=w1672, "Command"=T1."Stop", "VISA resource name"=w1675) -> ("error out"=w1673:errorcluster, "VISA resource name out"=w1674:refnum<visa-resource-name>)  [unwired: 4 in, 1 out]
          }
        }
        n1009 = flat-sequence {
          tunnel: w1661 -> [w1678]
          tunnel: w1660 -> [w1677]
          tunnel: [w1679] -> w1659
          tunnel: [w1680] -> w1658
          frame #0 {
            n1010 = call "Applied Send Command.vi"("error in (no error)"=w1677, "Command"=T1."Stop", "VISA resource name"=w1678) -> ("error out"=w1680:errorcluster, "VISA resource name out"=w1679:refnum<visa-resource-name>)  [unwired: 4 in, 1 out]
          }
        }
        n1011 = flat-sequence {
          tunnel: [w1669] -> w1651
          tunnel: [w1670] -> w1650
          tunnel: w1653 -> [w1667]
          tunnel: w1652 -> [w1668]
          frame #0 {
            n1012 = call "Applied Send Command.vi"("error in (no error)"=w1668, "Command"=T1."Stop", "VISA resource name"=w1667) -> ("error out"=w1670:errorcluster, "VISA resource name out"=w1669:refnum<visa-resource-name>)  [unwired: 4 in, 1 out]
          }
        }
        n1013 = flat-sequence {
          tunnel: w1649 -> [w1662]
          tunnel: w1648 -> [w1663]
          tunnel: [w1665] -> w1647
          tunnel: [w1664] -> w1646
          frame #0 {
            n1014 = call "Applied Send Command.vi"("error in (no error)"=w1663, "Command"=T1."Stop", "VISA resource name"=w1662) -> ("error out"=w1664:errorcluster, "VISA resource name out"=w1665:refnum<visa-resource-name>)  [unwired: 4 in, 1 out]
          }
        }
      }
      event #22 {
        n1015 = event-data() -> ()  [unwired: 1 in, 7 out]
        n1016 = flat-sequence {
          tunnel: w1697 -> [w1735]
          tunnel: w1696 -> [w1734]
          tunnel: [w1737] -> w1699
          tunnel: [w1736] -> w1698
          tunnel: [w1745] -> w1694
          tunnel: [w1746] -> w1695
          tunnel: w1699 -> [w1746]
          tunnel: w1698 -> [w1745]
          frame #0 {
            n1017 = call "Applied Send Command.vi"("error in (no error)"=w1734, "Command"=T1."Stop", "VISA resource name"=w1735) -> ("error out"=w1736:errorcluster, "VISA resource name out"=w1737:refnum<visa-resource-name>)  [unwired: 4 in, 1 out]
          }
          frame #1 {
            n1018 = property on="X Scan" class="Bool (strict)"("Value"=FALSE ("Slew Ready")) -> ()  [unwired: 2 in, 2 out]
            n1019 = property on="X Scan set" class="Bool"("DisabledEnum"=T2."Enabled" ("Disabled")) -> ()  [unwired: 2 in, 2 out]
            n1020 = property on="X Scan Velocity SP steps/sec" class="DigNum (strict)"("DisabledEnum"=T2."Enabled" ("Disabled")) -> ()  [unwired: 2 in, 2 out]
            n1021 = property on="X Scan Length SP steps" class="DigNum (strict)"("DisabledEnum"=T2."Enabled" ("Disabled")) -> ()  [unwired: 2 in, 2 out]
            n1022 = property on="X Go" class="Bool"("DisabledEnum"=T2."Enabled" ("Disabled")) -> ()  [unwired: 2 in, 2 out]
            n1023 = property on="X Scan OK" class="Bool"("DisabledEnum"=T2."Enabled" ("Disabled")) -> ()  [unwired: 2 in, 2 out]
          }
        }
        n1024 = flat-sequence {
          tunnel: w1705 -> [w1748]
          tunnel: w1704 -> [w1747]
          tunnel: [w1750] -> w1701
          tunnel: [w1749] -> w1700
          tunnel: [w1758] -> w1706
          tunnel: [w1759] -> w1707
          tunnel: w1701 -> [w1759]
          tunnel: w1700 -> [w1758]
          frame #0 {
            n1025 = call "Applied Send Command.vi"("error in (no error)"=w1747, "Command"=T1."Stop", "VISA resource name"=w1748) -> ("error out"=w1749:errorcluster, "VISA resource name out"=w1750:refnum<visa-resource-name>)  [unwired: 4 in, 1 out]
          }
          frame #1 {
            n1026 = property on="Y Scan" class="Bool (strict)"("Value"=FALSE ("Slew Ready")) -> ()  [unwired: 2 in, 2 out]
            n1027 = property on="Y Go" class="Bool"("DisabledEnum"=T2."Enabled" ("Disabled")) -> ()  [unwired: 2 in, 2 out]
            n1028 = property on="Y Scan Velocity SP steps/sec" class="DigNum (strict)"("DisabledEnum"=T2."Enabled" ("Disabled")) -> ()  [unwired: 2 in, 2 out]
            n1029 = property on="Y Scan set" class="Bool"("DisabledEnum"=T2."Enabled" ("Disabled")) -> ()  [unwired: 2 in, 2 out]
            n1030 = property on="Y Scan OK" class="Bool"("DisabledEnum"=T2."Enabled" ("Disabled")) -> ()  [unwired: 2 in, 2 out]
            n1031 = property on="Y Scan Length SP steps" class="DigNum (strict)"("DisabledEnum"=T2."Enabled" ("Disabled")) -> ()  [unwired: 2 in, 2 out]
          }
        }
        n1032 = flat-sequence {
          tunnel: [w1724] -> w1693
          tunnel: [w1723] -> w1692
          tunnel: w1691 -> [w1722]
          tunnel: w1690 -> [w1721]
          tunnel: [w1732] -> w1688
          tunnel: [w1733] -> w1689
          tunnel: w1693 -> [w1733]
          tunnel: w1692 -> [w1732]
          frame #0 {
            n1033 = call "Applied Send Command.vi"("error in (no error)"=w1721, "Command"=T1."Stop", "VISA resource name"=w1722) -> ("error out"=w1723:errorcluster, "VISA resource name out"=w1724:refnum<visa-resource-name>)  [unwired: 4 in, 1 out]
          }
          frame #1 {
            n1034 = property on="Z Scan" class="Bool (strict)"("Value"=FALSE ("Slew Ready")) -> ()  [unwired: 2 in, 2 out]
            n1035 = property on="Z Scan set" class="Bool"("DisabledEnum"=T2."Enabled" ("Disabled")) -> ()  [unwired: 2 in, 2 out]
            n1036 = property on="Z Scan Velocity SP steps/sec" class="DigNum (strict)"("DisabledEnum"=T2."Enabled" ("Disabled")) -> ()  [unwired: 2 in, 2 out]
            n1037 = property on="Z Scan Length SP steps" class="DigNum (strict)"("DisabledEnum"=T2."Enabled" ("Disabled")) -> ()  [unwired: 2 in, 2 out]
            n1038 = property on="Z Go" class="Bool"("DisabledEnum"=T2."Enabled" ("Disabled")) -> ()  [unwired: 2 in, 2 out]
            n1039 = property on="Z Scan OK" class="Bool"("DisabledEnum"=T2."Enabled" ("Disabled")) -> ()  [unwired: 2 in, 2 out]
          }
        }
        n1040 = flat-sequence {
          tunnel: [w1711] -> w1687
          tunnel: [w1710] -> w1686
          tunnel: w1685 -> [w1708]
          tunnel: w1684 -> [w1709]
          tunnel: [w1719] -> w1682
          tunnel: [w1720] -> w1683
          tunnel: w1687 -> [w1720]
          tunnel: w1686 -> [w1719]
          frame #0 {
            n1041 = call "Applied Send Command.vi"("error in (no error)"=w1709, "Command"=T1."Stop", "VISA resource name"=w1708) -> ("error out"=w1710:errorcluster, "VISA resource name out"=w1711:refnum<visa-resource-name>)  [unwired: 4 in, 1 out]
          }
          frame #1 {
            n1042 = property on="R Scan" class="Bool (strict)"("Value"=FALSE ("Slew Ready")) -> ()  [unwired: 2 in, 2 out]
            n1043 = property on="R Scan Velocity SP steps/sec" class="DigNum (strict)"("DisabledEnum"=T2."Enabled" ("Disabled")) -> ()  [unwired: 2 in, 2 out]
            n1044 = property on="R Go" class="Bool"("DisabledEnum"=T2."Enabled" ("Disabled")) -> ()  [unwired: 2 in, 2 out]
            n1045 = property on="R Scan OK" class="Bool"("DisabledEnum"=T2."Enabled" ("Disabled")) -> ()  [unwired: 2 in, 2 out]
            n1046 = property on="R Scan Length SP steps" class="DigNum (strict)"("DisabledEnum"=T2."Enabled" ("Disabled")) -> ()  [unwired: 2 in, 2 out]
            n1047 = property on="R Scan set" class="Bool"("DisabledEnum"=T2."Enabled" ("Disabled")) -> ()  [unwired: 2 in, 2 out]
          }
        }
        n1048 = property on="Scan Go" class="Bool"("DisabledEnum"=T2."Disabled and Grayed Out" ("Disabled")) -> ()  [unwired: 2 in, 2 out]
        n1049 = property on="Scan Cancel" class="Bool"("DisabledEnum"=T2."Disabled and Grayed Out" ("Disabled")) -> ()  [unwired: 2 in, 2 out]
      }
      event #23 {
        n1050 = event-data() -> ()  [unwired: 1 in, 7 out]
        n1051 = flat-sequence {
          tunnel: w1795 -> [w1814]
          tunnel: w1794 -> [w1815]
          tunnel: w1793 -> [w1812]
          tunnel: w1792 -> [w1813]
          tunnel: w1791 -> [w1811]
          tunnel: w1790 -> [w1810]
          tunnel: w1789 -> [w1809]
          tunnel: w1788 -> [w1808]
          tunnel: [w1807] -> w1779
          tunnel: [w1806] -> w1777
          tunnel: [w1805] -> w1775
          tunnel: [w1804] -> w1773
          tunnel: [w1803] -> w1771
          tunnel: [w1802] -> w1769
          tunnel: [w1801] -> w1767
          tunnel: [w1800] -> w1765
          tunnel: [w1799] -> w1763
          tunnel: [w1798] -> w1762
          tunnel: [w1797] -> w1761
          tunnel: [w1796] -> w1760
          tunnel: w1779 -> [w1871]
          tunnel: [w1870] -> w1778
          tunnel: w1777 -> [w1869]
          tunnel: [w1868] -> w1776
          tunnel: w1775 -> [w1867]
          tunnel: [w1866] -> w1774
          tunnel: w1773 -> [w1865]
          tunnel: [w1864] -> w1772
          tunnel: w1771 -> [w1863]
          tunnel: [w1862] -> w1770
          tunnel: w1769 -> [w1860]
          tunnel: [w1861] -> w1768
          tunnel: w1767 -> [w1859]
          tunnel: [w1858] -> w1766
          tunnel: w1765 -> [w1857]
          tunnel: [w1856] -> w1764
          tunnel: w1763 -> [w1855]
          tunnel: w1762 -> [w1854]
          tunnel: w1761 -> [w1853]
          tunnel: w1760 -> [w1852]
          tunnel: [w1906] -> w1787
          tunnel: [w1905] -> w1786
          tunnel: [w1904] -> w1785
          tunnel: [w1903] -> w1784
          tunnel: [w1902] -> w1783
          tunnel: [w1901] -> w1782
          tunnel: [w1908] -> w1781
          tunnel: [w1907] -> w1780
          tunnel: w1778 -> [w1908]
          tunnel: w1776 -> [w1907]
          tunnel: w1774 -> [w1906]
          tunnel: w1772 -> [w1905]
          tunnel: w1770 -> [w1904]
          tunnel: w1768 -> [w1903]
          tunnel: w1766 -> [w1902]
          tunnel: w1764 -> [w1901]
          frame #0 {
            n1052 = property on="X Scan" class="Bool (strict)"() -> ("Value"=w1796:bool)  [unwired: 2 in, 2 out]
            n1053 = property on="Y Scan" class="Bool (strict)"() -> ("Value"=w1797:bool)  [unwired: 2 in, 2 out]
            n1054 = property on="Z Scan" class="Bool (strict)"() -> ("Value"=w1798:bool)  [unwired: 2 in, 2 out]
            n1055 = property on="R Scan" class="Bool (strict)"() -> ("Value"=w1799:bool)  [unwired: 2 in, 2 out]
            n1056 = case shown="True" w1796 {
              tunnel: w1815 -> [w1835 w1839]
              tunnel: [w1835 w1838] -> w1806
              tunnel: w1814 -> [w1834 w1837]
              tunnel: [w1834 w1836] -> w1807
              frame #0 {
              }
              frame #1 {
                n1057 = property on="X Scan Length SP steps" class="DigNum (strict)"() -> ("Value"=w1840:i32)  [unwired: 2 in, 2 out]
                n1058 = Number To Decimal String(number=w1840) -> (decimal integer string=w1841:string)  [unwired: 1 in]
                n1059 = call "Applied Send Command.vi"("error in (no error)"=w1839, "Extra"=w1841, "Command"=T1."Distance or Position", "VISA resource name"=w1837) -> ("error out"=w1838:errorcluster, "VISA resource name out"=w1836:refnum<visa-resource-name>)  [unwired: 3 in, 1 out]
              }
            }
            n1060 = case shown="True" w1797 {
              tunnel: w1812 -> [w1844 w1849]
              tunnel: w1813 -> [w1843 w1848]
              tunnel: [w1843 w1845] -> w1804
              tunnel: [w1844 w1846] -> w1805
              frame #0 {
              }
              frame #1 {
                n1061 = property on="Y Scan Length SP steps" class="DigNum (strict)"() -> ("Value"=w1847:i32)  [unwired: 2 in, 2 out]
                n1062 = Number To Decimal String(number=w1847) -> (decimal integer string=w1850:string)  [unwired: 1 in]
                n1063 = call "Applied Send Command.vi"("error in (no error)"=w1848, "Extra"=w1850, "Command"=T1."Distance or Position", "VISA resource name"=w1849) -> ("error out"=w1845:errorcluster, "VISA resource name out"=w1846:refnum<visa-resource-name>)  [unwired: 3 in, 1 out]
              }
            }
            n1064 = case shown="True" w1798 {
              tunnel: w1811 -> [w1826 w1830]
              tunnel: [w1826 w1829] -> w1803
              tunnel: [w1825 w1828] -> w1802
              tunnel: w1810 -> [w1825 w1827]
              frame #0 {
              }
              frame #1 {
                n1065 = property on="Z Scan Length SP steps" class="DigNum (strict)"() -> ("Value"=w1831:i32)  [unwired: 2 in, 2 out]
                n1066 = Number To Decimal String(number=w1831) -> (decimal integer string=w1832:string)  [unwired: 1 in]
                n1067 = call "Applied Send Command.vi"("error in (no error)"=w1827, "Extra"=w1832, "Command"=T1."Distance or Position", "VISA resource name"=w1830) -> ("error out"=w1828:errorcluster, "VISA resource name out"=w1829:refnum<visa-resource-name>)  [unwired: 3 in, 1 out]
              }
            }
            n1068 = case shown="True" w1799 {
              tunnel: w1809 -> [w1817 w1822]
              tunnel: [w1817 w1821] -> w1801
              tunnel: w1808 -> [w1816 w1820]
              tunnel: [w1816 w1819] -> w1800
              frame #0 {
              }
              frame #1 {
                n1069 = property on="R Scan Length SP steps" class="DigNum (strict)"() -> ("Value"=w1818:i32)  [unwired: 2 in, 2 out]
                n1070 = Number To Decimal String(number=w1818) -> (decimal integer string=w1823:string)  [unwired: 1 in]
                n1071 = call "Applied Send Command.vi"("error in (no error)"=w1820, "Extra"=w1823, "Command"=T1."Distance or Position", "VISA resource name"=w1822) -> ("error out"=w1819:errorcluster, "VISA resource name out"=w1821:refnum<visa-resource-name>)  [unwired: 3 in, 1 out]
              }
            }
          }
          frame #1 {
            n1072 = case shown="True" w1852 {
              tunnel: w1871 -> [w1894 w1898]
              tunnel: [w1894 w1897] -> w1870
              tunnel: w1869 -> [w1893 w1896]
              tunnel: [w1893 w1895] -> w1868
              frame #0 {
              }
              frame #1 {
                n1073 = call "Applied Send Command.vi"("error in (no error)"=w1896, "Command"=T1."Feed to Length", "VISA resource name"=w1898) -> ("error out"=w1895:errorcluster, "VISA resource name out"=w1897:refnum<visa-resource-name>)  [unwired: 4 in, 1 out]
              }
            }
            n1074 = case shown="True" w1853 {
              tunnel: w1867 -> [w1887 w1891]
              tunnel: [w1887 w1890] -> w1866
              tunnel: w1865 -> [w1886 w1889]
              tunnel: [w1886 w1888] -> w1864
              frame #0 {
              }
              frame #1 {
                n1075 = call "Applied Send Command.vi"("error in (no error)"=w1889, "Command"=T1."Feed to Length", "VISA resource name"=w1891) -> ("error out"=w1888:errorcluster, "VISA resource name out"=w1890:refnum<visa-resource-name>)  [unwired: 4 in, 1 out]
              }
            }
            n1076 = case shown="False" w1854 {
              tunnel: w1863 -> [w1880 w1884]
              tunnel: [w1880 w1883] -> w1862
              tunnel: [w1879 w1882] -> w1861
              tunnel: w1860 -> [w1879 w1881]
              frame #0 {
              }
              frame #1 {
                n1077 = call "Applied Send Command.vi"("error in (no error)"=w1881, "Command"=T1."Feed to Length", "VISA resource name"=w1884) -> ("error out"=w1882:errorcluster, "VISA resource name out"=w1883:refnum<visa-resource-name>)  [unwired: 4 in, 1 out]
              }
            }
            n1078 = case shown="False" w1855 {
              tunnel: w1859 -> [w1873 w1877]
              tunnel: [w1873 w1876] -> w1858
              tunnel: w1857 -> [w1872 w1875]
              tunnel: [w1872 w1874] -> w1856
              frame #0 {
              }
              frame #1 {
                n1079 = call "Applied Send Command.vi"("error in (no error)"=w1875, "Command"=T1."Feed to Length", "VISA resource name"=w1877) -> ("error out"=w1874:errorcluster, "VISA resource name out"=w1876:refnum<visa-resource-name>)  [unwired: 4 in, 1 out]
              }
            }
          }
          frame #2 {
            n1080 = call "Time Delay7"("Delay Time (s)"=0.1) -> ()  [unwired: 10 in, 1 out]
            n1081 = property on="R Scan" class="Bool (strict)"("Val(Sgnl)"=FALSE ("Slew Ready 2")) -> ()  [unwired: 2 in, 2 out]
            n1082 = property on="Z Scan" class="Bool (strict)"("Val(Sgnl)"=FALSE ("Slew Ready 2")) -> ()  [unwired: 2 in, 2 out]
            n1083 = property on="X Scan" class="Bool (strict)"("Val(Sgnl)"=FALSE ("Slew Ready 2")) -> ()  [unwired: 2 in, 2 out]
            n1084 = property on="Y Scan" class="Bool (strict)"("Val(Sgnl)"=FALSE ("Slew Ready 2")) -> ()  [unwired: 2 in, 2 out]
            n1085 = property on="Z Scan Velocity SP steps/sec" class="DigNum (strict)"("DisabledEnum"=T2."Enabled" ("Disabled")) -> ()  [unwired: 2 in, 2 out]
            n1086 = property on="X Scan Length SP steps" class="DigNum (strict)"("DisabledEnum"=T2."Enabled" ("Disabled")) -> ()  [unwired: 2 in, 2 out]
            n1087 = property on="Y Scan Selocity SP steps/sec" class="DigNum (strict)"("DisabledEnum"=T2."Enabled" ("Disabled")) -> ()  [unwired: 2 in, 2 out]
            n1088 = property on="Z Scan Length SP steps" class="DigNum (strict)"("DisabledEnum"=T2."Enabled" ("Disabled")) -> ()  [unwired: 2 in, 2 out]
            n1089 = property on="Y Scan Length SP steps" class="DigNum (strict)"("DisabledEnum"=T2."Enabled" ("Disabled")) -> ()  [unwired: 2 in, 2 out]
            n1090 = property on="X Scan Velocity SP steps/sec" class="DigNum (strict)"("DisabledEnum"=T2."Enabled" ("Disabled")) -> ()  [unwired: 2 in, 2 out]
            n1091 = property on="R Scan Velocity SP steps/sec" class="DigNum (strict)"("DisabledEnum"=T2."Enabled" ("Disabled")) -> ()  [unwired: 2 in, 2 out]
            n1092 = property on="R Scan Length SP steps" class="DigNum (strict)"("DisabledEnum"=T2."Enabled" ("Disabled")) -> ()  [unwired: 2 in, 2 out]
            n1093 = property on="Scan Go" class="Bool"("DisabledEnum"=T2."Disabled and Grayed Out" ("Disabled")) -> ()  [unwired: 2 in, 2 out]
            n1094 = property on="Scan Cancel" class="Bool"("DisabledEnum"=T2."Disabled and Grayed Out" ("Disabled")) -> ()  [unwired: 2 in, 2 out]
          }
        }
      }
      event #24 {
        n1095 = event-data() -> ()  [unwired: 1 in, 7 out]
        n1096 = flat-sequence {
          tunnel: [w1953] -> w1932
          tunnel: w1933 -> [w1955]
          tunnel: [w1954] -> w1931
          tunnel: w1934 -> [w1956]
          frame #0 {
            n1097 = property on="Reset X Motor Steps" class="DigNum (strict)"() -> ("Value"=w1959:i32)  [unwired: 2 in, 2 out]
            n1098 = Number To Decimal String(number=w1959) -> (decimal integer string=w1957:string)  [unwired: 1 in]
            n1099 = call "Applied Send Command.vi"("error in (no error)"=w1955, "Extra"=w1957, "Command"=T1."Set ABS Position", "VISA resource name"=w1956) -> ("error out"=w1954:errorcluster, "VISA resource name out"=w1953:refnum<visa-resource-name>)  [unwired: 3 in, 1 out]
          }
        }
        n1100 = flat-sequence {
          tunnel: w1938 -> [w1964]
          tunnel: w1937 -> [w1961]
          tunnel: [w1963] -> w1936
          tunnel: [w1962] -> w1935
          frame #0 {
            n1101 = property on="Reset Y Motor Steps" class="DigNum (strict)"() -> ("Value"=w1966:i32)  [unwired: 2 in, 2 out]
            n1102 = Number To Decimal String(number=w1966) -> (decimal integer string=w1965:string)  [unwired: 1 in]
            n1103 = call "Applied Send Command.vi"("error in (no error)"=w1961, "Extra"=w1965, "Command"=T1."Set ABS Position", "VISA resource name"=w1964) -> ("error out"=w1962:errorcluster, "VISA resource name out"=w1963:refnum<visa-resource-name>)  [unwired: 3 in, 1 out]
          }
        }
        n1104 = flat-sequence {
          tunnel: [w1944] -> w1926
          tunnel: [w1943] -> w1925
          tunnel: w1928 -> [w1942]
          tunnel: w1927 -> [w1941]
          frame #0 {
            n1105 = property on="Reset R Motor Steps" class="DigNum (strict)"() -> ("Value"=w1945:i32)  [unwired: 2 in, 2 out]
            n1106 = Number To Decimal String(number=w1945) -> (decimal integer string=w1940:string)  [unwired: 1 in]
            n1107 = call "Applied Send Command.vi"("error in (no error)"=w1941, "Extra"=w1940, "Command"=T1."Set ABS Position", "VISA resource name"=w1942) -> ("error out"=w1943:errorcluster, "VISA resource name out"=w1944:refnum<visa-resource-name>)  [unwired: 3 in, 1 out]
          }
        }
        n1108 = flat-sequence {
          tunnel: [w1951] -> w1924
          tunnel: [w1950] -> w1923
          tunnel: w1930 -> [w1948]
          tunnel: w1929 -> [w1949]
          frame #0 {
            n1109 = property on="Reset Z Motor Steps" class="DigNum (strict)"() -> ("Value"=w1952:i32)  [unwired: 2 in, 2 out]
            n1110 = Number To Decimal String(number=w1952) -> (decimal integer string=w1946:string)  [unwired: 1 in]
            n1111 = call "Applied Send Command.vi"("error in (no error)"=w1949, "Extra"=w1946, "Command"=T1."Set ABS Position", "VISA resource name"=w1948) -> ("error out"=w1950:errorcluster, "VISA resource name out"=w1951:refnum<visa-resource-name>)  [unwired: 3 in, 1 out]
          }
        }
      }
    }
    n1112 = case shown="True" "Delete Button" {
      tunnel: w377 -> [_ w402]
      frame #0 {
      }
      frame #1 {
        n1113 = property on="Preset positions" class="Ring (strict)"() -> ("Value"=w400:i32)  [unwired: 2 in, 2 out]
        n1114 = Delete From Array(array=w402, index=w400) -> (array with subset deleted=w401:string[])  [unwired: 1 in, 1 out]
        n1115 = property on="Presets" class="Arr (strict)"() -> ("Value"=w399:i32[][])  [unwired: 2 in, 2 out]
        n1116 = property on="Preset positions" class="Ring (strict)"("Strings []"=w401) -> ()  [unwired: 2 in, 2 out]
        n1117 = Delete From Array(array=w399, index (row)=w400) -> (array with subset deleted=w398:i32[][])  [unwired: 2 in, 1 out]
        n1118 = property on="Presets" class="Arr (strict)"("Val(Sgnl)"=w398) -> ()  [unwired: 2 in, 2 out]
      }
    }
    n1119 = case shown="True" "Set Button" {
      tunnel: "Preset positions" -> [_ w420]
      frame #0 {
      }
      frame #1 {
        n1120 = property on="Presets" class="Arr (strict)"() -> ("Value"=w417:i32[][])  [unwired: 2 in, 2 out]
        n1121 = Index Array(array=w417, index (row)=w420) -> (element=w419:i32[])  [unwired: 1 in]
        n1122 = Array To Cluster(array=w419) -> (cluster=w418:T4)
        n1123 = Unbundle(w418) -> ("Value[0]"=w416:i32, "Value[1]"=w415:i32, "Value[2]"=w414:i32, "Value[3]"=w413:i32)  [unwired: 5 out]
        n1124 = property on="X Step SP" class="DigNum (strict)"("Val(Sgnl)"=w416) -> ()  [unwired: 2 in, 2 out]
        n1125 = property on="Y Step SP" class="DigNum (strict)"("Val(Sgnl)"=w415) -> ()  [unwired: 2 in, 2 out]
        n1126 = property on="Z Step SP" class="DigNum (strict)"("Val(Sgnl)"=w414) -> ()  [unwired: 2 in, 2 out]
        n1127 = property on="R Step SP" class="DigNum (strict)"("Val(Sgnl)"=w413) -> ()  [unwired: 2 in, 2 out]
      }
    }
    n1128 = case shown="True" "Add Button" {
      tunnel: w377 -> [_ w412]
      frame #0 {
      }
      frame #1 {
        n1129 = property on="X Step PV" class="DigNum (strict)"() -> ("Value"=w407:i32)  [unwired: 2 in, 2 out]
        n1130 = property on="Y Step PV" class="DigNum (strict)"() -> ("Value"=w406:i32)  [unwired: 2 in, 2 out]
        n1131 = property on="Z Step PV" class="DigNum (strict)"() -> ("Value"=w405:i32)  [unwired: 2 in, 2 out]
        n1132 = property on="R Step PV" class="DigNum (strict)"() -> ("Value"=w404:i32)  [unwired: 2 in, 2 out]
        n1133 = Build Array(w407, w406, w405, w404) -> (w410:i32[])
        n1134 = Build Array (concatenate)(w412, "String") -> (w411:string[])
        n1135 = property on="Preset positions" class="Ring (strict)"("Strings []"=w411) -> ()  [unwired: 2 in, 2 out]
        n1136 = property on="Presets" class="Arr (strict)"() -> ("Value"=w409:i32[][])  [unwired: 2 in, 2 out]
        n1137 = Build Array (concatenate)(w409, w410) -> (w403:i32[][])
        n1138 = property on="Presets" class="Arr (strict)"("Val(Sgnl)"=w403) -> ()  [unwired: 2 in, 2 out]
      }
    }
  }
  n1139 = flat-sequence {
    tunnel: w70 -> [w1968]
    tunnel: w69 -> [w1967]
    tunnel: [w1979] -> w46
    frame #0 {
      # "GET CURRENT POSITION"
      n1140 = call "Applied Send Command.vi"("error in (no error)"=w1967, "Extra"="", "Command"=T1."Immediate Position?", "VISA resource name"=w1968) -> ("error out"=w1969:errorcluster, "read buffer"=w1974:string, "VISA resource name out"=w1970:refnum<visa-resource-name>)  [unwired: 3 in]
      n1141 = call "Applied Send Command.vi"("error in (no error)"=w1969, "Command"=T1."Stop & Kill Buffer", "VISA resource name"=w1970) -> ("error out"=w1976:errorcluster, "VISA resource name out"=w1977:refnum<visa-resource-name>)  [unwired: 4 in, 1 out]
      n1142 = Hexadecimal String To Number(string=w1974, offset=3) -> (number=w1971:u32)  [unwired: 1 in, 1 out]
      n1143 = VISA Close(VISA resource name=w1977, error in (no error)=w1976) -> ()  [unwired: 1 out]
      n1144 = To Long Integer(number=w1971) -> (32bit integer=w1979:i32)
    }
  }
  n1145 = flat-sequence {
    tunnel: w50 -> [w1982]
    tunnel: w49 -> [w1981]
    tunnel: [w1980] -> w45
    frame #0 {
      # "GET CURRENT POSITION"
      n1146 = call "Applied Send Command.vi"("error in (no error)"=w1981, "Extra"="", "Command"=T1."Immediate Position?", "VISA resource name"=w1982) -> ("error out"=w1983:errorcluster, "read buffer"=w1988:string, "VISA resource name out"=w1984:refnum<visa-resource-name>)  [unwired: 3 in]
      n1147 = call "Applied Send Command.vi"("error in (no error)"=w1983, "Command"=T1."Stop & Kill Buffer", "VISA resource name"=w1984) -> ("error out"=w1990:errorcluster, "VISA resource name out"=w1991:refnum<visa-resource-name>)  [unwired: 4 in, 1 out]
      n1148 = Hexadecimal String To Number(string=w1988, offset=3) -> (number=w1985:u32)  [unwired: 1 in, 1 out]
      n1149 = VISA Close(VISA resource name=w1991, error in (no error)=w1990) -> ()  [unwired: 1 out]
      n1150 = To Long Integer(number=w1985) -> (32bit integer=w1980:i32)
    }
  }
  n1151 = flat-sequence {
    tunnel: w52 -> [w1994]
    tunnel: w51 -> [w1993]
    tunnel: [w1995] -> w44
    frame #0 {
      # "GET CURRENT POSITION"
      n1152 = call "Applied Send Command.vi"("error in (no error)"=w1993, "Extra"="", "Command"=T1."Immediate Position?", "VISA resource name"=w1994) -> ("error out"=w1996:errorcluster, "read buffer"=w2001:string, "VISA resource name out"=w1997:refnum<visa-resource-name>)  [unwired: 3 in]
      n1153 = call "Applied Send Command.vi"("error in (no error)"=w1996, "Command"=T1."Stop & Kill Buffer", "VISA resource name"=w1997) -> ("error out"=w2003:errorcluster, "VISA resource name out"=w2004:refnum<visa-resource-name>)  [unwired: 4 in, 1 out]
      n1154 = Hexadecimal String To Number(string=w2001, offset=3) -> (number=w1998:u32)  [unwired: 1 in, 1 out]
      n1155 = VISA Close(VISA resource name=w2004, error in (no error)=w2003) -> ()  [unwired: 1 out]
      n1156 = To Long Integer(number=w1998) -> (32bit integer=w1995:i32)
    }
  }
  n1157 = flat-sequence {
    tunnel: w48 -> [w2007]
    tunnel: w47 -> [w2006]
    tunnel: [w2008] -> w43
    frame #0 {
      # "GET CURRENT POSITION"
      n1158 = call "Applied Send Command.vi"("error in (no error)"=w2006, "Extra"="", "Command"=T1."Immediate Position?", "VISA resource name"=w2007) -> ("error out"=w2009:errorcluster, "read buffer"=w2014:string, "VISA resource name out"=w2010:refnum<visa-resource-name>)  [unwired: 3 in]
      n1159 = call "Applied Send Command.vi"("error in (no error)"=w2009, "Command"=T1."Stop & Kill Buffer", "VISA resource name"=w2010) -> ("error out"=w2016:errorcluster, "VISA resource name out"=w2017:refnum<visa-resource-name>)  [unwired: 4 in, 1 out]
      n1160 = Hexadecimal String To Number(string=w2014, offset=3) -> (number=w2011:u32)  [unwired: 1 in, 1 out]
      n1161 = VISA Close(VISA resource name=w2017, error in (no error)=w2016) -> ()  [unwired: 1 out]
      n1162 = To Long Integer(number=w2011) -> (32bit integer=w2008:i32)
    }
  }
  n1163 = flat-sequence {
    tunnel: w46 -> [w2024]
    tunnel: w45 -> [w2023]
    tunnel: w44 -> [w2022]
    tunnel: w43 -> [w2021]
    frame #0 {
      n1164 = Build Array(w2024, w2023, w2022, w2021) -> (w2019:i32[])
      n1165 = call-poly <vilib>:"Write To Spreadsheet File.vi"("1D data"=w2019, "file path (dialog if empty)"=path "S:/LV codes/SCL2/POS.TXT") -> ()  [unwired: 6 in, 1 out]
    }
    frame #1 {
      n1166 = property on="Presets" class="Arr (strict)"() -> ("Value"=w2031:i32[][])  [unwired: 2 in, 2 out]
      n1167 = property on="Preset positions" class="Ring (strict)"() -> ("Strings []"=w2027:string[])  [unwired: 2 in, 2 out]
      n1168 = Number To Decimal String(number=w2031) -> (decimal integer string=w2025:string[][])  [unwired: 1 in]
      n1169 = Transpose 2D Array(2D array=w2025) -> (transposed array=w2026:string[][])
      n1170 = Build Array (concatenate)(w2027, w2026) -> (w2028:string[][])
      n1171 = Transpose 2D Array(2D array=w2028) -> (transposed array=w2029:string[][])
      n1172 = call-poly <vilib>:"Write To Spreadsheet File.vi"("2D data"=w2029, "file path (dialog if empty)"=path "S:/LV codes/SCL2/PRESET.TXT") -> ()  [unwired: 6 in, 1 out]
    }
  }
